vi "TC.vi"() -> ()   [LabVIEW 2013]
uses:
  lib/Lib.llb/CS.lvclass
  lib/Lib.llb/TCS.lvclass
  lib/Lib.llb/QCS.lvclass
  lib/Lib.llb/CS Emulation.lvclass
  lib/Lib.llb/PCS.lvclass
panel:
  out "TempStabilized":refnum<user-event>
  out "All I":dbl[](array[numeric])
  out "VI called?":bool=TRUE
  out "Error code":u8
  out "UpdateChannelInfo":refnum<user-event>
  out "zBridge set nr.":u8
  out "zDll":path=path "C:/Users/Sasha/Dropbox/Labview/LC Software/ImpSoft-V5.2.2-multithreaded/ImpBridgeLabview/ImpBridgeDll.dll"
  in  "String":string="^ Click the Run button to start the program "
  in  "Tab Control 6":enum32{"Page 1", "Page 2"}(tab)
  in  "Load config":bool
  in  "Start":bool
  in  "Load Data":bool
  in  "Pause":bool
  in  "Stop":bool
  in  "Minimize":bool
  in  "Copy to Clipboard":bool
  in  "Save to Cal Log":bool
  in  "Save config":bool
  in  "Save Data":bool
  in  "Clear all plots":bool
  in  "LogFileCreationTime":timestamp=timestamp(2742897600 s since 1904-01-01)
  out "UpdateLogFilePath":refnum<user-event>
  out "Calib path":path=path "C:/avs-47/aaaa"
  out "Log path":path
  out "TCS port":i32(ring)=3 items=["COM1", "COM2", "COM3", "COM4", "COM5", "COM6", "COM7", "COM8", "COM9", "PRN1", "PRN2", "PRN3", "PRN4"]
  out "UpdateCalibrations":refnum<user-event>
  out "AVS VISA session":refnum<visa-resource-name>="COM3"
  out "Current1flow":bool
  out "Current2flow":bool
  in  "Tab Control":enum32{"AVS"}(tab)
  in  "Channel Controls":T1(tab)=enum."All"
  out "T 01":dbl=nan caption="T" format="%#.3f mK"
  out "R 0":dbl caption="R" format="%.3p"
  out "R-Plot 0":cluster{dbl[], dbl[]}(graph) caption="R-Plot"
  in  "Log 0":bool caption="Log Y"
  out "T 02":dbl=nan caption="T" format="%#.3f mK"
  out "R 1":dbl caption="R" format="%.3p"
  out "R-Plot 1":cluster{dbl[], dbl[]}(graph) caption="R-Plot"
  in  "Log 1":bool caption="Log Y"
  out "T 03":dbl=nan caption="T" format="%#.3f mK"
  out "R 2":dbl caption="R" format="%.3p"
  out "R-Plot 2":cluster{dbl[], dbl[]}(graph) caption="R-Plot"
  in  "Log 2":bool caption="Log Y"
  out "T 04":dbl=nan caption="T" format="%#.3f mK"
  out "R 3":dbl caption="R" format="%.3p"
  out "R-Plot 3":cluster{dbl[], dbl[]}(graph) caption="R-Plot"
  in  "Log 3":bool caption="Log Y"
  out "T 05":dbl=nan caption="T" format="%#.3f mK"
  out "R 4":dbl caption="R" format="%.3p"
  out "R-Plot 4":cluster{dbl[], dbl[]}(graph) caption="R-Plot"
  in  "Log 4":bool caption="Log Y"
  out "T 06":dbl=nan caption="T" format="%#.3f mK"
  out "R 5":dbl caption="R" format="%.3p"
  out "R-Plot 5":cluster{dbl[], dbl[]}(graph) caption="R-Plot"
  in  "Log 5":bool caption="Log Y"
  out "T 07":dbl=nan caption="T" format="%#.3f mK"
  out "R 6":dbl caption="R" format="%.3p"
  out "R-Plot 6":cluster{dbl[], dbl[]}(graph) caption="R-Plot"
  in  "Log 6":bool caption="Log Y"
  out "T 08":dbl=nan caption="T" format="%#.3f mK"
  out "R 7":dbl caption="R" format="%.3p"
  out "R-Plot 7":cluster{dbl[], dbl[]}(graph) caption="R-Plot"
  in  "Log 7":bool caption="Log Y"
  out "T 9":dbl=nan caption="T" format="%#.3f mK"
  out "R 8":dbl caption="R" format="%.3p"
  out "R-Plot 8":cluster{dbl[], dbl[]}(graph) caption="R-Plot"
  in  "Log 8":bool caption="Log Y"
  out "T 10":dbl=nan caption="T" format="%#.3f mK"
  out "R 9":dbl caption="R" format="%.3p"
  out "R-Plot 9":cluster{dbl[], dbl[]}(graph) caption="R-Plot"
  in  "Log 9":bool caption="Log Y"
  out "T":T2 {"T0 3" format="%.2p"; "T0 2" format="%.2p"; "T0" format="%.2p"; "T0" format="%.2p"; "T0" format="%.2p"; "T0" format="%.2p"; "T0" format="%.2p"; "T0" format="%.2p"; "T0" format="%.2p"; "T0" format="%.2p"}
  in  "AVS names":T3={"AVS Name 0"="3K", "AVS Name 1"="Still", "AVS Name 2"="50 mK", "AVS Name 3"="MC", "AVS Name 4"="MC", "AVS Name 5"="", "AVS Name 6"="", "AVS Name 7"="", "AVS Name 8"="", "AVS Name 9"=""}
  in  "Edit Calibrations":T4
  in  "Thermometer":T5 {"Select sensor 10" items=["No Calibration.vi"]; "Select sensor 9" items=["No Calibration.vi"]; "Select sensor 8" items=["No Calibration.vi"]; "Select sensor 7" items=["No Calibration.vi"]; "Select sensor 6" items=["No Calibration.vi"]; "Select sensor 5" items=["No Calibration.vi"]; "Select sensor 4" items=["No Calibration.vi"]; "Select sensor 3" items=["No Calibration.vi"]; "Select sensor 2" items=["No Calibration.vi"]; "Select sensor 1" items=["No Calibration.vi"]}
  out "Units":T3
  out "R":T6={"R0"=0.0, "R1"=0.0, "R2"=-0.0, "R3"=0.0, "R4"=0.0, "R5"=0.0, "R6"=0.0, "R7"=0.0, "R6 2"=0.0, "R7 2"=0.0} {"R7 2" format="%.3p"; "R6 2" format="%.3p"; "R7" format="%.3p"; "R6" format="%.3p"; "R5" format="%.3p"; "R4" format="%.3p"; "R3" format="%.3p"; "R2" format="%.3p"; "R1" format="%.3p"; "R0" format="%.3p"}
  in  "Scan Parameters":enum32{"Page 1", "Page 2"}(tab)
  in  "Exc&Ranges":T7={"Excitationl 0"=4, "Excitationl 0"=4, "Excitationl 0"=3, "Excitationl 0"=3, "Excitationl 0"=3, "Excitationl 0"=3, "Excitationl 0"=3, "Excitationl 0"=3, "Range 0"=5, "Range 0"=5, "Range 0"=5, "Range 0"=5, "Range 0"=5, "Range 0"=5, "Range 0"=5, "Range 0"=5} {"Range 0" items=["n.a."=-1, "open"=0, "2 Ohm"=1, "20 Ohm"=2, "200 Ohm"=3, "2k Ohm"=4, "20k Ohm"=5, "200k Ohm"=6, "2M Ohm"=7]; "Range 0" items=["n.a."=-1, "open"=0, "2 Ohm"=1, "20 Ohm"=2, "200 Ohm"=3, "2k Ohm"=4, "20k Ohm"=5, "200k Ohm"=6, "2M Ohm"=7]; "Range 0" items=["n.a."=-1, "open"=0, "2 Ohm"=1, "20 Ohm"=2, "200 Ohm"=3, "2k Ohm"=4, "20k Ohm"=5, "200k Ohm"=6, "2M Ohm"=7]; "Range 0" items=["n.a."=-1, "open"=0, "2 Ohm"=1, "20 Ohm"=2, "200 Ohm"=3, "2k Ohm"=4, "20k Ohm"=5, "200k Ohm"=6, "2M Ohm"=7]; "Range 0" items=["n.a."=-1, "open"=0, "2 Ohm"=1, "20 Ohm"=2, "200 Ohm"=3, "2k Ohm"=4, "20k Ohm"=5, "200k Ohm"=6, "2M Ohm"=7]; "Range 0" items=["n.a."=-1, "open"=0, "2 Ohm"=1, "20 Ohm"=2, "200 Ohm"=3, "2k Ohm"=4, "20k Ohm"=5, "200k Ohm"=6, "2M Ohm"=7]; "Range 0" items=["n.a."=-1, "open"=0, "2 Ohm"=1, "20 Ohm"=2, "200 Ohm"=3, "2k Ohm"=4, "20k Ohm"=5, "200k Ohm"=6, "2M Ohm"=7]; "Range 0" items=["n.a."=-1, "open"=0, "2 Ohm"=1, "20 Ohm"=2, "200 Ohm"=3, "2k Ohm"=4, "20k Ohm"=5, "200k Ohm"=6, "2M Ohm"=7]; "Excitationl 0" items=["none", "3 µV", "10 µV", "30 µV", "100 µV", "300 µV", "1 mV", "3 mV"]; "Excitationl 0" items=["none", "3 µV", "10 µV", "30 µV", "100 µV", "300 µV", "1 mV", "3 mV"]; "Excitationl 0" items=["none", "3 µV", "10 µV", "30 µV", "100 µV", "300 µV", "1 mV", "3 mV"]; "Excitationl 0" items=["none", "3 µV", "10 µV", "30 µV", "100 µV", "300 µV", "1 mV", "3 mV"]; "Excitationl 0" items=["none", "3 µV", "10 µV", "30 µV", "100 µV", "300 µV", "1 mV", "3 mV"]; "Excitationl 0" items=["none", "3 µV", "10 µV", "30 µV", "100 µV", "300 µV", "1 mV", "3 mV"]; "Excitationl 0" items=["none", "3 µV", "10 µV", "30 µV", "100 µV", "300 µV", "1 mV", "3 mV"]; "Excitationl 0" items=["none", "3 µV", "10 µV", "30 µV", "100 µV", "300 µV", "1 mV", "3 mV"]}
  out "Status":T8
  out "zBridge params":T3
  out "uPlots":T9
  in  "Autorange":bool=TRUE
  out "Active":T10={"active Channel 0"=TRUE, "active Channel 1"=TRUE, "active Channel 2"=TRUE, "active Channel 3"=FALSE, "active Channel 4"=FALSE, "active Channel 5"=FALSE, "active Channel 6"=FALSE, "active Channel 7"=FALSE, "active Channel 8"=FALSE, "active Channel 9"=FALSE}
  out "SP":cluster{"Numeric":dbl, "R/T":dbl}(graph) caption="R-Plot 10"
  in  "HW Address":u32
  in  "Edit calibration":bool
  in  "Convert":bool
  out "T7":dbl caption="T=" format="%#.2p"
  in  "R7":dbl caption="R=" format="%_6g"
  in  "Select sensor 1":u16(ring) items=["No Calibration.vi"]
  out "I_list[i]":dbl[](array[numeric]) min=-1.0
  out "I 2":dbl[](array[numeric]) min=-1.0
  out "Revision":string="TC" caption="V"
  in  "Tab Control 5":enum32{"Page 1", "Page 2"}(tab)
  in  "Data History":enum32{"History", "Settings"}(tab)=enum."Settings"
  in  "Mode Buttons":T11(radio)
  in  "Clear plot":bool
  out "AVS names small":T3={"AVS Name 0"="3K", "AVS Name 1"="Still", "AVS Name 2"="50 mK", "AVS Name 3"="MC", "AVS Name 4"="MC", "AVS Name 5"="", "AVS Name 6"="", "AVS Name 7"="", "AVS Name 8"="", "AVS Name 9"=""}
  out "Time":dbl format="%<%X\n%x>T"
  out "Small T":dbl[](array[numeric]) caption="T" format="%.2p"
  out "Small R":dbl[](array[numeric]) caption="R" format="%.3p"
  in  "AVS Runtime Settings":T12={"Read AVS channels from"=0, "Last Channel"=4, "Delay Between Scans"=0, "Stabilisation Delay"=0.5, "Averages"=2, "Data Memory"=5000, "Filter graphs:"=FALSE, "Y_min"=0.0, "Y_max"=2000000.0, "Plot type"=enum."T vs Time", "Boolean"=FALSE, "Data Memory 2"=30.0} {"Data Memory 2" min=0.0; "Delay Between Scans" format="%.0f s"; "Averages" min=1 max=1000; "Stabilisation Delay" min=0.5; "Last Channel" min=0 max=9 step=1; "Read AVS channels from" min=0 max=7 step=1; "Y_max" format="%#_6f"; "Y_min" min=0.0 format="%#_6f"; "Data Memory" min=3 max=20000}
  out "I":dbl[](array[numeric])
  in  "Data":cluster{"R":dbl[], "T":dbl[], "Time":dbl[]}[](array[cluster])=[{"R"=[], "T"=[], "Time"=[]}, {"R"=[0.0, 2.0], "T"=[], "Time"=[]}]
  out "Int":dbl=10.0 format="%#.2f"
  out "T_array":dbl[](array[numeric])
  in  "Data array":dbl[](array[numeric])
  out "I3_SetPnt":dbl
  out "Currents changed":bool
  in  "Excitations":T13={"Excitationl 0"=4, "Excitation 1"=4, "Excitation 2"=3, "Excitation 3"=3, "Excitation 4"=3, "Excitation 5"=3, "Excitation 6"=3, "Excitation 7"=3} {"Excitation 7" items=["none", "3 µV", "10 µV", "30 µV", "100 µV", "300 µV", "1 mV", "3 mV"]; "Excitation 6" items=["none", "3 µV", "10 µV", "30 µV", "100 µV", "300 µV", "1 mV", "3 mV"]; "Excitation 5" items=["none", "3 µV", "10 µV", "30 µV", "100 µV", "300 µV", "1 mV", "3 mV"]; "Excitation 4" items=["none", "3 µV", "10 µV", "30 µV", "100 µV", "300 µV", "1 mV", "3 mV"]; "Excitation 3" items=["none", "3 µV", "10 µV", "30 µV", "100 µV", "300 µV", "1 mV", "3 mV"]; "Excitation 2" items=["none", "3 µV", "10 µV", "30 µV", "100 µV", "300 µV", "1 mV", "3 mV"]; "Excitation 1" items=["none", "3 µV", "10 µV", "30 µV", "100 µV", "300 µV", "1 mV", "3 mV"]; "Excitationl 0" items=["none", "3 µV", "10 µV", "30 µV", "100 µV", "300 µV", "1 mV", "3 mV"]}
  in  "Ranges":T13={"Excitationl 0"=5, "Excitation 1"=5, "Excitation 2"=5, "Excitation 3"=5, "Excitation 4"=5, "Excitation 5"=5, "Excitation 6"=5, "Excitation 7"=5} {"Excitation 7" items=["n.a."=-1, "open"=0, "2 Ohm"=1, "20 Ohm"=2, "200 Ohm"=3, "2k Ohm"=4, "20k Ohm"=5, "200k Ohm"=6, "2M Ohm"=7]; "Excitation 6" items=["n.a."=-1, "open"=0, "2 Ohm"=1, "20 Ohm"=2, "200 Ohm"=3, "2k Ohm"=4, "20k Ohm"=5, "200k Ohm"=6, "2M Ohm"=7]; "Excitation 5" items=["n.a."=-1, "open"=0, "2 Ohm"=1, "20 Ohm"=2, "200 Ohm"=3, "2k Ohm"=4, "20k Ohm"=5, "200k Ohm"=6, "2M Ohm"=7]; "Excitation 4" items=["n.a."=-1, "open"=0, "2 Ohm"=1, "20 Ohm"=2, "200 Ohm"=3, "2k Ohm"=4, "20k Ohm"=5, "200k Ohm"=6, "2M Ohm"=7]; "Excitation 3" items=["n.a."=-1, "open"=0, "2 Ohm"=1, "20 Ohm"=2, "200 Ohm"=3, "2k Ohm"=4, "20k Ohm"=5, "200k Ohm"=6, "2M Ohm"=7]; "Excitation 2" items=["n.a."=-1, "open"=0, "2 Ohm"=1, "20 Ohm"=2, "200 Ohm"=3, "2k Ohm"=4, "20k Ohm"=5, "200k Ohm"=6, "2M Ohm"=7]; "Excitation 1" items=["n.a."=-1, "open"=0, "2 Ohm"=1, "20 Ohm"=2, "200 Ohm"=3, "2k Ohm"=4, "20k Ohm"=5, "200k Ohm"=6, "2M Ohm"=7]; "Excitationl 0" items=["n.a."=-1, "open"=0, "2 Ohm"=1, "20 Ohm"=2, "200 Ohm"=3, "2k Ohm"=4, "20k Ohm"=5, "200k Ohm"=6, "2M Ohm"=7]}
  out "CS ref":refnum<class "CS.lvclass">
  out "start 2":bool
  in  "Tab Control 3":enum32{"Page 1", "Page 2"}(tab)
  out "Automatic mode 0":bool
  out "Automatic mode 1":bool
  out "Map Channel 0 to 2":T14(ring) caption="Output to"
  in  "uA 0":u32
  in  "CS Names":T15={"CS Name 0"="N.C.", "CS Name 1"="3K", "CS Name 2"="Still", "CS Name 3"="MC"}
  out "Ch0 -":T16={"uA"="000", "ON"=FALSE, "Gated"=FALSE, "current flows"=FALSE, "Error"=FALSE}
  in  "uA 3":u32
  in  "uA 2":u32
  in  "uA 1":u32
  out "Automatic mode 3":bool
  out "Automatic mode 2":bool
  out "Chn 3":T16={"uA"="000", "ON"=FALSE, "Gated"=FALSE, "current flows"=FALSE, "Error"=FALSE}
  out "Chn 2":T16={"uA"="000", "ON"=FALSE, "Gated"=FALSE, "current flows"=FALSE, "Error"=FALSE}
  out "Chn 1":T16={"uA"="000", "ON"=FALSE, "Gated"=FALSE, "current flows"=FALSE, "Error"=FALSE}
  out "I3":dbl=10.0
  out "vi reference":refnum<vi>
  in  "CS Ch3 mode":enum32{"Page 1", "Page 2"}(tab)=enum."Page 2"
  in  "T Sweep":T17={"Start value"=200.0, "End value"=250.0, "Step"=10.0, "Current"=0.0, "I_next"=FALSE, "I_prev"=FALSE, "Interrrupt Sweep"=FALSE, "Start"=FALSE, "Boolean"=TRUE} {"Step" min=0.0; "End value" min=0.0; "Start value" min=0.0}
  in  "Show PID graph?":bool
  out "I0":dbl format="%#.1f"
  out "CallExtVI":refnum<user-event>
  out "Unit":string
  out "UpdateValuesAVS":refnum<user-event>
  out "DoPID":refnum<user-event>
  out "UpdateValuesZBridge":refnum<user-event>
  out "zBridge params/Error":string
  out "CurCalibrations":T18
  out "LMB Down":bool
  out "T controlled":dbl
  out "ResetPIDloop":refnum<user-event>
  in  "Tab Control 2":T19(tab)
  in  "Parameters":bool
  out "ID":string
  out "Bridge status":errorcluster
  out "CS status":errorcluster
  out "General":errorcluster caption="General status"
  in  "Refresh Button":bool
  in  "Bridge settings":T20={"AVS type"=enum."AVS47A (GPIB interface)", "AVS_SPort"="COM5", "Address"="GPIB0::20::INSTR", "AVS_CalFolder"=path "E:/Dropbox/Labview/LC Software/All Calibrations"}
  in  "Current source settings":T21={"TCS_Port"="COM1", "TCS_Imax"=5, "CS type"=enum."TCS", "QCS/PCS Device"=0}
  in  "Data logging":T22={"AVS_Path"=path "C:/avs-47", "AVS_FName"="LogAVS", "CAL_FName"="calibration", "Filenames suffix"="_%Y-%m-%d-%H-%M-%S", "Delimeter"="\t", "NewFevery"=7, "Time Units"=enum."Days", "Date/Time Format"="%Y-%m-%d %H:%M:%S", "External VI path"=path "C:/Users/User1/Dropbox/Labview/LC Software/TempControl/OnTempStabilized Ext VI Laurens.vi", "VI state:"=enum."Bad", "Ask on start?"=FALSE, "Run description"="\n"}
  in  "I_Clear":bool
  in  "I3 as temp":cluster{"I3 as temp 2":bool}
  in  "I3":T23={"Toggle ON/OFF"=FALSE, "Toggle Gated"=FALSE, "I"=0, "Range"=enum."x1 uA"} {"I" max=100000 step=1}
  in  "I2":T23={"Toggle ON/OFF"=FALSE, "Toggle Gated"=FALSE, "I"=0, "Range"=enum."x1 uA"} {"I" max=100000 step=1}
  in  "I1":T23={"Toggle ON/OFF"=FALSE, "Toggle Gated"=FALSE, "I"=0, "Range"=enum."x1 uA"} {"I" max=100000 step=1}
  in  "I0":T23={"Toggle ON/OFF"=FALSE, "Toggle Gated"=FALSE, "I"=0, "Range"=enum."x1 uA"} {"I" max=100000 step=1}
  in  "Set QCS Channel 0 output to":T24(ring) caption="Output to"
  in  "Mode":enum16{"Manual", "Automatic"}(ring) caption="CS control mode"
  in  "Write to log":bool
  in  "Load from file":bool
  in  "Save to file":bool
  in  "I_tofirst":bool
  in  "I_next":bool
  in  "I_prev":bool
  out "VI state:":T25(ring)
  in  "Call external VI":bool
  out "Time Old":dbl format="%#_16g"
  in  "I_list":dbl[][](array[numeric]) min=-1.0
  out "I_selection":bool[](array[boolean])=[TRUE, FALSE, FALSE, FALSE, FALSE, FALSE, FALSE, FALSE, FALSE, FALSE]
  in  "Automode Settings 2":T26={"AVS Channel"=0, "N averages"=10, "Delay Time"=10.0, "T stability"=0.3, "FB on"=enum."Temperature"} {"Delay Time" min=0.0 format="%#_g min"; "AVS Channel" min=-1 max=9 step=1}
  in  "Automode 2":bool=TRUE caption="Enable automatic sweeping/list iteration"
  in  "PID setup 2":T27={"Current limit, [uA]"=10000.0, "Proportional Gain"=3.0, "Integral Gain"=3.0, "Derivative Gain"=1.0, "SP tolerance"=0.1, "Feed Fwd Gain [uA/mK]"=0.0, "Integral Gain Bandwidth"=10.0, "Integral Gain Background"=1.0, "FB on 2"=enum."1"} {"Integral Gain Background" format="%#.6g"; "Integral Gain Bandwidth" format="%#.6g"; "Feed Fwd Gain [uA/mK]" format="%#.5g"; "SP tolerance" format="%#.5g"; "Derivative Gain" format="%#.6g"; "Integral Gain" format="%#.6g"; "Proportional Gain" format="%#.6g"; "Current limit, [uA]" format="%#.5g"}
  in  "Reset PID":bool
  in  "Next step":bool
  out "I_list_idx":i32=10 caption="Point #"
  out "I_list_idx_max":i32=10 caption="of"
  out "Timer":dbl format="%<%H:%M:%S>t"
  out "Slope":dbl format="%#_3g %"
  out "Error":dbl=10.0 format="%#_6f"
  out "SP reached?":bool
  # "Quick convert R->T:"
  # "Ohm"
  # "mK"
  # "Ch#"
  # "Miniplot"
  # "Channel parameters"
  # "Impedance"
  # "Unit"
  # "Type of sensor"
  # "T [mK]"
  # "Description"
  # "0"
  # "1"
  # "2"
  # "3"
  # "4"
  # "5"
  # "6"
  # "7"
  # "8"
  # "9"
  # "0"
  # "1"
  # "2"
  # "3"
  # "4"
  # "5"
  # "7"
  # "8"
  # "9"
  # "6"
  # "auto"
  # "auto"
  # "auto"
  # "auto"
  # "gated"
  # "gated"
  # "gated"
  # "gated"
  # "Ch3"
  # "Current source mode"
  # "Current source manual control"
  # "Automatic mode or current source"
  # "Currents List"
  # "Settings"
  # "I0"
  # "I1"
  # "I2"
  # "I3"
  # "Status"
  # "On temperature stabilized"
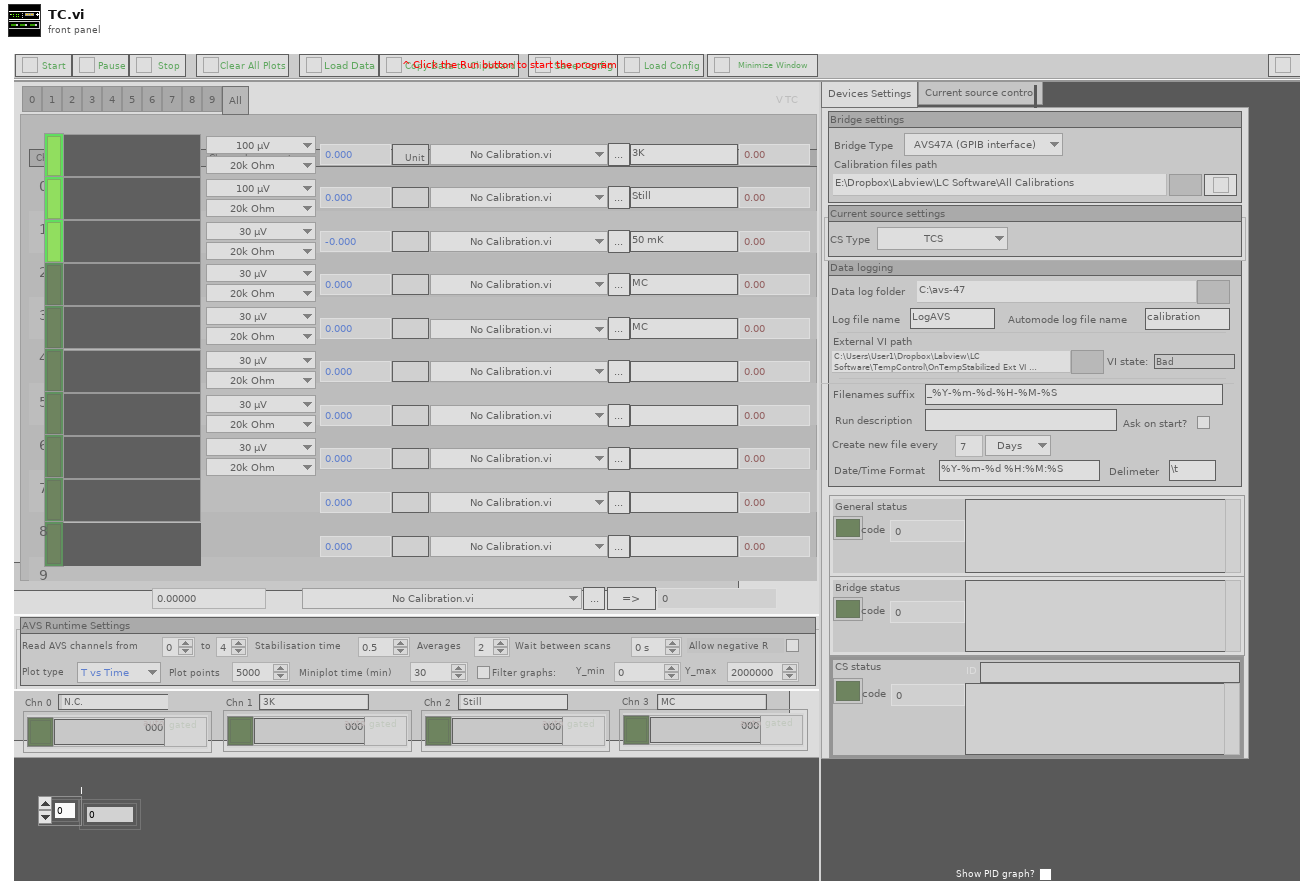
[diagram p1: front panel]
types:
  T1 = enum32{"0", "1", "2", "3", "4", "5", "6", "7", "8", "9", "All", "PID loop"}
  T2 = cluster{"T0":dbl, "T0":dbl, "T0":dbl, "T0":dbl, "T0":dbl, "T0":dbl, "T0":dbl, "T0":dbl, "T0 2":dbl, "T0 3":dbl}
  T3 = cluster{"AVS Name 0":string, "AVS Name 1":string, "AVS Name 2":string, "AVS Name 3":string, "AVS Name 4":string, "AVS Name 5":string, "AVS Name 6":string, "AVS Name 7":string, "AVS Name 8":string, "AVS Name 9":string}
  T4 = cluster{"Boolean":bool, "Boolean 2":bool, "Boolean 3":bool, "Boolean 4":bool, "Boolean 5":bool, "Boolean 6":bool, "Boolean 7":bool, "Boolean 8":bool, "Boolean 9":bool, "Boolean 10":bool}
  T5 = cluster{"Select sensor 1":u16, "Select sensor 2":u16, "Select sensor 3":u16, "Select sensor 4":u16, "Select sensor 5":u16, "Select sensor 6":u16, "Select sensor 7":u16, "Select sensor 8":u16, "Select sensor 9":u16, "Select sensor 10":u16}
  T6 = cluster{"R0":dbl, "R1":dbl, "R2":dbl, "R3":dbl, "R4":dbl, "R5":dbl, "R6":dbl, "R7":dbl, "R6 2":dbl, "R7 2":dbl}
  T7 = cluster{"Excitationl 0":i16, "Excitationl 0":i16, "Excitationl 0":i16, "Excitationl 0":i16, "Excitationl 0":i16, "Excitationl 0":i16, "Excitationl 0":i16, "Excitationl 0":i16, "Range 0":i16, "Range 0":i16, "Range 0":i16, "Range 0":i16, "Range 0":i16, "Range 0":i16, "Range 0":i16, "Range 0":i16}
  T8 = cluster{"Numeric":dbl, "Numeric":dbl, "Numeric":dbl, "Numeric":dbl, "Numeric":dbl, "Numeric":dbl, "Numeric":dbl, "Numeric":dbl, "Numeric":dbl, "Numeric":dbl}
  T9 = cluster{"uPlot 0":cluster{dbl[], dbl[]}, "uPlot 1":cluster{dbl[], dbl[]}, "uPlot 2":cluster{dbl[], dbl[]}, "uPlot 3":cluster{dbl[], dbl[]}, "uPlot 4":cluster{dbl[], dbl[]}, "uPlot 5":cluster{dbl[], dbl[]}, "uPlot 6":cluster{dbl[], dbl[]}, "uPlot 7":cluster{dbl[], dbl[]}, "uPlot 8":cluster{dbl[], dbl[]}, "uPlot 9":cluster{dbl[], dbl[]}}
  T10 = cluster{"active Channel 0":bool, "active Channel 1":bool, "active Channel 2":bool, "active Channel 3":bool, "active Channel 4":bool, "active Channel 5":bool, "active Channel 6":bool, "active Channel 7":bool, "active Channel 8":bool, "active Channel 9":bool}
  T11 = enum32{"No Selection", "Cursor Mode", "Erase point", "Erase Range"}
  T12 = cluster{"Read AVS channels from":i8, "Last Channel":i8, "Delay Between Scans":u32, "Stabilisation Delay":dbl, "Averages":u16, "Data Memory":u16, "Filter graphs:":bool, "Y_min":dbl, "Y_max":dbl, "Plot type":enum16{"R vs Time", "T vs Time"}, "Boolean":bool, "Data Memory 2":dbl}
  T13 = cluster{"Excitationl 0":i16, "Excitation 1":i16, "Excitation 2":i16, "Excitation 3":i16, "Excitation 4":i16, "Excitation 5":i16, "Excitation 6":i16, "Excitation 7":i16}
  T14 = enum16{"Chn 0", "Aux 0", "Aux 1", "Aux 2", "Aux 3"}
  T15 = cluster{"CS Name 0":string, "CS Name 1":string, "CS Name 2":string, "CS Name 3":string}
  T16 = cluster{"uA":string, "ON":bool, "Gated":bool, "current flows":bool, "Error":bool}
  T17 = cluster{"Start value":dbl, "End value":dbl, "Step":dbl, "Current":dbl, "I_next":bool, "I_prev":bool, "Interrrupt Sweep":bool, "Start":bool, "Boolean":bool}
  T18 = cluster{"[0]":string, "[1]":string, "[2]":string, "[3]":string, "[4]":string, "[5]":string, "[6]":string, "[7]":string, "[8]":string, "[9]":string}
  T19 = enum32{"Devices Settings", "Current source control"}
  T20 = cluster{"AVS type":enum16{"AVS47A (GPIB interface)", "AVS47B (RS232 interface)", "AVS Emulation", "Impedance Bridge", "Disabled"}, "AVS_SPort":refnum<visa-resource-name>, "Address":refnum<visa-resource-name>, "AVS_CalFolder":path}
  T21 = cluster{"TCS_Port":refnum<visa-resource-name>, "TCS_Imax":i32, "CS type":enum16{"TCS", "QCS v1", "PCS (n.a.)", "CS Emulation", "Disabled"}, "QCS/PCS Device":u16}
  T22 = cluster{"AVS_Path":path, "AVS_FName":string, "CAL_FName":string, "Filenames suffix":string, "Delimeter":string, "NewFevery":u32, "Time Units":enum16{"Minutes", "Hours", "Days"}, "Date/Time Format":string, "External VI path":path, "VI state:":enum32{"Bad", "Idle", "Run top level", "Running"}, "Ask on start?":bool, "Run description":string}
  T23 = cluster{"Toggle ON/OFF":bool, "Toggle Gated":bool, "I":u32, "Range":enum8{"Auto", "x1 uA", "x10 uA", "x100 uA", "x1 mA"}}
  T24 = enum16{"Channel 0", "Aux 0", "Aux 1", "Aux 2", "Aux 3"}
  T25 = enum32{"Bad", "Idle", "Run top level", "Running"}
  T26 = cluster{"AVS Channel":i32, "N averages":i32, "Delay Time":dbl, "T stability":dbl, "FB on":enum16{"Resistance", "Temperature"}}
  T27 = cluster{"Current limit, [uA]":dbl, "Proportional Gain":dbl, "Integral Gain":dbl, "Derivative Gain":dbl, "SP tolerance":dbl, "Feed Fwd Gain [uA/mK]":dbl, "Integral Gain Bandwidth":dbl, "Integral Gain Background":dbl, "FB on 2":enum16{"0", "1", "2", "3"}}
  T28 = cluster{"error":bool, "code":i32, "source":string}
  T29 = enum32{"No Selection", "Erase Data", "Erase Range", "Cursor Mode"}
  T30 = enum16{"AVS47A (GPIB interface)", "AVS47B (RS232 interface)", "AVS Emulation", "Impedance Bridge", "Disabled"}
  T31 = enum16{"TCS", "QCS v1", "PCS (n.a.)", "CS Emulation", "Disabled"}
  T32 = enum8{"Auto", "x1 uA", "x10 uA", "x100 uA", "x1 mA"}
  T33 = cluster{"Cluster":cluster{"Time":dbl[], "T":dbl[]}, "Cluster":cluster{"Time":dbl[], "T":dbl[]}, "Cluster":cluster{"Time":dbl[], "T":dbl[]}, "Cluster":cluster{"Time":dbl[], "T":dbl[]}, "Cluster":cluster{"Time":dbl[], "T":dbl[]}, "Cluster":cluster{"Time":dbl[], "T":dbl[]}, "Cluster":cluster{"Time":dbl[], "T":dbl[]}, "Cluster":cluster{"Time":dbl[], "T":dbl[]}, "Cluster":cluster{"Time":dbl[], "T":dbl[]}, "Cluster":cluster{"Time":dbl[], "T":dbl[]}}
  T34 = enum32{"HKEY_CLASSES_ROOT", "HKEY_CURRENT_USER", "HKEY_LOCAL_MACHINE", "HKEY_USERS", "HKEY_PERFORMANCE_DATA", "HKEY_CURRENT_CONFIG", "HKEY_DYN_DATA"}
  T35 = enum32{"invalid app kind", "Development System", "Run Time System", "Student Edition", "Embedded LabVIEW", "Evaluation", "Custom"}
  T36 = cluster{"[0]":dbl, "[1]":dbl, "[2]":dbl, "[3]":dbl, "[4]":dbl, "[5]":dbl, "[6]":dbl, "[7]":dbl, "[8]":dbl, "[9]":dbl}
  T37 = cluster{"Temperature[0]":dbl, "Temperature[1]":dbl, "Temperature[2]":dbl, "Temperature[3]":dbl, "Temperature[4]":dbl, "Temperature[5]":dbl, "Temperature[6]":dbl, "Temperature[7]":dbl, "Temperature[8]":dbl, "Temperature[9]":dbl}
  T38 = cluster{"type":string, "creator":string, "permissions":i32, "data size":i32, "res size":i32, "creation date":u32, "modification date":u32, "bFolder":bool, "bInvisible":bool, "location":cluster{"vertical":i16, "horizontal":i16}, "owner":string, "group":string}
  T39 = cluster{"Units[0]":string, "Units[1]":string, "Units[2]":string, "Units[3]":string, "Units[4]":string, "Units[5]":string, "Units[6]":string, "Units[7]":string, "Units[8]":string, "Units[9]":string}
  T40 = cluster{"zBridge params[0]":string, "zBridge params[1]":string, "zBridge params[2]":string, "zBridge params[3]":string, "zBridge params[4]":string, "zBridge params[5]":string, "zBridge params[6]":string, "zBridge params[7]":string, "zBridge params[8]":string, "zBridge params[9]":string}
  T41 = cluster{"date/time string":string, "Value":dbl[], "Value":dbl[], "Value":dbl[]}
  T42 = typedef "LVPoint32TypeDef.ctl" = cluster{"Horizontal":i32, "Vertical":i32}
  T43 = cluster{"Output Array":dbl[], "array w/ subset deleted":dbl[], "array w/ subset deleted":dbl[]}
  T44 = typedef "LVRectTypeDef.ctl" = cluster{"Left":i16, "Top":i16, "Right":i16, "Bottom":i16}
  T45 = cluster{"Excitationl 0":i16, "Excitation 1":i16, "Excitation 2":i16, "Excitation 3":i16, "Excitation 4":i16, "Excitation 5":i16, "Excitation 6":i16, "Excitation 7":i16, "Range 0":i16, "Range 1":i16, "Range 2":i16, "Range 3":i16, "Range 4":i16, "Range 5":i16, "Range 6":i16, "Range 7":i16}
  T46 = enum8{"Active", "Channel Type", "Channel No", "Reference No", "RLC select", "Save Data", "L Inverted", "Menu Active"}
  T47 = cluster{"Range 0":i16, "Range 1":i16, "Range 2":i16, "Range 3":i16, "Range 4":i16, "Range 7":i16, "Range 5":i16, "Range 6":i16}
  T48 = cluster{"Range 0":i16, "Range 1":i16, "Range 2":i16, "Range 3":i16, "Range 4":i16, "Range 5":i16, "Range 6":i16, "Range 7":i16}
  T49 = cluster{"RANGE 0":u16, "RANGE 1":u16, "RANGE 2":u16, "RANGE 3":u16, "RANGE 4":u16, "RANGE 5":u16, "RANGE 6":u16, "RANGE 7":u16}
  T50 = cluster{"Range":u8, "Current":dbl, "Current (string)":string, "On?":bool, "G?":bool, "I?":bool, "Err?":bool}
  T51 = cluster{"uA":string, " ON":bool, "Gated":bool, "current flows":bool, "Error":bool}
  T52 = cluster{"Toggle ON/OFF":bool, "Toggle Gated":bool}
  T53 = cluster{"Current":u32, "Range":enum16{"Auto", "x1 uA", "x10 uA", "x100 uA", "x1 mA"}}
  T54 = cluster{"Toggle ON/OFF":bool, "Toggle Gated":bool, "Current":u32, "Range":enum8{"Auto", "x1 uA", "x10 uA", "x100 uA", "x1 mA"}}
  T55 = cluster{"Status[0]":i32, "Status[1]":i32, "Status[2]":i32, "Status[3]":i32, "Status[4]":i32, "Status[5]":i32, "Status[6]":i32, "Status[7]":i32, "Status[8]":i32, "Status[9]":i32}
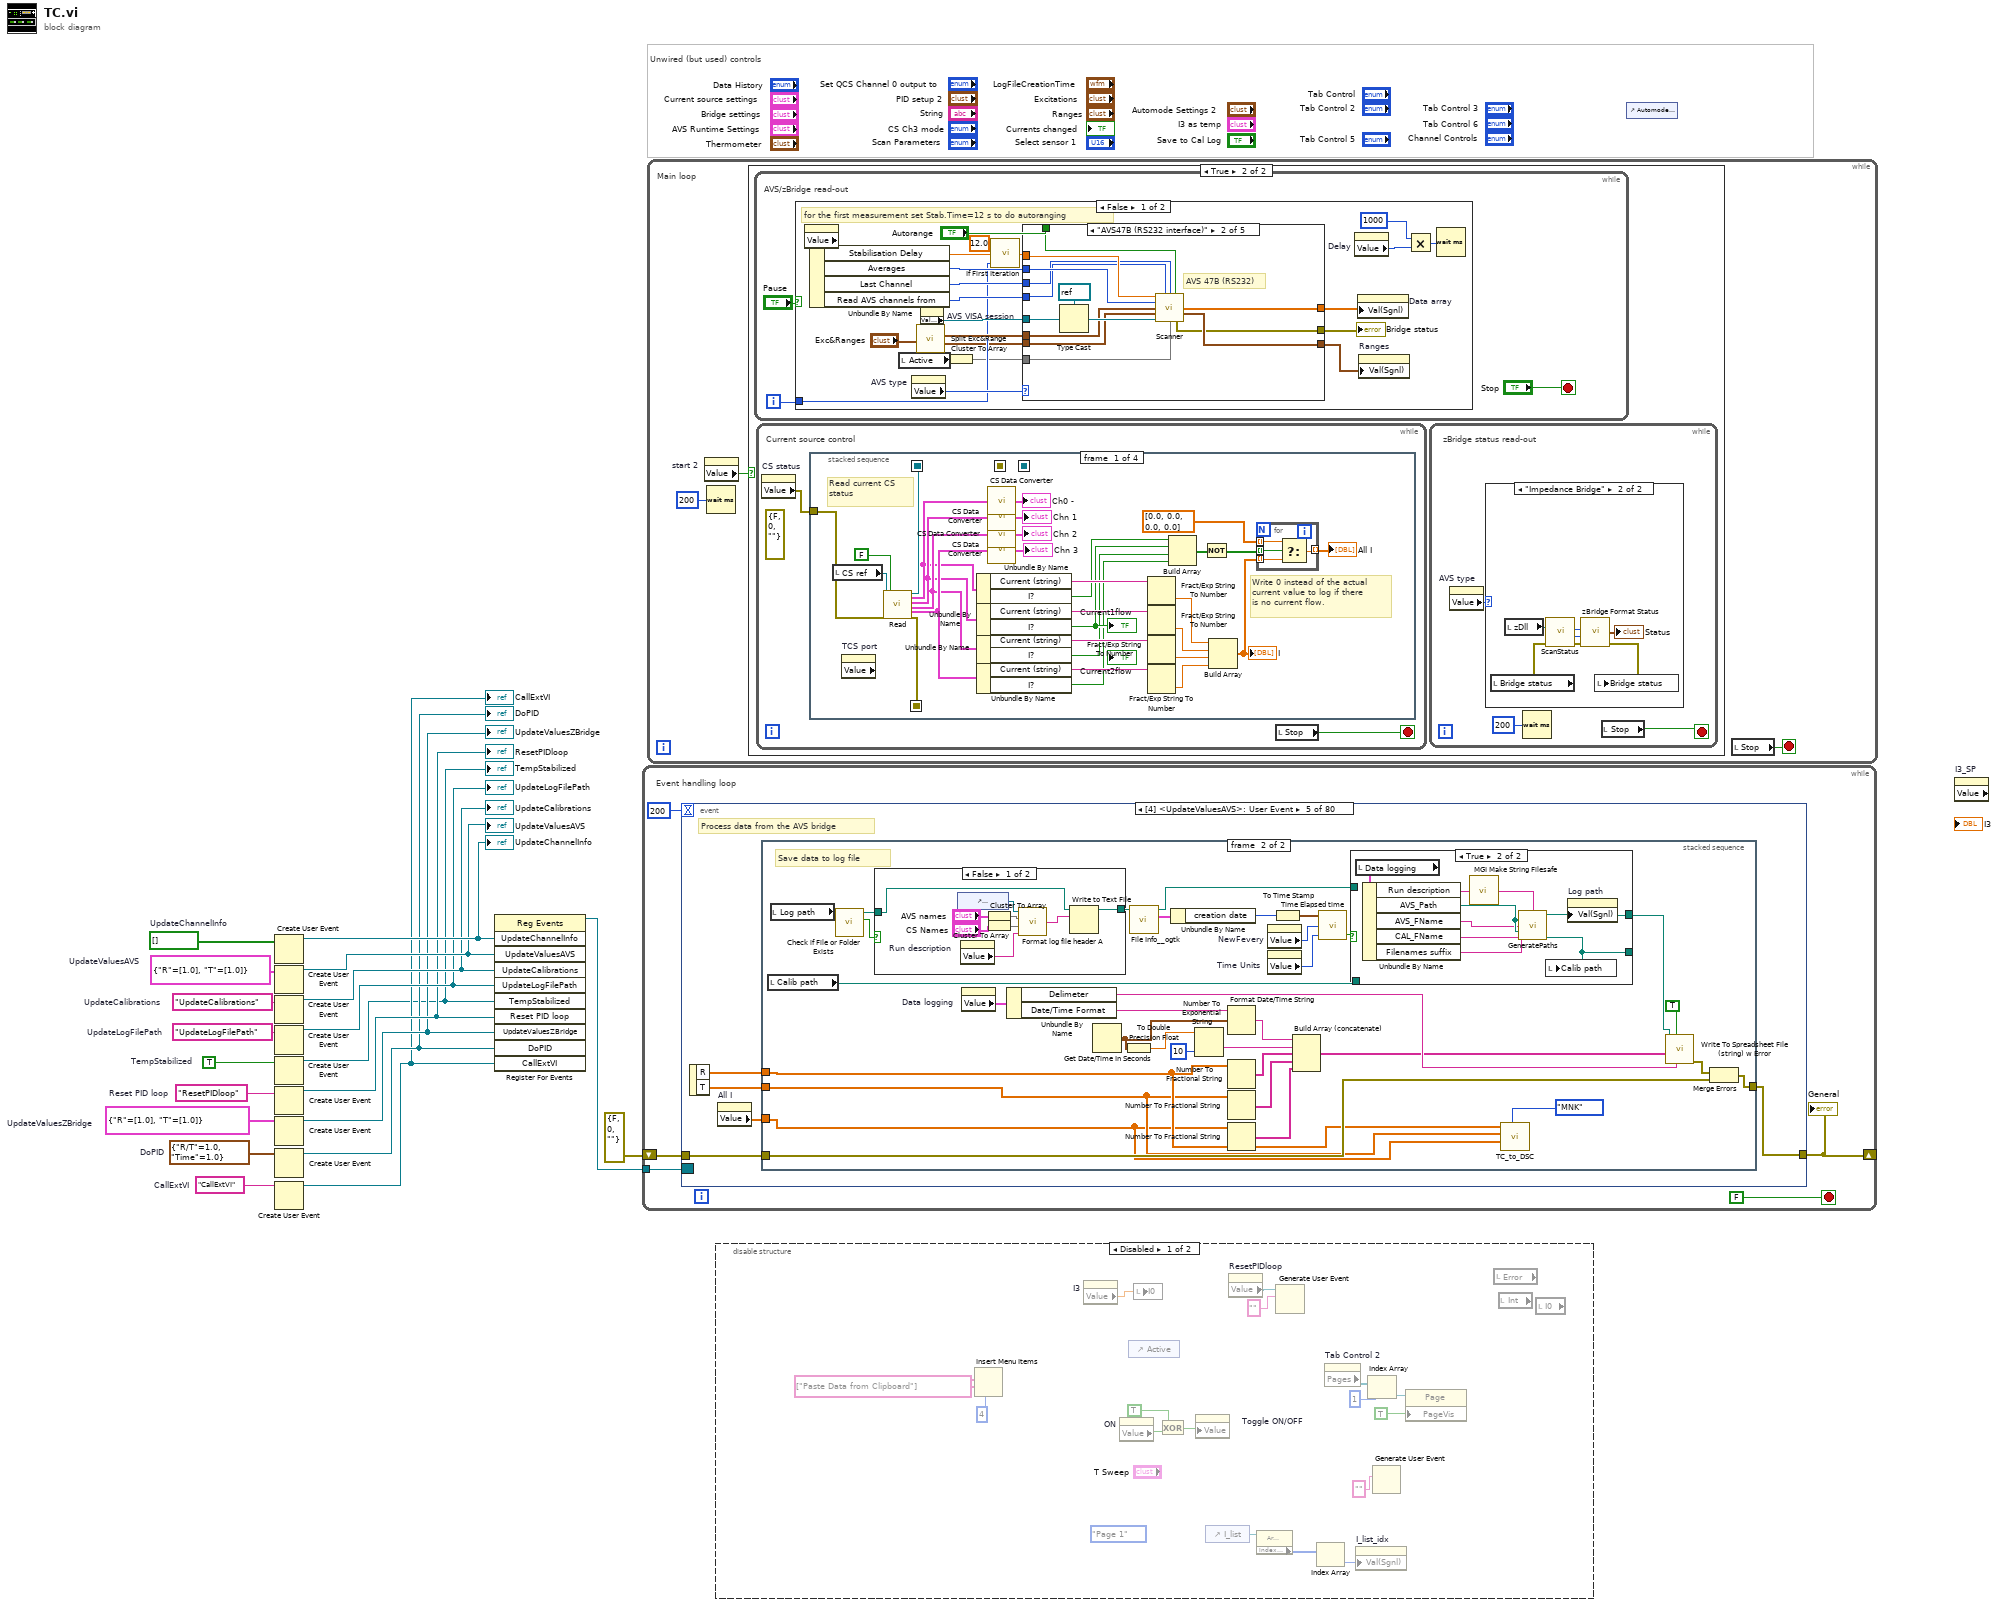
[diagram p0: block diagram]
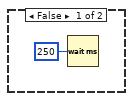
[diagram p3: hidden frame]
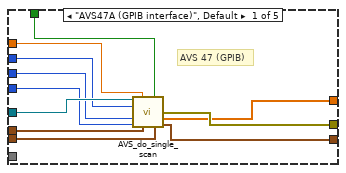
[diagram p5: hidden frame]
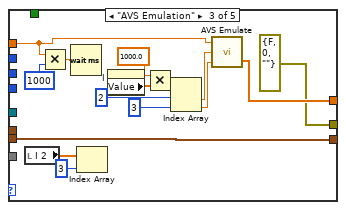
[diagram p6: hidden frame]
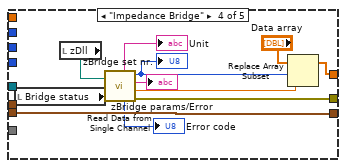
[diagram p7: hidden frame]
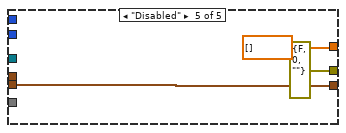
[diagram p8: hidden frame]
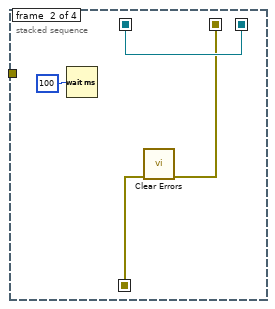
[diagram p10: hidden frame]
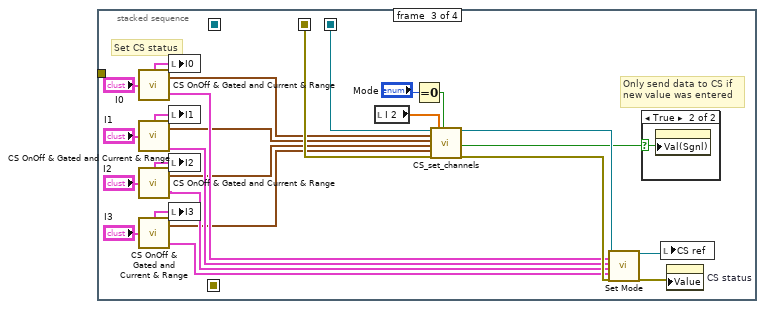
[diagram p11: hidden frame]
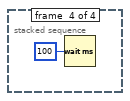
[diagram p13: hidden frame]
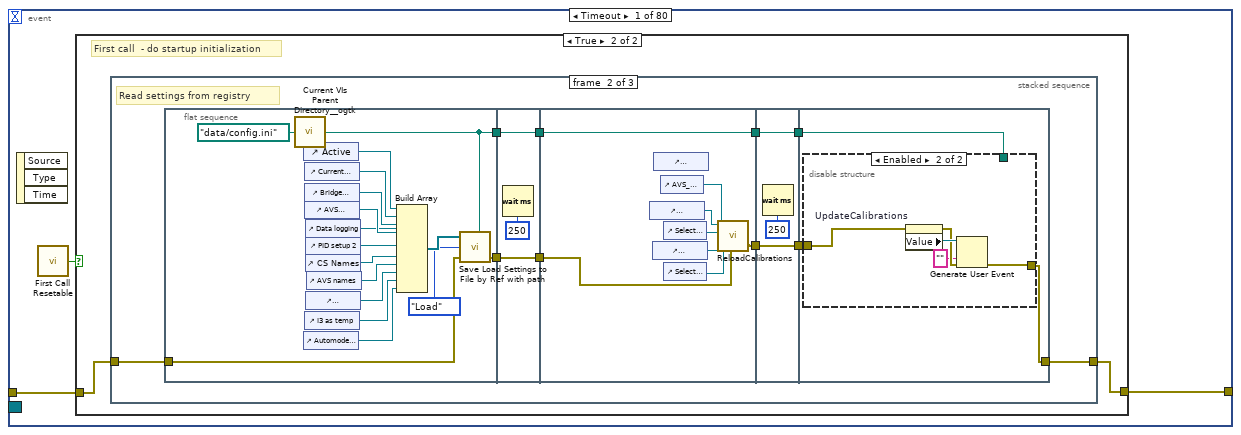
[diagram p14: hidden frame]
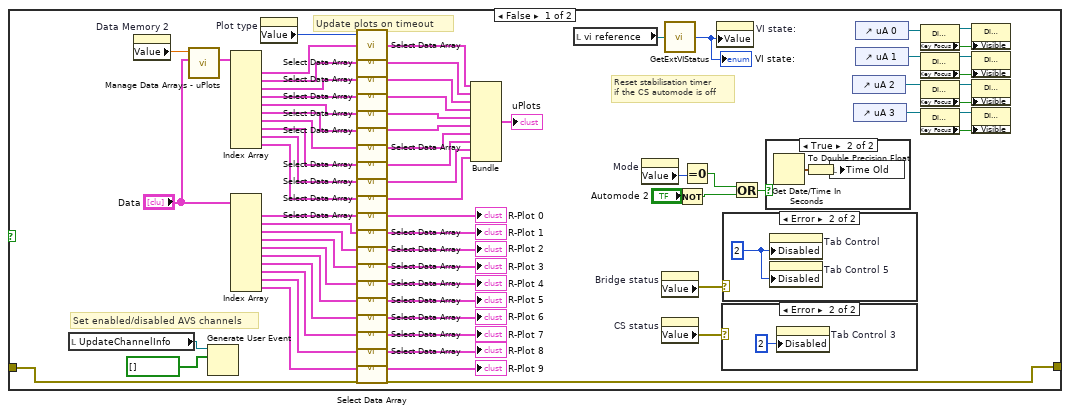
[diagram p15: hidden frame]
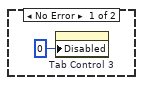
[diagram p16: hidden frame]
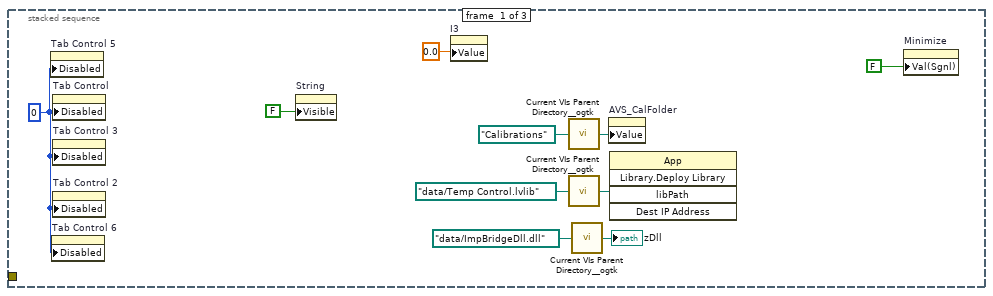
[diagram p19: hidden frame]
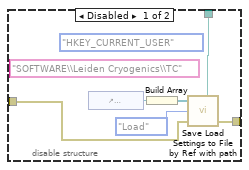
[diagram p20: hidden frame]
diagram:
  w2 = "CallExtVI"  # CallExtVI
  w4 = bool[] []  # UpdateChannelInfo
  w7 = cluster{"R/T":dbl, "Time":dbl} {"R/T"=1.0, "Time"=1.0}  # DoPID
  w8 = cluster{"R":dbl[], "T":dbl[]} {"R"=[1.0], "T"=[1.0]}  # UpdateValuesAVS
  w9 = cluster{"R":dbl[], "T":dbl[]} {"R"=[1.0], "T"=[1.0]}  # UpdateValuesZBridge
  w11 = "ResetPIDloop"  # Reset PID loop
  w13 = TRUE  # TempStabilized
  w14 = "UpdateLogFilePath"  # UpdateLogFilePath
  w17 = "UpdateCalibrations"  # UpdateCalibrations
  # "Unwired (but used) controls"
  n1 = Create User Event(user event datatype=w4) -> (user event=w20:refnum<user-event>)  [unwired: 1 in, 1 out]
  "UpdateChannelInfo" <- w20
  n2 = Create User Event(user event datatype=w8) -> (user event=w19:refnum<user-event>)  [unwired: 1 in, 1 out]
  "UpdateValuesAVS" <- w19
  n3 = Create User Event(user event datatype=w17) -> (user event=w16:refnum<user-event>)  [unwired: 1 in, 1 out]
  "UpdateCalibrations" <- w16
  n4 = Create User Event(user event datatype=w14) -> (user event=w15:refnum<user-event>)  [unwired: 1 in, 1 out]
  "UpdateLogFilePath" <- w15
  n5 = Create User Event ("TempStabilized")(user event datatype=w13) -> (user event=w1:refnum<user-event>)  [unwired: 1 in, 1 out]
  "TempStabilized" <- w1
  n6 = Create User Event(user event datatype=w11) -> (user event=w10:refnum<user-event>)  [unwired: 1 in, 1 out]
  "ResetPIDloop" <- w10
  n7 = Create User Event(user event datatype=w9) -> (user event=w6:refnum<user-event>)  [unwired: 1 in, 1 out]
  "UpdateValuesZBridge" <- w6
  n8 = Create User Event(user event datatype=w7) -> (user event=w5:refnum<user-event>)  [unwired: 1 in, 1 out]
  "DoPID" <- w5
  n9 = Create User Event(user event datatype=w2) -> (user event=w3:refnum<user-event>)  [unwired: 1 in, 1 out]
  "CallExtVI" <- w3
  n10 = register-events(w20, w19, w16, w15, w1, w10, w6, w5, w3) -> (reference out=w18:refnum<event-registration>)  [unwired: 2 in, 1 out]
  n11 = while {
    tunnel: w18 -> [w24]
    shift-right: [w21] -> _
    shift-left: errorcluster {"status"=FALSE, "code"=0, "source"=""} ("error in (no error)") -> [w22]
    stop <- FALSE stop-if-true
    # "Event handling loop"
    n12 = event shown="[4] <UpdateValuesAVS>: User Event" {
      selector: w24 -> [_ _ _ _ _ _ _ _ _ _ _ _ _ _ _ _ _ _ _ _ _ _ _ _ _ _ _ _ _ _ _ _ _ _ _ _ _ _ _ _ _ _ _ _ _ _ _ _ _ _ _ _ _ _ _ _ _ _ _ _ _ _ _ _ _ _ _ _ _ _ _ _ _ _ _ _ _ _ _ _]
      dyn-events: _ -> [_ _ _ _ _ _ _ _ _ _ _ _ _ _ _ _ _ _ _ _ _ _ _ _ _ _ _ _ _ _ _ _ _ _ _ _ _ _ _ _ _ _ _ _ _ _ _ _ _ _ _ _ _ _ _ _ _ _ _ _ _ _ _ _ _ _ _ _ _ _ _ _ _ _ _ _ _ _ _ _]
      timeout: 200 -> [_ _ _ _ _ _ _ _ _ _ _ _ _ _ _ _ _ _ _ _ _ _ _ _ _ _ _ _ _ _ _ _ _ _ _ _ _ _ _ _ _ _ _ _ _ _ _ _ _ _ _ _ _ _ _ _ _ _ _ _ _ _ _ _ _ _ _ _ _ _ _ _ _ _ _ _ _ _ _ _]
      tunnel: w22 -> [w28 _ _ w355 w404 w483 _ _ w645 _ _ w724 w732 w771 _ _ _ _ _ _ _ _ _ w964 _ w971 _ _ _ _ _ _ _ _ _ w1050 _ _ _ _ _ _ _ _ _ _ _ _ _ _ _ _ _ _ _ _ _ _ _ _ w1409 w1426 _ _ _ _ _ _ _ _ _ _ _ _ _ _ _ _ _ _]
      tunnel: [w27 _ _ w359 w403 w480 _ _ w644 _ _ w723 w732 w771 _ _ _ _ _ _ _ _ _ w964 _ w971 _ _ _ _ _ _ _ _ _ w1050 _ _ _ _ _ _ _ _ _ _ _ _ _ _ _ _ _ _ _ _ _ _ _ _ w1408 w1425 _ _ _ _ _ _ _ _ _ _ _ _ _ _ _ _ _ _] -> w21
      event Timeout {
        n13 = event-data() -> ()  [unwired: 1 in, 3 out]
        n14 = call "First Call Resetable.vi"() -> ("First Call?"=w26:bool)
        n15 = case shown="True" w26 {
          tunnel: w28 -> [w33 w104]
          tunnel: [w33 w103] -> w27
          frame False {
            # "Update plots on timeout"
            # "Set enabled/disabled AVS channels"
            # "Reset stabilisation timer\nif the CS automode is off"
            n16 = local read "UpdateChannelInfo"() -> (w34:refnum<user-event>)
            n17 = property on="Data Memory 2" class="DigNum (strict)"() -> ("Value"=w81:dbl)  [unwired: 2 in, 2 out]
            n18 = call "Manage Data Arrays - uPlots.vi"("Data In"="Data", "Data Memory"=w81) -> ("Data Out"=w36:cluster{"R":dbl[], "T":dbl[], "Time":dbl[]}[])  [unwired: 7 in]
            n19 = Generate User Event(user event=w34, event data cluster=bool[] [] ("event data")) -> ()  [unwired: 2 in, 2 out]
            n20 = Index Array(array=w36) -> (element #1=w51:cluster{"R":dbl[], "T":dbl[], "Time":dbl[]}, element #2=w52:cluster{"R":dbl[], "T":dbl[], "Time":dbl[]}, element #3=w53:cluster{"R":dbl[], "T":dbl[], "Time":dbl[]}, element #4=w54:cluster{"R":dbl[], "T":dbl[], "Time":dbl[]}, element #5=w55:cluster{"R":dbl[], "T":dbl[], "Time":dbl[]}, element #6=w56:cluster{"R":dbl[], "T":dbl[], "Time":dbl[]}, element #7=w57:cluster{"R":dbl[], "T":dbl[], "Time":dbl[]}, element #8=w58:cluster{"R":dbl[], "T":dbl[], "Time":dbl[]}, element #9=w59:cluster{"R":dbl[], "T":dbl[], "Time":dbl[]}, element #10=w60:cluster{"R":dbl[], "T":dbl[], "Time":dbl[]})  [unwired: 10 in]
            n21 = Index Array(array="Data") -> (element #1=w80:cluster{"R":dbl[], "T":dbl[], "Time":dbl[]}, element #2=w79:cluster{"R":dbl[], "T":dbl[], "Time":dbl[]}, element #3=w78:cluster{"R":dbl[], "T":dbl[], "Time":dbl[]}, element #4=w77:cluster{"R":dbl[], "T":dbl[], "Time":dbl[]}, element #5=w76:cluster{"R":dbl[], "T":dbl[], "Time":dbl[]}, element #6=w75:cluster{"R":dbl[], "T":dbl[], "Time":dbl[]}, element #7=w74:cluster{"R":dbl[], "T":dbl[], "Time":dbl[]}, element #8=w73:cluster{"R":dbl[], "T":dbl[], "Time":dbl[]}, element #9=w72:cluster{"R":dbl[], "T":dbl[], "Time":dbl[]}, element #10=w71:cluster{"R":dbl[], "T":dbl[], "Time":dbl[]})  [unwired: 10 in]
            n22 = property on="Plot type" class="Enum (strict)"() -> ("Value"=w39:enum16{"R vs Time", "T vs Time"})  [unwired: 2 in, 2 out]
            n23 = call "Select Data Array.vi"("Cluster 2"=w51, "Value"=w39) -> ("Cluster"=w61:cluster{"Time":dbl[], "T":dbl[]})
            n24 = call "Select Data Array.vi"("Cluster 2"=w52, "Value"=w39) -> ("Cluster"=w62:cluster{"Time":dbl[], "T":dbl[]})
            n25 = call "Select Data Array.vi"("Cluster 2"=w53, "Value"=w39) -> ("Cluster"=w63:cluster{"Time":dbl[], "T":dbl[]})
            n26 = call "Select Data Array.vi"("Cluster 2"=w54, "Value"=w39) -> ("Cluster"=w64:cluster{"Time":dbl[], "T":dbl[]})
            n27 = call "Select Data Array.vi"("Cluster 2"=w55, "Value"=w39) -> ("Cluster"=w70:cluster{"Time":dbl[], "T":dbl[]})
            n28 = call "Select Data Array.vi"("Cluster 2"=w56, "Value"=w39) -> ("Cluster"=w65:cluster{"Time":dbl[], "T":dbl[]})
            n29 = call "Select Data Array.vi"("Cluster 2"=w57, "Value"=w39) -> ("Cluster"=w66:cluster{"Time":dbl[], "T":dbl[]})
            n30 = call "Select Data Array.vi"("Cluster 2"=w58, "Value"=w39) -> ("Cluster"=w67:cluster{"Time":dbl[], "T":dbl[]})
            n31 = call "Select Data Array.vi"("Cluster 2"=w59, "Value"=w39) -> ("Cluster"=w68:cluster{"Time":dbl[], "T":dbl[]})
            n32 = call "Select Data Array.vi"("Cluster 2"=w60, "Value"=w39) -> ("Cluster"=w69:cluster{"Time":dbl[], "T":dbl[]})
            n33 = call "Select Data Array.vi"("Cluster 2"=w80, "Value"=w39) -> ("Cluster"=→"R-Plot 0":cluster{"Time":dbl[], "T":dbl[]})
            n34 = call "Select Data Array.vi"("Cluster 2"=w79, "Value"=w39) -> ("Cluster"=→"R-Plot 1":cluster{"Time":dbl[], "T":dbl[]})
            n35 = call "Select Data Array.vi"("Cluster 2"=w78, "Value"=w39) -> ("Cluster"=→"R-Plot 2":cluster{"Time":dbl[], "T":dbl[]})
            n36 = call "Select Data Array.vi"("Cluster 2"=w77, "Value"=w39) -> ("Cluster"=→"R-Plot 3":cluster{"Time":dbl[], "T":dbl[]})
            n37 = call "Select Data Array.vi"("Cluster 2"=w76, "Value"=w39) -> ("Cluster"=→"R-Plot 4":cluster{"Time":dbl[], "T":dbl[]})
            n38 = call "Select Data Array.vi"("Cluster 2"=w75, "Value"=w39) -> ("Cluster"=→"R-Plot 5":cluster{"Time":dbl[], "T":dbl[]})
            n39 = call "Select Data Array.vi"("Cluster 2"=w74, "Value"=w39) -> ("Cluster"=→"R-Plot 6":cluster{"Time":dbl[], "T":dbl[]})
            n40 = call "Select Data Array.vi"("Cluster 2"=w73, "Value"=w39) -> ("Cluster"=→"R-Plot 7":cluster{"Time":dbl[], "T":dbl[]})
            n41 = call "Select Data Array.vi"("Cluster 2"=w72, "Value"=w39) -> ("Cluster"=→"R-Plot 8":cluster{"Time":dbl[], "T":dbl[]})
            n42 = call "Select Data Array.vi"("Cluster 2"=w71, "Value"=w39) -> ("Cluster"=→"R-Plot 9":cluster{"Time":dbl[], "T":dbl[]})
            n43 = Bundle("Cluster"=w61, "Cluster"=w62, "Cluster"=w63, "Cluster"=w64, "Cluster"=w70, "Cluster"=w65, "Cluster"=w66, "Cluster"=w67, "Cluster"=w68, "Cluster"=w69) -> (→"uPlots":T33)  [unwired: 1 in]
            n44 = local read "vi reference"() -> (w35:refnum<vi>)
            n45 = property on="Mode" class="Enum (strict)"() -> ("Value"=w96:enum16{"Manual", "Automatic"})  [unwired: 2 in, 2 out]
            n46 = property on="Bridge status" class="Clust (strict)"() -> ("Value"=w31:errorcluster)  [unwired: 2 in, 2 out]
            n47 = property on="CS status" class="Clust (strict)"() -> ("Value"=w30:errorcluster)  [unwired: 2 in, 2 out]
            n48 = call "GetExtVIStatus.vi"("vi reference in"=w35) -> ("Exec.State"=w32:T25)  [unwired: 2 out]
            "VI state:" <- w32
            n49 = Not(x="Automode 2") -> (.not. x?=w95:bool)
            n50 = Equal To 0?(x=w96) -> (x = 0?=w29:bool)
            n51 = property on="VI state:" class="Enum (strict)"("Value"=w32) -> ()  [unwired: 2 in, 2 out]
            n52 = case shown="Error" w30 {
              frame No Error {
                n53 = property on="Tab Control 3" class="TabCtl (strict)"("Disabled"=u8 0) -> ()  [unwired: 2 in, 2 out]
              }
              frame Error {
                n54 = property on="Tab Control 3" class="TabCtl (strict)"("Disabled"=u8 2) -> ()  [unwired: 2 in, 2 out]
              }
            }
            n55 = case shown="Error" w31 {
              frame No Error {
              }
              frame Error {
                w100 = u8 2 ("Disabled")
                n56 = property on="Tab Control" class="TabCtl (strict)"("Disabled"=w100) -> ()  [unwired: 2 in, 2 out]
                n57 = property on="Tab Control 5" class="TabCtl (strict)"("Disabled"=w100) -> ()  [unwired: 2 in, 2 out]
              }
            }
            n58 = Or(x=w29, y=w95) -> (x .or. y?=w94:bool)
            n59 = case shown="True" w94 {
              frame False {
              }
              frame True {
                n60 = Get Date/Time In Seconds() -> (seconds since 1Jan1904=w101:timestamp)
                n61 = To Double Precision Float(number=w101) -> (double precision float=w102:dbl)
                n62 = local write "Time Old"(w102) -> ()
              }
            }
            n63 = control-ref of="uA 2"() -> (w82:refnum<vi>)
            n64 = control-ref of="uA 3"() -> (w83:refnum<vi>)
            n65 = control-ref of="uA 0"() -> (w93:refnum<vi>)
            n66 = control-ref of="uA 1"() -> (w89:refnum<vi>)
            n67 = property class="DigNum (strict)"(reference=w93) -> (reference out=w92:refnum<vi>, "Key Focus"=w91:bool)  [unwired: 1 in, 1 out]
            n68 = property class="DigNum (strict)"(reference=w89) -> (reference out=w90:refnum<vi>, "Key Focus"=w88:bool)  [unwired: 1 in, 1 out]
            n69 = property class="DigNum (strict)"(reference=w82) -> (reference out=w84:refnum<vi>, "Key Focus"=w85:bool)  [unwired: 1 in, 1 out]
            n70 = property class="DigNum (strict)"(reference=w83) -> (reference out=w86:refnum<vi>, "Key Focus"=w87:bool)  [unwired: 1 in, 1 out]
            n71 = property class="DigNum (strict)"(reference=w92, "Visible"=w91) -> ()  [unwired: 1 in, 2 out]
            n72 = property class="DigNum (strict)"(reference=w90, "Visible"=w88) -> ()  [unwired: 1 in, 2 out]
            n73 = property class="DigNum (strict)"(reference=w84, "Visible"=w85) -> ()  [unwired: 1 in, 2 out]
            n74 = property class="DigNum (strict)"(reference=w86, "Visible"=w87) -> ()  [unwired: 1 in, 2 out]
          }
          frame True {
            # "First call  - do startup initialization"
            n75 = stacked-sequence {
              tunnel: w104 -> [_ w124 _]
              tunnel: [_ w115 _] -> w103
              frame #0 {
                w112 = u8 0 ("Disabled")
                n76 = property on="Tab Control 5" class="TabCtl (strict)"("Disabled"=w112) -> ()  [unwired: 2 in, 2 out]
                n77 = property on="Tab Control 6" class="TabCtl (strict)"("Disabled"=w112) -> ()  [unwired: 2 in, 2 out]
                n78 = property on="Tab Control" class="TabCtl (strict)"("Disabled"=w112) -> ()  [unwired: 2 in, 2 out]
                n79 = property on="Tab Control 3" class="TabCtl (strict)"("Disabled"=w112) -> ()  [unwired: 2 in, 2 out]
                n80 = property on="Tab Control 2" class="TabCtl (strict)"("Disabled"=w112) -> ()  [unwired: 2 in, 2 out]
                n81 = property on="String" class="Str"("Visible"=FALSE) -> ()  [unwired: 2 in, 2 out]
                n82 = property on="I3" class="DigNum (strict)"("Value"=0.0 ("I3")) -> ()  [unwired: 2 in, 2 out]
                n83 = call "Current VIs Parent Directory__ogtk.vi"("Relative path (.)"=path "Calibrations" ("Library Path")) -> ("Parent Directory (+ Relative)"=w108:path)  [unwired: 4 in]
                n84 = call "Current VIs Parent Directory__ogtk.vi"("Relative path (.)"=path "data/Temp Control.lvlib" ("Library Path")) -> ("Parent Directory (+ Relative)"=w110:path)  [unwired: 4 in]
                n85 = call "Current VIs Parent Directory__ogtk.vi"("Relative path (.)"=path "data/ImpBridgeDll.dll" ("Library Path")) -> ("Parent Directory (+ Relative)"=→"zDll":path)  [unwired: 4 in]
                n86 = property on="AVS_CalFolder" class="Path"("Value"=w108) -> ()  [unwired: 2 in, 2 out]
                n87 = invoke class="App" method="Library.Deploy Library"("libPath"=w110) -> ()  [unwired: 4 in, 5 out]
                n88 = property on="Minimize" class="Bool (strict)"("Val(Sgnl)"=FALSE ("Value (Signaling)")) -> ()  [unwired: 2 in, 2 out]
              }
              frame #1 {
                # "Read settings from registry"
                n89 = flat-sequence {
                  tunnel: [w138] -> w123
                  tunnel: w124 -> [w137]
                  tunnel: [w135] -> w122
                  tunnel: w123 -> [w144]
                  tunnel: [w144] -> w121
                  tunnel: [w142] -> w120
                  tunnel: w122 -> [w142]
                  tunnel: [w149] -> w119
                  tunnel: w121 -> [w148]
                  tunnel: [w146] -> w118
                  tunnel: w120 -> [w146]
                  tunnel: w119 -> [w155]
                  tunnel: [w155] -> w117
                  tunnel: [w153] -> w116
                  tunnel: w118 -> [w153]
                  tunnel: w117 -> [w158]
                  tunnel: [w157] -> w115
                  tunnel: w116 -> [w156]
                  frame #0 {
                    n90 = call "Current VIs Parent Directory__ogtk.vi"("Relative path (.)"=path "data/config.ini") -> ("Parent Directory (+ Relative)"=w135:path)  [unwired: 4 in]
                    n91 = control-ref of="Active"() -> (w127:refnum<vi>)
                    n92 = control-ref of="Automode Settings 2"() -> (w125:refnum<vi>)
                    n93 = control-ref of="Current source settings"() -> (w128:refnum<vi>)
                    n94 = control-ref of="Bridge settings"() -> (w139:refnum<vi>)
                    n95 = control-ref of="AVS Runtime Settings"() -> (w134:refnum<vi>)
                    n96 = control-ref of="I3 as temp"() -> (w126:refnum<vi>)
                    n97 = control-ref of="Data logging"() -> (w133:refnum<vi>)
                    n98 = control-ref of="PID setup 2"() -> (w132:refnum<vi>)
                    n99 = control-ref of="CS Names"() -> (w131:refnum<vi>)
                    n100 = control-ref of="CurCalibrations"() -> (w129:refnum<vi>)
                    n101 = control-ref of="AVS names"() -> (w130:refnum<vi>)
                    n102 = Build Array(w127, w128, w139, w134, w133, w132, w131, w130, w129, w126, w125) -> (w141:refnum<vi>[])
                    n103 = call "Save Load Settings to File by Ref with path.vi"("Array of Cluster References"=w141, "Action"=enum8{"Load", "Save"}."Load", "error in (no error)"=w137, "configuration file path"=w135) -> ("error out"=w138:errorcluster)  [unwired: 5 in]
                  }
                  frame #1 {
                    n104 = Wait (ms)(milliseconds to wait=250) -> ()  [unwired: 1 out]
                  }
                  frame #2 {
                    n105 = control-ref of="Thermometer"() -> (w147:refnum<vi>)
                    n106 = control-ref of="CurCalibrations"() -> (w145:refnum<vi>)
                    n107 = control-ref of="CurCalibrations"() -> ()  [unwired: 1 out]
                    n108 = control-ref of="AVS_CalFolder"() -> (w151:refnum<vi>)
                    n109 = control-ref of="Select sensor 1"() -> (w152:refnum<vi>)
                    n110 = control-ref of="Select sensor 1"() -> (w150:refnum<vi>)
                    n111 = call "ReloadCalibrations.vi"("error in (no error)"=w148, "Quick convert sensors"=w150, "CurCalibrations"=w145, "Calibration files path"=w151, "Channel1 sensors"=w152, "Channels list"=w147) -> ("error out"=w149:errorcluster)  [unwired: 1 in]
                  }
                  frame #3 {
                    n112 = Wait (ms)(milliseconds to wait=250) -> ()  [unwired: 1 out]
                  }
                  frame #4 {
                    n113 = disable-structure shown="Enabled" {
                      disable-tunnel: w158 -> [w161 w168]
                      disable-tunnel: [w160 w166] -> w157
                      disable-tunnel: w156 -> [w159 _]
                      frame Disabled {
                        (unwired) "SOFTWARE\\Leiden Cryogenics\\TC" ("subkey 2")
                        (unwired) T34."HKEY_CURRENT_USER" ("root key (HKEY_LOCAL_MACHINE) 2")
                        n114 = control-ref of="Thermometer"() -> (w163:refnum<vi>)
                        n115 = Build Array(w163) -> (w162:refnum<vi>[])
                        n116 = call "Save Load Settings to File by Ref with path.vi"("Array of Cluster References"=w162, "Action"=enum8{"Load", "Save"}."Load", "error in (no error)"=w161, "configuration file path"=w159) -> ("error out"=w160:errorcluster)  [unwired: 5 in]
                      }
                      frame Enabled {
                        n117 = property on="UpdateCalibrations" class="TypRef (strict)"(error in=w168) -> (error out=w167:errorcluster, "Value"=w169:refnum<user-event>)  [unwired: 1 in, 1 out]
                        n118 = Generate User Event(user event=w169, event data cluster="" ("event data"), error in=w167) -> (error out=w166:errorcluster)  [unwired: 1 in, 1 out]
                      }
                    }
                  }
                }
              }
              frame #2 {
                w179 = 0.0 ("T_error")
                w180 = u8 0 ("Disabled")
                # "Set enabled/disabled AVS channels"
                # "Print VI version on low left corner"
                # "Reset Current lists\nto first element"
                # "Reset pid parameters"
                # "Hardware settings"
                # "Reset currents lists"
                # "Set initial controls state"
                n119 = property on="Start" class="Bool"("Visible"=TRUE, "Disabled"=u8 0, "Value"=FALSE ("start")) -> ()  [unwired: 2 in, 2 out]
                n120 = property on="I_list_idx" class="DigNum (strict)"("Val(Sgnl)"=1 ("Value (Signaling)")) -> ()  [unwired: 2 in, 2 out]
                n121 = property on="Mode" class="Enum (strict)"("Val(Sgnl)"=enum16{"Manual", "Automatic"}."Manual" ("Value (Signaling)")) -> ()  [unwired: 2 in, 2 out]
                n122 = property on="I_tofirst" class="Bool (strict)"("Val(Sgnl)"=TRUE ("Value (Signaling)")) -> ()  [unwired: 2 in, 2 out]
                n123 = property on="AVS type" class="Enum (strict)"("Disabled"=w180) -> ()  [unwired: 2 in, 2 out]
                n124 = property on="Address" class="VISAName"("Disabled"=w180) -> ()  [unwired: 2 in, 2 out]
                n125 = property on="TCS_Port" class="VISAName"("Disabled"=w180) -> ()  [unwired: 2 in, 2 out]
                n126 = property on="CS type" class="Enum (strict)"("Disabled"=w180) -> ()  [unwired: 2 in, 2 out]
                n127 = property on="QCS/PCS Device" class="DigNum (strict)"("Disabled"=w180) -> ()  [unwired: 2 in, 2 out]
                n128 = property on="Set QCS Channel 0 output to" class="Enum (strict)"("Disabled"=u8 2, "Value"=T24."Channel 0" ("Map Channel 0 to")) -> ()  [unwired: 2 in, 2 out]
                n129 = property class="App"() -> ("App.Kind"=w175:T35)  [unwired: 2 in, 2 out]
                n130 = case shown="\"Run Time System\"" w175 {
                  tunnel: [w185 w196] -> w176
                  frame "invalid app kind", Default {
                    n131 = control-ref of="This VI"() -> (w192:refnum<vi>)
                    n132 = property class="VI"(reference=w192) -> ("Hist.Revision"=w191:u32)  [unwired: 1 in, 2 out]
                    n133 = Divide(x=w191, y=1000.0 ("x")) -> (x/y=w187:dbl)
                    n134 = Number To Fractional String(use system decimal point (T)=FALSE, number=w187, precision (6)=i16 2) -> (F-format string=w186:string)  [unwired: 1 in]
                    n135 = Concatenate Strings("" ("string"), w186) -> (w185:string)
                  }
                  frame "Run Time System" {
                    n136 = Current VI's Path() -> (path=w198:path)
                    n137 = Strip Path(path=w198) -> (stripped path=w197:path)  [unwired: 1 out]
                    n138 = Path To String(path=w197) -> (string=w195:string)
                    n139 = invoke class="FileVersionInfo" method="GetVersionInfo"(reference=refnum<k24> refnum (".NET object"), "fileName"=w195) -> ("GetVersionInfo"=w194:refnum<k24>)  [unwired: 2 in, 3 out]
                    n140 = property class="FileVersionInfo"(reference=w194) -> ("FileVersion"=w196:string)  [unwired: 1 in, 2 out]
                  }
                }
                "Revision" <- w176
                n141 = local write "Error"(w179) -> ()
                n142 = local write "Int"(w179) -> ()
                n143 = local read "UpdateChannelInfo"() -> (w174:refnum<user-event>)
                n144 = Generate User Event(user event=w174, event data cluster=bool[] [] ("event data")) -> ()  [unwired: 2 in, 2 out]
              }
            }
          }
        }
      }
      event "Start": Value Change {
        # "\"Start\" button clicked -> start measuring"
        n145 = event-data() -> ()  [unwired: 1 in, 6 out]
        n146 = stacked-sequence {
          frame #0 {
            n147 = property on="Run description" class="Str"() -> ("Value"=w201:string)  [unwired: 2 in, 2 out]
            n148 = property on="Ask on start?" class="Bool (strict)"() -> ("Value"=w200:bool)  [unwired: 2 in, 2 out]
            n149 = Not(x=w200) -> (.not. x?=w199:bool)
            n150 = call "Run Reference DLG.vi"("Enable"=w200, "Run Reference"=w201, "Dont' ask again"=w199) -> ("Dont' ask again"=w203:bool, "Run Reference"=w204:string, "OK"=w205:bool)  [unwired: 13 in, 1 out]
            n151 = Not(x=w203) -> (.not. x?=w202:bool)
            n152 = case shown="True" w205 {
              tunnel: w204 -> [_ w207]
              tunnel: w202 -> [_ w206]
              frame False {
              }
              frame True {
                n153 = property on="Run description" class="Str"("Val(Sgnl)"=w207) -> ()  [unwired: 2 in, 2 out]
                n154 = property on="Ask on start?" class="Bool (strict)"("Val(Sgnl)"=w206) -> ()  [unwired: 2 in, 2 out]
              }
            }
          }
          frame #1 {
            (unwired) T34."HKEY_CURRENT_USER" ("root key (HKEY_LOCAL_MACHINE) 2")
            # "Save new settings to config file"
            n155 = control-ref of="Active"() -> (w211:refnum<vi>)
            n156 = control-ref of="I3 as temp"() -> (w210:refnum<vi>)
            n157 = control-ref of="Automode Settings 2"() -> (w209:refnum<vi>)
            n158 = control-ref of="Automode Settings 2"() -> (w208:refnum<vi>)
            n159 = control-ref of="CS Names"() -> (w216:refnum<vi>)
            n160 = control-ref of="AVS names"() -> (w215:refnum<vi>)
            n161 = control-ref of="CurCalibrations"() -> (w212:refnum<vi>)
            n162 = control-ref of="Bridge settings"() -> (w222:refnum<vi>)
            n163 = control-ref of="AVS Runtime Settings"() -> (w223:refnum<vi>)
            n164 = control-ref of="Current source settings"() -> (w221:refnum<vi>)
            n165 = control-ref of="Thermometer"() -> (w224:refnum<vi>)
            n166 = control-ref of="PID setup 2"() -> (w225:refnum<vi>)
            n167 = control-ref of="Data logging"() -> (w220:refnum<vi>)
            n168 = Build Array(w211, w222, w223, w221, w220, w224, w225, w216, w215, w212, w210, w209, w208) -> (w218:refnum<vi>[])
            n169 = call "Current VIs Parent Directory__ogtk.vi"("Relative path (.)"=path "data/config.ini") -> ("Parent Directory (+ Relative)"=w213:path)  [unwired: 4 in]
            n170 = call "Save Load Settings to File by Ref with path.vi"("Array of Cluster References"=w218, "subkey"="SOFTWARE\\Leiden Cryogenics\\TC" ("subkey 2"), "Action"=enum8{"Load", "Save"}."Save", "configuration file path"=w213) -> ()  [unwired: 5 in, 1 out]
          }
          frame #2 {
            w238 = u8 2 ("Disabled")
            # "Reset stop button"
            # "Hide Start button"
            # "Load external calibration VI"
            # "Set controls\nInitialize data for run"
            # "Lock hardware settings"
            n171 = property on="AVS type" class="Enum (strict)"("Disabled"=w238) -> ()  [unwired: 2 in, 2 out]
            n172 = property on="Address" class="VISAName"("Disabled"=w238) -> ()  [unwired: 2 in, 2 out]
            n173 = property on="AVS_SPort" class="VISAName"("Disabled"=w238) -> ()  [unwired: 2 in, 2 out]
            n174 = property on="TCS_Port" class="VISAName"("Disabled"=w238) -> ()  [unwired: 2 in, 2 out]
            n175 = property on="CS type" class="Enum (strict)"("Disabled"=w238) -> ()  [unwired: 2 in, 2 out]
            n176 = property on="QCS/PCS Device" class="DigNum (strict)"("Disabled"=w238) -> ()  [unwired: 2 in, 2 out]
            n177 = property on="Set QCS Channel 0 output to" class="Enum (strict)"("Disabled"=u8 0) -> ()  [unwired: 2 in, 2 out]
            n178 = Get Date/Time In Seconds() -> (seconds since 1Jan1904=w237:timestamp)
            n179 = To Double Precision Float(number=w237) -> (double precision float=w236:dbl)
            n180 = local write "Time Old"(w236) -> ()
            n181 = property on="External VI path" class="Path"() -> ("Value"=w235:path)  [unwired: 2 in, 2 out]
            n182 = vi-ref "OnTempStabilizedRef.vi"() -> (w234:refnum<vi>)
            n183 = Open VI Reference(type specifier VI Refnum (for type only)=w234, vi path=w235) -> (vi reference=→"vi reference":refnum<vi>)  [unwired: 4 in, 1 out]
            n184 = local write "VI called?"(FALSE ("VI called?")) -> ()
            n185 = disable-structure shown="Disabled" {
              frame Disabled {
                (unwired) 0.0 ("Value")
              }
              frame Enabled {
              }
            }
            n186 = property on="Start" class="Bool"("Visible"=FALSE, "Disabled"=u8 2) -> ()  [unwired: 2 in, 2 out]
            n187 = Initialize Array(cluster{"R":dbl[], "T":dbl[], "Time":dbl[]} {"R"=[], "T"=[], "Time"=[]}, 10 ("dimension size")) -> (w229:cluster{"R":dbl[], "T":dbl[], "Time":dbl[]}[])
            n188 = disable-structure shown="Enabled" {
              frame Enabled {
                n189 = property on="Stop" class="Bool (strict)"("Value"=FALSE ("MainStopButton")) -> ()  [unwired: 2 in, 2 out]
              }
              frame Disabled {
              }
            }
            n190 = local write "Data"(w229) -> ()
          }
          frame #3 {
            # "Initialize CS"
            n191 = local read "CS ref"() -> (w250:refnum<class "CS.lvclass">)
            n192 = call-dynamic "Initialize.vi"("CS in"=w250, "HW Address"="HW Address", "error in (no error)"=T28 {"error"=FALSE, "code"=0, "source"=""} ("error in")) -> ("CS out"=w243:refnum<class "CS.lvclass">, "Instrument ID"=→"ID":string, "error out"=w242:errorcluster)  [unwired: 10 in]
            n193 = call-dynamic "Get Currents & Ranges.vi"("CS.lvclass in"=w243, "error in (no error)"=w242) -> ("CS.lvclass out"=w251:refnum<class "CS.lvclass">, "I0"=w252:cluster{"Value":dbl, "Range":dbl}, "I1"=w244:cluster{"Value":dbl, "Range":dbl}, "I2"=w245:cluster{"Value":dbl, "Range":dbl}, "I3"=w246:cluster{"Value":dbl, "Range":dbl}, "error out"=w248:errorcluster)  [unwired: 12 in]
            "CS status" <- w248
            n194 = local write "CS ref"(w251) -> ()
            n195 = Unbundle By Name(w248) -> ("status"=w240:bool)
            n196 = case shown="False" w240 {
              tunnel: w244 -> [w264 _]
              tunnel: w245 -> [w263 _]
              tunnel: w246 -> [w262 _]
              tunnel: w252 -> [w256 _]
              frame False {
                n197 = Unbundle By Name(w256) -> ("Value"=w255:dbl, "Range"=w254:dbl)
                n198 = Unbundle By Name(w264) -> ("Value"=w261:dbl, "Range"=w260:dbl)
                n199 = Unbundle By Name(w263) -> ("Value"=w259:dbl, "Range"=w258:dbl)
                n200 = Unbundle By Name(w262) -> ("Value"=w253:dbl, "Range"=w257:dbl)
                n201 = property on="I" class="DigNum (strict)"("Value"=w255) -> ()  [unwired: 2 in, 2 out]
                n202 = property on="I" class="DigNum (strict)"("Value"=w261) -> ()  [unwired: 2 in, 2 out]
                n203 = property on="I" class="DigNum (strict)"("Value"=w259) -> ()  [unwired: 2 in, 2 out]
                n204 = property on="I" class="DigNum (strict)"("Value"=w253) -> ()  [unwired: 2 in, 2 out]
                n205 = property on="Range" class="Enum (strict)"("Value"=w254) -> ()  [unwired: 2 in, 2 out]
                n206 = property on="Range" class="Enum (strict)"("Value"=w260) -> ()  [unwired: 2 in, 2 out]
                n207 = property on="Range" class="Enum (strict)"("Value"=w258) -> ()  [unwired: 2 in, 2 out]
                n208 = property on="Range" class="Enum (strict)"("Value"=w257) -> ()  [unwired: 2 in, 2 out]
                n209 = local write "I0"(w253) -> ()
                n210 = property on="I3" class="DigNum (strict)"("Value"=w253) -> ()  [unwired: 2 in, 2 out]
              }
              frame True {
              }
            }
          }
          frame #4 {
            # "Initialize AVS/zBridge"
            n211 = property on="AVS type" class="Enum (strict)"() -> ("Value"=w268:T30)  [unwired: 2 in, 2 out]
            n212 = case shown="\"AVS47B (RS232 interface)\"" w268 {
              tunnel: [w276 w285 refnum<visa-resource-name> refnum ("dup VISA session") refnum<visa-resource-name> refnum ("dup VISA session")] -> w267
              tunnel: [w275 w288 w301 errorcluster {"status"=FALSE, "code"=0, "source"=""} ("error out")] -> w266
              tunnel: [TRUE ("start 2") TRUE ("start 2") TRUE ("start 2") TRUE ("start 2")] -> w269
              frame "AVS47A (GPIB interface)" {
                # "Set default Parameters,\n enable Autoranging"
                n213 = property on="Address" class="VISAName"() -> ("Value"=w270:refnum<visa-resource-name>)  [unwired: 2 in, 2 out]
                n214 = call "AVS47IB Initialize.vi"("Instr. Descriptor (GPIB::)"=w270) -> ("VISA session"=w284:refnum<visa-resource-name>, "error out"=w271:errorcluster)  [unwired: 13 in]
                n215 = call "AVS47IB Stop.vi"("VISA session"=w284, "error in (no error)"=w271) -> ("dup VISA session"=w282:refnum<visa-resource-name>, "error out"=w274:errorcluster)  [unwired: 12 in]
                n216 = call "AVS47IB Go Remote.vi"("VISA session"=w282, "error in (no error)"=w274) -> ("dup VISA session"=w283:refnum<visa-resource-name>, "error out"=w273:errorcluster)  [unwired: 12 in]
                n217 = call "AVS47IB Configure 47IB.vi"("VISA session"=w283, "Printer Enabled (-1:no change)"=i8 0, "Buffer Enabled (-1:no change)"=i8 0, "Message Headers Included  (-1:no change)"=i8 0, "Autoranging Enabled (-1:no change)"=i8 1, "Stabilisation Delay (-1:no change)"=i8 15, "error in (no error)"=w273) -> ("dup VISA session"=w276:refnum<visa-resource-name>, "error out"=w275:errorcluster)  [unwired: 7 in]
              }
              frame "AVS47B (RS232 interface)" {
                n218 = property on="Bridge settings" class="Clust (strict)"() -> ("Value"=w293:T20)  [unwired: 2 in, 2 out]
                n219 = Unbundle By Name(w293) -> ("AVS_SPort"=w292:refnum<visa-resource-name>)
                n220 = call "InitPort_b.vi"("VISA resource"=w292) -> ("error out"=w287:errorcluster, "dup VISA resource"=w291:refnum<visa-resource-name>)  [unwired: 5 in]
                n221 = Type Cast(type=refnum<visa-resource-name> refnum ("dup VISA session"), x=w291) -> (*(type *) &x=w286:refnum<visa-resource-name>)
                n222 = case shown="No Error" w287 {
                  selector: w287 -> [w294 w297]
                  tunnel: w286 -> [w295 w299]
                  tunnel: [w294 w298] -> w288
                  tunnel: [w295 refnum<visa-resource-name> refnum ("dup VISA session")] -> w285
                  frame No Error {
                  }
                  frame Error {
                    n223 = VISA Close(VISA resource name=w299, error in (no error)=w297) -> (error out=w298:errorcluster)
                  }
                }
              }
              frame "Impedance Bridge" {
                n224 = local read "zDll"() -> (w300:path)
                n225 = call "StartScan.vi"("path in"=w300) -> ("error out"=w301:errorcluster)  [unwired: 9 in, 1 out]
              }
              frame "Disabled", Default {
              }
            }
            "AVS VISA session" <- w267
            "start 2" <- w269
            n226 = property on="Data array" class="Arr (strict)"("Value"=dbl[] [0.0, 0.0, 0.0, 0.0, 0.0, 0.0, 0.0, 0.0, 0.0, 0.0] ("R_array")) -> ()  [unwired: 2 in, 2 out]
            n227 = property on="Bridge status" class="Clust (strict)"("Value"=w266) -> ()  [unwired: 2 in, 2 out]
          }
          frame #5 {
            # "Generate paths for log files"
            n228 = Unbundle By Name("Data logging") -> ("Run description"=w308:string, "Filenames suffix"=w309:string, "AVS_Path"=w311:path, "AVS_FName"=w313:string, "CAL_FName"=w312:string)
            n229 = call "MGI Make String Filesafe.vi"("String In"=w308) -> ("Filesafe String Out"=w307:string)
            n230 = call "GeneratePaths.vi"("Filename Suffix"=w309, "Run description"=w307, "AVS_Path"=w311, "AVS_FName"=w313, "CAL_Path"=w311, "CAL_FName"=w312) -> ("Generated Log path"=w310:path, "Generated Calib path"=→"Calib path":path)  [unwired: 8 in]
            n231 = property on="Log path" class="Path"("Val(Sgnl)"=w310) -> ()  [unwired: 2 in, 2 out]
          }
        }
      }
      event "Stop": Value Change; Application Instance Close {
        # "\"Stop\" button pressed -> Stop measuring."
        n232 = event-data() -> ()  [unwired: 1 in, 3 out]
        n233 = flat-sequence {
          frame #0 {
            (unwired) T34."HKEY_CURRENT_USER" ("root key (HKEY_LOCAL_MACHINE) 2")
            # "Save settings to config file"
            n234 = control-ref of="Active"() -> (w318:refnum<vi>)
            n235 = control-ref of="Bridge settings"() -> (w327:refnum<vi>)
            n236 = control-ref of="AVS Runtime Settings"() -> (w326:refnum<vi>)
            n237 = control-ref of="Current source settings"() -> (w328:refnum<vi>)
            n238 = control-ref of="Data logging"() -> (w329:refnum<vi>)
            n239 = control-ref of="Thermometer"() -> (w325:refnum<vi>)
            n240 = control-ref of="PID setup 2"() -> (w324:refnum<vi>)
            n241 = control-ref of="CS Names"() -> (w323:refnum<vi>)
            n242 = control-ref of="AVS names"() -> (w322:refnum<vi>)
            n243 = control-ref of="CurCalibrations"() -> (w319:refnum<vi>)
            n244 = control-ref of="I3 as temp"() -> (w317:refnum<vi>)
            n245 = control-ref of="Automode Settings 2"() -> (w316:refnum<vi>)
            n246 = call "Current VIs Parent Directory__ogtk.vi"("Relative path (.)"=path "data/config.ini") -> ("Parent Directory (+ Relative)"=w320:path)  [unwired: 4 in]
            n247 = Build Array(w318, w327, w326, w328, w329, w325, w324, w323, w322, w319, w317, w316) -> (w331:refnum<vi>[])
            n248 = call "Save Load Settings to File by Ref with path.vi"("Array of Cluster References"=w331, "subkey"="SOFTWARE\\Leiden Cryogenics\\TC" ("subkey 2"), "Action"=enum8{"Load", "Save"}."Save", "configuration file path"=w320) -> ()  [unwired: 5 in, 1 out]
          }
          frame #1 {
            # "Free serial ports"
            n249 = control-ref of="AVS VISA session"() -> (w334:refnum<vi>)
            n250 = control-ref of="TCS_Port"() -> (w339:refnum<vi>)
            n251 = local read "zDll"() -> (w333:path)
            n252 = call "StopScan.vi"("path in"=w333) -> ()  [unwired: 9 in, 2 out]
            n253 = property class="VISAName"(reference=w334) -> (error out=w336:errorcluster, "Value"=w335:refnum<visa-resource-name>)  [unwired: 1 in, 1 out]
            n254 = property class="VISAName"(reference=w339) -> (error out=w337:errorcluster, "Value"=w338:refnum<visa-resource-name>)  [unwired: 1 in, 1 out]
            n255 = VISA Close(VISA resource name=w335, error in (no error)=w336) -> ()  [unwired: 1 out]
            n256 = VISA Close(VISA resource name=w338, error in (no error)=w337) -> ()  [unwired: 1 out]
          }
          frame #2 {
            w342 = u8 0 ("Disabled")
            # "Reset controls state"
            n257 = property on="Start" class="Bool"("Visible"=TRUE, "Disabled"=u8 0, "Value"=FALSE ("start")) -> ()  [unwired: 2 in, 2 out]
            n258 = property on="Stop" class="Bool (strict)"("Value"=FALSE ("MainStopButton")) -> ()  [unwired: 2 in, 2 out]
            n259 = property on="start 2" class="Bool (strict)"("Value"=FALSE ("start 2")) -> ()  [unwired: 2 in, 2 out]
            n260 = property on="AVS type" class="Enum (strict)"("Disabled"=w342) -> ()  [unwired: 2 in, 2 out]
            n261 = property on="Address" class="VISAName"("Disabled"=w342) -> ()  [unwired: 2 in, 2 out]
            n262 = property on="AVS_SPort" class="VISAName"("Disabled"=w342) -> ()  [unwired: 2 in, 2 out]
            n263 = property on="TCS_Port" class="VISAName"("Disabled"=w342) -> ()  [unwired: 2 in, 2 out]
            n264 = property on="CS type" class="Enum (strict)"("Disabled"=w342) -> ()  [unwired: 2 in, 2 out]
            n265 = property on="QCS/PCS Device" class="DigNum (strict)"("Disabled"=w342) -> ()  [unwired: 2 in, 2 out]
          }
          frame #3 {
            w346 = u8 2 ("Disabled")
            # "Disable UI"
            n266 = property on="Tab Control 6" class="TabCtl (strict)"("Disabled"=w346) -> ()  [unwired: 2 in, 2 out]
            n267 = property on="Tab Control" class="TabCtl (strict)"("Disabled"=w346) -> ()  [unwired: 2 in, 2 out]
            n268 = property on="Tab Control 3" class="TabCtl (strict)"("Disabled"=w346) -> ()  [unwired: 2 in, 2 out]
            n269 = property on="Tab Control 2" class="TabCtl (strict)"("Disabled"=w346) -> ()  [unwired: 2 in, 2 out]
            n270 = property on="Tab Control 5" class="TabCtl (strict)"("Disabled"=w346) -> ()  [unwired: 2 in, 2 out]
            n271 = property on="String" class="Str"("Visible"=TRUE) -> ()  [unwired: 2 in, 2 out]
          }
          frame #4 {
            # "Stop execution"
            n272 = Stop(stop? (T)=TRUE) -> ()
          }
        }
      }
      event "Data array": Value Change {
        # "Received new data from AVS/zBridge. Do general tasks - update indicators, calculate temperature and pass the data further to \nAVS/zBridge specific processing"
        n273 = event-data() -> ("NewVal"=w352:dbl[])  [unwired: 1 in, 4 out]
        n274 = for {
          tunnel: w352 -> [w384] mode=indexing
          tunnel: [w382] -> w351 mode=indexing
          n275 = Less?(x=w384, y=1e+25) -> (x < y?=w385:bool)
          n276 = Select(t=w384, s=w385, f=inf) -> (s? t:f=w382:dbl)
        }
        n277 = Index Array(array=w351) -> (element #1=→"R 0":dbl, element #2=→"R 1":dbl, element #3=→"R 2":dbl, element #4=→"R 3":dbl, element #5=→"R 4":dbl, element #6=→"R 5":dbl, element #7=→"R 6":dbl, element #8=→"R 7":dbl, element #9=→"R 8":dbl, element #10=→"R 9":dbl)  [unwired: 10 in]
        n278 = Array To Cluster(array=w351) -> (cluster=→"R":T36)
        n279 = local read "CurCalibrations"() -> (w354:T18)
        n280 = property on="AVS_CalFolder" class="Path"() -> ("Value"=w363:path)  [unwired: 2 in, 2 out]
        n281 = Cluster To Array(cluster=w354) -> (array=w353:string[])
        n282 = call "Resistance to Temp no Ext.vi"("error in"=w355, "Path"=w363, "CurCalibrations"=w353, "Resistance"=w351) -> ("Temperature"=w358:dbl[])  [unwired: 1 in, 3 out]
        "T_array" <- w358
        n283 = Array To Cluster(array=w358) -> (cluster=w361:T37)
        "T" <- w361
        n284 = Unbundle(w361) -> ("Temperature[0]"=→"T 01":dbl, "Temperature[1]"=→"T 02":dbl, "Temperature[2]"=→"T 03":dbl, "Temperature[3]"=→"T 04":dbl, "Temperature[4]"=→"T 05":dbl, "Temperature[5]"=→"T 06":dbl, "Temperature[6]"=→"T 07":dbl, "Temperature[7]"=→"T 08":dbl, "Temperature[8]"=→"T 9":dbl, "Temperature[9]"=→"T 10":dbl)
        n285 = property on="Mode Buttons" class="RadioBtnsControl (strict)"() -> ("Value"=w360:T11)  [unwired: 2 in, 2 out]
        n286 = case shown="\"No Selection\", Default" w360 {
          tunnel: w358 -> [w399 _]
          tunnel: w351 -> [w398 _]
          frame "No Selection", Default {
            n287 = Get Date/Time In Seconds() -> (seconds since 1Jan1904=w397:timestamp)
            n288 = To Double Precision Float(number=w397) -> (double precision float=→"Time":dbl)
            "Small T" <- w399
            "Small R" <- w398
          }
          frame "Cursor Mode" {
          }
        }
        n289 = Bundle(w351, "Temperature"=w358) -> (w357:cluster{dbl[], "Temperature":dbl[]})  [unwired: 1 in]
        n290 = property on="AVS type" class="Enum (strict)"() -> ("Value"=w356:T30)  [unwired: 2 in, 2 out]
        n291 = case shown="\"Impedance Bridge\"" w356 {
          tunnel: [w390 w391 w394] -> w359
          tunnel: w355 -> [w389 w391 w395]
          tunnel: w357 -> [w387 _ w393]
          frame Default {
            n292 = local read "UpdateValuesAVS"() -> (w388:refnum<user-event>)
            n293 = Generate User Event(user event=w388, event data cluster=w387, error in=w389) -> (error out=w390:errorcluster)  [unwired: 1 in, 1 out]
          }
          frame "Disabled" {
          }
          frame "Impedance Bridge" {
            n294 = local read "UpdateValuesZBridge"() -> (w392:refnum<user-event>)
            n295 = Generate User Event(user event=w392, event data cluster=w393, error in=w395) -> (error out=w394:errorcluster)  [unwired: 1 in, 1 out]
          }
        }
      }
      event User Event {
        # "Process data from the AVS bridge"
        n296 = event-data() -> ("R"=w401:dbl[], "T"=w400:dbl[])  [unwired: 1 in]
        n297 = property on="All I" class="Arr (strict)"() -> ("Value"=w402:dbl[])  [unwired: 2 in, 2 out]
        n298 = stacked-sequence {
          tunnel: w404 -> [_ w431]
          tunnel: [_ w445] -> w403
          tunnel: w402 -> [_ w427]
          tunnel: w401 -> [w423 w429]
          tunnel: w400 -> [w424 w428]
          frame #0 {
            # "Filter data and add it to the data array. \nDo PID"
            n299 = property on="AVS Runtime Settings" class="Clust (strict)"() -> ("Value"=w412:T12)  [unwired: 2 in, 2 out]
            n300 = Unbundle By Name(w412) -> ("Y_max"=w415:dbl, "Y_min"=w414:dbl, "Filter graphs:"=w413:bool)
            n301 = local read "Data"() -> (w409:cluster{"R":dbl[], "T":dbl[], "Time":dbl[]}[])
            n302 = property on="Data Memory" class="DigNum (strict)"() -> ("Value"=w417:u16)  [unwired: 2 in, 2 out]
            n303 = Get Date/Time In Seconds() -> (seconds since 1Jan1904=w411:timestamp)
            n304 = To Double Precision Float(number=w411) -> (double precision float=w408:dbl)
            n305 = call "Manage Data Arrays - AVS.vi"("Y_max"=w415, "Y_min"=w414, "Filter Graph Results"=w413, "Append New Data"=TRUE, "Data In"=w409, "Curr R"=w423, "Curr T"=w424, "Curr Time"=w408, "Data Memory"=w417) -> ("Data Out"=w410:cluster{"R":dbl[], "T":dbl[], "Time":dbl[]}[])  [unwired: 10 in]
            n306 = property on="FB on" class="Enum (strict)"() -> ("Value"=w405:enum16{"Resistance", "Temperature"})  [unwired: 2 in, 2 out]
            n307 = local write "Data"(w410) -> ()
            n308 = property on="AVS Channel" class="DigNum (strict)"() -> ("Value"=w406:i32)  [unwired: 2 in, 2 out]
            n309 = Index Array(array=w423, index=w406) -> (element=w422:dbl)
            n310 = Index Array(array=w424, index=w406) -> (element=w421:dbl)
            n311 = case shown="\"Temperature\"" w405 {
              tunnel: w422 -> [w425 _]
              tunnel: [w425 w426] -> w419
              tunnel: w421 -> [_ w426]
              frame "Resistance", Default {
              }
              frame "Temperature" {
              }
            }
            "T controlled" <- w419
            n312 = local read "DoPID"() -> (w420:refnum<user-event>)
            n313 = Bundle(w419, w408) -> (w418:cluster{dbl, dbl})  [unwired: 1 in]
            n314 = Generate User Event(user event=w420, event data cluster=w418) -> ()  [unwired: 2 in, 2 out]
            n315 = local write "Units"(T3 {"AVS Name 0"="O\u0000h\u0000m\u0000\u0000\u0000\u0000\u0000\u0000\u0000\u0000\u0000\u0000\u0000\u0000\u0000\u0000\u0000", "AVS Name 1"="O\u0000h\u0000m\u0000\u0000\u0000\u0000\u0000\u0000\u0000\u0000\u0000\u0000\u0000\u0000\u0000\u0000\u0000", "AVS Name 2"="O\u0000h\u0000m\u0000\u0000\u0000\u0000\u0000\u0000\u0000\u0000\u0000\u0000\u0000\u0000\u0000\u0000\u0000", "AVS Name 3"="O\u0000h\u0000m\u0000\u0000\u0000\u0000\u0000\u0000\u0000\u0000\u0000\u0000\u0000\u0000\u0000\u0000\u0000", "AVS Name 4"="O\u0000h\u0000m\u0000\u0000\u0000\u0000\u0000\u0000\u0000\u0000\u0000\u0000\u0000\u0000\u0000\u0000\u0000", "AVS Name 5"="O\u0000h\u0000m\u0000\u0000\u0000\u0000\u0000\u0000\u0000\u0000\u0000\u0000\u0000\u0000\u0000\u0000\u0000", "AVS Name 6"="O\u0000h\u0000m\u0000\u0000\u0000\u0000\u0000\u0000\u0000\u0000\u0000\u0000\u0000\u0000\u0000\u0000\u0000", "AVS Name 7"="O\u0000h\u0000m\u0000\u0000\u0000\u0000\u0000\u0000\u0000\u0000\u0000\u0000\u0000\u0000\u0000\u0000\u0000", "AVS Name 8"="O\u0000h\u0000m\u0000\u0000\u0000\u0000\u0000\u0000\u0000\u0000\u0000\u0000\u0000\u0000\u0000\u0000\u0000", "AVS Name 9"="O\u0000h\u0000m\u0000\u0000\u0000\u0000\u0000\u0000\u0000\u0000\u0000\u0000\u0000\u0000\u0000\u0000\u0000"} ("Units")) -> ()
          }
          frame #1 {
            # "Save data to log file"
            n316 = local read "Calib path"() -> (w444:path)
            n317 = local read "Log path"() -> (w443:path)
            n318 = call <vilib>:"Check if File or Folder Exists.vi"("path"=w443) -> ("file or folder exists?"=w435:bool, "dup path"=w436:path)  [unwired: 8 in, 1 out]
            n319 = case shown="False" w435 {
              tunnel: w436 -> [w472 w479]
              tunnel: [w472 w479] -> w437
              frame False {
                n320 = control-ref of="Thermometer"() -> (w475:refnum<vi>)
                n321 = property on="Run description" class="Str"() -> ("Value"=w471:string)  [unwired: 2 in, 2 out]
                n322 = Cluster To Array(cluster="AVS names") -> (array=w477:string[])
                n323 = Cluster To Array(cluster="CS Names") -> (array=w478:string[])
                n324 = call "Format log file header A.vi"("Run description"=w471, "CS Names"=w478, "AVS names"=w477, "Thermometer"=w475) -> ("String"=w473:string)
                n325 = Write to Text File(file (use dialog)=w472, text=w473) -> ()  [unwired: 2 in, 3 out]
              }
              frame True {
              }
            }
            n326 = property on="Data logging" class="Clust (strict)"() -> ("Value"=w458:T22)  [unwired: 2 in, 2 out]
            n327 = Unbundle By Name(w458) -> ("Delimeter"=w459:string, "Date/Time Format"=w457:string)
            n328 = Get Date/Time In Seconds() -> (seconds since 1Jan1904=w450:timestamp)
            n329 = To Double Precision Float(number=w450) -> (double precision float=w448:dbl)
            n330 = call "File Info__ogtk.vi"("file"=w437) -> ("file info"=w433:T38, "file out"=w442:path)  [unwired: 5 in, 1 out]
            n331 = Unbundle By Name(w433) -> ("creation date"=w434:u32)
            n332 = Number To Exponential String(number=w448, precision (6)=i16 10) -> (E-format string=w449:string)  [unwired: 2 in]
            n333 = Format Date/Time String(time format string (%c)=w457, seconds (now)=w450) -> (date/time string=w454:string)  [unwired: 1 in]
            n334 = Number To Fractional String(number=w429) -> (F-format string=w456:string[])  [unwired: 3 in]
            n335 = Number To Fractional String(number=w428) -> (F-format string=w455:string[])  [unwired: 3 in]
            n336 = Number To Fractional String(number=w427) -> (F-format string=w453:string[])  [unwired: 3 in]
            n337 = property on="NewFevery" class="DigNum (strict)"() -> ("Value"=w438:u32)  [unwired: 2 in, 2 out]
            n338 = property on="Time Units" class="Enum (strict)"() -> ("Value"=w439:enum16{"Minutes", "Hours", "Days"})  [unwired: 2 in, 2 out]
            n339 = To Time Stamp(1:w434) -> (0:w440:timestamp)
            n340 = Build Array (concatenate)(w454, w449, w456, w455, w453) -> (w452:string[])
            n341 = call "Time Elapsed time.vi"("Time Units"=w439, "Delay Time"=w438, "Time Old In"=w440) -> ("T>dT?"=w441:bool)  [unwired: 2 out]
            n342 = case shown="True" w441 {
              tunnel: [w461 w464] -> w432
              tunnel: [w460 w465] -> _
              tunnel: w442 -> [w461 _]
              tunnel: w444 -> [w460 _]
              frame False {
              }
              frame True {
                n343 = local read "Data logging"() -> (w466:T22)
                n344 = Unbundle By Name(w466) -> ("Run description"=w462:string, "AVS_Path"=w470:path, "AVS_FName"=w468:string, "CAL_FName"=w469:string, "Filenames suffix"=w467:string)
                n345 = call "MGI Make String Filesafe.vi"("String In"=w462) -> ("Filesafe String Out"=w463:string)
                n346 = call "GeneratePaths.vi"("Filename Suffix"=w467, "Run description"=w463, "AVS_Path"=w470, "AVS_FName"=w468, "CAL_Path"=w470, "CAL_FName"=w469) -> ("Generated Log path"=w464:path, "Generated Calib path"=w465:path)  [unwired: 8 in]
                n347 = local write "Calib path"(w465) -> ()
                n348 = property on="Log path" class="Path"("Val(Sgnl)"=w464) -> ()  [unwired: 2 in, 2 out]
              }
            }
            n349 = call "TC_to_DSC.vi"("Enum"=enum16{"CF", "MNK"}."MNK", "I"=w427, "T"=w428, "R"=w429) -> ()  [unwired: 8 in]
            n350 = call "Write To Spreadsheet File (string) w Error.vi"("delimiter (\\t)"=w459, "append to file? (new file:F)"=TRUE, "1D data"=w452, "file path (dialog if empty)"=w432) -> ("error out"=w446:errorcluster)  [unwired: 6 in, 1 out]
            n351 = Merge Errors(w446, w431) -> (w445:errorcluster)
          }
        }
      }
      event User Event {
        # "Process data from the zBridge bridge"
        n352 = event-data() -> ("R"=w486:dbl[], "T"=w485:dbl[])  [unwired: 1 in, 4 out]
        n353 = local read "zBridge params/Error"() -> (w481:string)
        n354 = local read "zBridge set nr."() -> (w487:u8)
        n355 = property on="All I" class="Arr (strict)"() -> ("Value"=w484:dbl[])  [unwired: 2 in, 2 out]
        n356 = local read "Unit"() -> (w482:string)
        n357 = stacked-sequence {
          tunnel: w481 -> [w513 _]
          tunnel: w487 -> [w496 w523]
          tunnel: w486 -> [w495 w549]
          tunnel: w485 -> [w494 w548]
          tunnel: w484 -> [_ w547]
          tunnel: w483 -> [_ w546]
          tunnel: [_ w545] -> w480
          tunnel: w482 -> [w499 _]
          frame #0 {
            # "Only do PID after measuring\non selected channel"
            n358 = local read "zBridge params"() -> (w498:T3)
            n359 = local read "Units"() -> (w500:T3)
            n360 = Cluster To Array(cluster=w500) -> (array=w503:string[])
            n361 = Cluster To Array(cluster=w498) -> (array=w514:string[])
            n362 = Replace Array Subset(array=w503, new element=w499, index=w496) -> (w502:string[])
            n363 = Replace Array Subset(array=w514, new element=w513, index=w496) -> (w515:string[])
            n364 = Array To Cluster(array=w502) -> (cluster=→"Units":T39)
            n365 = Array To Cluster(array=w515) -> (cluster=→"zBridge params":T40)
            n366 = property on="AVS Runtime Settings" class="Clust (strict)"() -> ("Value"=w507:T12)  [unwired: 2 in, 2 out]
            n367 = Unbundle By Name(w507) -> ("Y_max"=w510:dbl, "Y_min"=w509:dbl, "Filter graphs:"=w508:bool)
            n368 = local read "Data"() -> (w504:cluster{"R":dbl[], "T":dbl[], "Time":dbl[]}[])
            n369 = property on="FB on" class="Enum (strict)"() -> ("Value"=w488:enum16{"Resistance", "Temperature"})  [unwired: 2 in, 2 out]
            n370 = property on="AVS Channel" class="DigNum (strict)"() -> ("Value"=w489:i32)  [unwired: 2 in, 2 out]
            n371 = property on="Data Memory" class="DigNum (strict)"() -> ("Value"=w512:u16)  [unwired: 2 in, 2 out]
            n372 = Get Date/Time In Seconds() -> (seconds since 1Jan1904=w506:timestamp)
            n373 = To Double Precision Float(number=w506) -> (double precision float=w491:dbl)
            n374 = Index Array(array=w495, index=w489) -> (element=w492:dbl)
            n375 = Index Array(array=w494, index=w489) -> (element=w493:dbl)
            n376 = call "Manage Data Arrays - zBridge.vi"("Y_max"=w510, "Y_min"=w509, "Filter Graph Results"=w508, "Append New Data"=TRUE, "Data In"=w504, "Curr R"=w495, "Curr T"=w494, "Curr Time"=w491, "Channel"=w496, "Data Memory"=w512) -> ("Data Out"=w505:cluster{"R":dbl[], "T":dbl[], "Time":dbl[]}[])  [unwired: 9 in]
            n377 = case shown="\"Resistance\", Default" w488 {
              tunnel: w493 -> [_ w518]
              tunnel: w492 -> [w517 _]
              tunnel: [w517 w518] -> w490
              frame "Resistance", Default {
              }
              frame "Temperature" {
              }
            }
            n378 = local write "Data"(w505) -> ()
            n379 = Equal?(x=w496, y=w489) -> (x = y?=w497:bool)
            n380 = case shown="True" w497 {
              tunnel: w490 -> [_ w520]
              tunnel: w491 -> [_ w519]
              frame False {
              }
              frame True {
                n381 = local read "DoPID"() -> (w522:refnum<user-event>)
                n382 = Bundle(w520, w519) -> (w521:cluster{dbl, dbl})  [unwired: 1 in]
                n383 = Generate User Event(user event=w522, event data cluster=w521) -> ()  [unwired: 2 in, 2 out]
              }
            }
            n384 = property on="T controlled" class="DigNum (strict)"("Value"=w490) -> ()  [unwired: 2 in, 2 out]
          }
          frame #1 {
            n385 = local read "Log path"() -> (w526:path)
            n386 = local read "Calib path"() -> (w543:path)
            n387 = call "Strip Path Extension - Path__ogtk.vi"("path"=w526) -> ("root"=w527:string, "extension"=w530:string)
            n388 = Format Into String(format string="_%d", initial string=w527, w523) -> (resulting string=w528:string)  [unwired: 1 in, 1 out]
            n389 = local read "Data logging"() -> (w544:T22)
            n390 = Concatenate Strings(w528, "." ("string"), w530) -> (w525:string)
            n391 = String To Path(string=w525) -> (path=w524:path)
            n392 = call <vilib>:"Check if File or Folder Exists.vi"("path"=w524) -> ("file or folder exists?"=w535:bool, "dup path"=w536:path)  [unwired: 8 in, 1 out]
            n393 = Unbundle By Name(w544) -> ("Delimeter"=w562:string, "Date/Time Format"=w561:string)
            n394 = case shown="False" w535 {
              tunnel: w536 -> [w579 w582]
              tunnel: [w579 w582] -> w537
              frame False {
                n395 = local read "AVS names"() -> (w578:T3)
                n396 = local read "CS Names"() -> (w577:T15)
                n397 = control-ref of="Thermometer"() -> (w581:refnum<vi>)
                n398 = property on="Run description" class="Str"() -> ("Value"=w574:string)  [unwired: 2 in, 2 out]
                n399 = Cluster To Array(cluster=w578) -> (array=w575:string[])
                n400 = Cluster To Array(cluster=w577) -> (array=w576:string[])
                n401 = call "Format log file header Z.vi"("Run description"=w574, "CS Names"=w576, "AVS names"=w575, "Thermometer"=w581) -> ("String"=w580:string)
                n402 = Write to Text File(file (use dialog)=w579, text=w580) -> ()  [unwired: 2 in, 3 out]
              }
              frame True {
              }
            }
            n403 = Get Date/Time In Seconds() -> (seconds since 1Jan1904=w554:timestamp)
            n404 = To Double Precision Float(number=w554) -> (double precision float=w552:dbl)
            n405 = Number To Exponential String(number=w552, precision (6)=i16 10) -> (E-format string=w553:string)  [unwired: 2 in]
            n406 = Format Date/Time String(time format string (%c)=w561, seconds (now)=w554) -> (date/time string=w558:string)  [unwired: 1 in]
            n407 = Number To Exponential String(number=w549) -> (E-format string=w560:string[])  [unwired: 3 in]
            n408 = Number To Engineering String(4:w548) -> (0:w559:string[])  [unwired: 3 in]
            n409 = Number To Fractional String(number=w547) -> (F-format string=w557:string[])  [unwired: 3 in]
            n410 = call "File Info__ogtk.vi"("file"=w537) -> ("file info"=w533:T38, "file out"=w542:path)  [unwired: 5 in, 1 out]
            n411 = Unbundle By Name(w533) -> ("creation date"=w534:u32)
            n412 = Build Array (concatenate)(w558, w553, w560, w559, w557) -> (w556:string[])
            n413 = property on="NewFevery" class="DigNum (strict)"() -> ("Value"=w538:u32)  [unwired: 2 in, 2 out]
            n414 = property on="Time Units" class="Enum (strict)"() -> ("Value"=w539:enum16{"Minutes", "Hours", "Days"})  [unwired: 2 in, 2 out]
            n415 = To Time Stamp(1:w534) -> (0:w540:timestamp)
            n416 = call "Time Elapsed time.vi"("Time Units"=w539, "Delay Time"=w538, "Time Old In"=w540) -> ("T>dT?"=w541:bool)  [unwired: 2 out]
            n417 = case shown="True" w541 {
              tunnel: [w564 w567] -> w532
              tunnel: [w563 w569] -> _
              tunnel: w542 -> [w564 _]
              tunnel: w543 -> [w563 _]
              frame False {
              }
              frame True {
                n418 = local read "Data logging"() -> (w570:T22)
                n419 = Unbundle By Name(w570) -> ("Run description"=w566:string, "Filenames suffix"=w568:string, "AVS_Path"=w573:path, "AVS_FName"=w571:string, "CAL_FName"=w572:string)
                n420 = call "MGI Make String Filesafe.vi"("String In"=w566) -> ("Filesafe String Out"=w565:string)
                n421 = call "GeneratePaths.vi"("Filename Suffix"=w568, "Run description"=w565, "AVS_Path"=w573, "AVS_FName"=w571, "CAL_Path"=w573, "CAL_FName"=w572) -> ("Generated Log path"=w567:path, "Generated Calib path"=w569:path)  [unwired: 8 in]
                n422 = local write "Calib path"(w569) -> ()
                n423 = property on="Log path" class="Path"("Val(Sgnl)"=w567) -> ()  [unwired: 2 in, 2 out]
              }
            }
            n424 = call "Write To Spreadsheet File (string) w Error.vi"("delimiter (\\t)"=w562, "append to file? (new file:F)"=TRUE, "1D data"=w556, "file path (dialog if empty)"=w532) -> ("error out"=w550:errorcluster)  [unwired: 6 in, 1 out]
            n425 = Merge Errors(w550, w546) -> (w545:errorcluster)
          }
        }
      }
      event User Event {
        # "Current source automatic mode"
        # "Check if PID error (SP-PV)==0"
        # "Check if temperature\nis stabilized"
        # "Check if any channel\nis in automatic mode"
        # "Check if stabilization delay time \nis elapsed"
        # "T sabilized?"
        # "If TCS auto mode enabled and temperature is not changing => fire TempStabilized event to save log and set new CS point. Otherwise do PID (if enabled)."
        n426 = event-data() -> ("R/T"=w592:dbl, "Time"=w593:dbl)  [unwired: 1 in, 4 out]
        n427 = local read "I_list[i]"() -> (w586:dbl[])
        n428 = local read "Error"() -> (w596:dbl)
        n429 = property on="N averages" class="DigNum (strict)"() -> ("Value"=w589:i32)  [unwired: 2 in, 2 out]
        n430 = property on="FB to" class="Enum (strict)"() -> ("Value"=w585:enum16{"0", "1", "2", "3"})  [unwired: 2 in, 2 out]
        n431 = local read "Time Old"() -> (w602:dbl)
        n432 = local read "Mode"() -> (w584:enum16{"Manual", "Automatic"})
        n433 = property on="T stability" class="DigNum (strict)"() -> ("Value"=w587:dbl)  [unwired: 2 in, 2 out]
        n434 = Equal To 0?(x=w596) -> (x = 0?=w594:bool)
        n435 = property on="Delay Time" class="DigNum (strict)"() -> ("Value"=w588:dbl)  [unwired: 2 in, 2 out]
        n436 = Index Array(array=w586, index=w585) -> (element=w603:dbl)
        n437 = Not Equal To 0?(x=w584) -> (x != 0?=w583:bool)
        n438 = call "Derivatives Pt by Pt.vi"("Points to avg"=w589, "accuracy (%)"=w587, "Time"=w593, "Data"=w592) -> ("Stable?"=w595:bool, "Stability (%)"=→"Slope":dbl, "dt (s)"=w599:dbl)  [unwired: 3 in]
        n439 = call "Time Elapsed dbl.vi"("Delay Time"=w588, "Time Old In"=w602) -> ("T>dT?"=w591:bool, "Delta T"=→"Timer":dbl, "Time New Out"=w601:dbl)  [unwired: 1 in]
        n440 = Compound Arithmetic op=AND(w591, w583, w594, w595) -> (w597:bool)
        "SP reached?" <- w597
        n441 = property on="I3 as temp 2" class="Bool (strict)"() -> ("Value"=w590:bool)  [unwired: 2 in, 2 out]
        n442 = case shown="True" w597 {
          tunnel: w601 -> [_ w620]
          tunnel: w599 -> [w618 _]
          tunnel: w592 -> [w612 _]
          tunnel: w590 -> [w610 _]
          tunnel: w603 -> [w611 _]
          tunnel: w586 -> [w607 _]
          tunnel: w585 -> [w606 _]
          tunnel: w583 -> [w604 _]
          frame False {
            # "Temperature is not stable. If enabled, do PID regulation"
            n443 = And(x=w610, y=w604) -> (x .and. y?=w605:bool)
            n444 = local read "PID setup 2"() -> (w615:T27)
            n445 = property on="I3" class="DigNum (strict)"() -> ("Value"=w616:dbl)  [unwired: 2 in, 2 out]
            n446 = call "PID control incremental.vi"("Process Variable"=w612, "dt"=w618, "Setpoint"=w611, "PID Settings"=w615, "I in"=w616, "PID Enabled"=w605) -> ("err out"=→"Error":dbl, "int out"=→"Int":dbl, "I out"=w609:dbl)  [unwired: 10 in, 1 out]
            n447 = Bundle("Numeric"=w611, "R/T"=w612) -> (→"SP":cluster{"Numeric":dbl, "R/T":dbl})  [unwired: 1 in]
            n448 = Replace Array Subset(array=w607, new element=w609, index=w606) -> (→"I 2":dbl[])
          }
          frame True {
            # "Temperature is stable & automode is on"
            n449 = case shown="False" "Call external VI" {
              tunnel: w620 -> [w623 _]
              frame False {
                # "External VI call disabled -> proceed\nwith automode"
                n450 = local write "Time Old"(w623) -> ()
                n451 = property on="TempStabilized" class="TypRef (strict)"() -> ("Value"=w622:refnum<user-event>)  [unwired: 2 in, 2 out]
                n452 = Generate User Event(user event=w622, event data cluster=TRUE ("event data")) -> ()  [unwired: 2 in, 2 out]
              }
              frame True {
                # "Call external VI"
                n453 = property on="CallExtVI" class="TypRef (strict)"() -> ("Value"=w624:refnum<user-event>)  [unwired: 2 in, 2 out]
                n454 = Generate User Event(user event=w624, event data cluster="" ("event data")) -> ()  [unwired: 2 in, 2 out]
              }
            }
          }
        }
      }
      event User Event {
        n455 = event-data() -> ()  [unwired: 1 in, 5 out]
        n456 = local read "vi reference"() -> (w629:refnum<vi>)
        n457 = call "GetExtVIStatus.vi"("vi reference in"=w629) -> ("vi reference out"=w626:refnum<vi>, "Exec.State"=w628:T25, "Finished?"=w627:bool)
        n458 = case shown="\"Idle\"" w628 {
          tunnel: w627 -> [_ _]
          tunnel: w626 -> [_ w630]
          frame "Bad", Default {
          }
          frame "Idle" {
            n459 = local read "VI called?"() -> (w631:bool)
            n460 = case shown="True" w631 {
              tunnel: w630 -> [w633 _]
              frame False {
                n461 = property on="Data array" class="Arr (strict)"() -> ("Value"=w636:dbl[])  [unwired: 2 in, 2 out]
                n462 = property on="T_array" class="Arr (strict)"() -> ("Value"=w637:dbl[])  [unwired: 2 in, 2 out]
                n463 = property on="I" class="Arr (strict)"() -> ("Value"=w638:dbl[])  [unwired: 2 in, 2 out]
                n464 = Format Date/Time String() -> (date/time string=w635:string)  [unwired: 3 in]
                n465 = Bundle("date/time string"=w635, "Value"=w636, "Value"=w637, "Value"=w638) -> (w634:T41)  [unwired: 1 in]
                n466 = call "CallExtVI.vi"("vi reference in"=w633, "Cluster"=w634) -> ()  [unwired: 1 out]
                "VI called?" <- TRUE ("VI called?")
              }
              frame True {
                n467 = property on="TempStabilized" class="TypRef (strict)"() -> ("Value"=w640:refnum<user-event>)  [unwired: 2 in, 2 out]
                n468 = Get Date/Time In Seconds() -> (seconds since 1Jan1904=w641:timestamp)
                n469 = To Double Precision Float(number=w641) -> (double precision float=w642:dbl)
                n470 = Generate User Event(user event=w640, event data cluster=TRUE ("event data")) -> ()  [unwired: 2 in, 2 out]
                n471 = local write "Time Old"(w642) -> ()
              }
            }
          }
        }
      }
      event User Event {
        # "CS automode\nT is stabilized"
        n472 = event-data() -> ("TempStabilized"=w643:bool)  [unwired: 1 in, 4 out]
        n473 = stacked-sequence {
          tunnel: w645 -> [w648 _]
          tunnel: [w649 _] -> w644
          tunnel: w643 -> [_ w657]
          frame #0 {
            # "Step1: Save R,T,I values to calibration file"
            n474 = property on="Data logging" class="Clust (strict)"() -> ("Value"=w652:T22)  [unwired: 2 in, 2 out]
            n475 = Unbundle By Name(w652) -> ("Date/Time Format"=w653:string, "Delimeter"=w650:string)
            n476 = local write "VI called?"(FALSE ("VI called?")) -> ()
            n477 = property on="R" class="Clust (strict)"() -> ("Value"=w651:T6)  [unwired: 2 in, 2 out]
            n478 = property on="T" class="Clust (strict)"() -> ("Value"=w655:T2)  [unwired: 2 in, 2 out]
            n479 = property on="I" class="Arr (strict)"() -> ("Value"=w654:dbl[])  [unwired: 2 in, 2 out]
            n480 = property on="Calib path" class="Path"() -> ("Value"=w656:path)  [unwired: 2 in, 2 out]
            n481 = call "Write to cal log file.vi"("Value 2"=w654, "Date/Time Format"=w653, "Value 3"=w655, "Value"=w651, "Delimeter"=w650, "Value 4"=w656) -> ("error out"=w647:errorcluster)  [unwired: 1 out]
            n482 = Merge Errors(w647, w648) -> (w649:errorcluster)
          }
          frame #1 {
            # "Step 2: Sweep through the currents list"
            n483 = case shown="True" w657 {
              frame False {
              }
              frame True {
                n484 = local read "I_list_idx_max"() -> (w659:i32)
                n485 = local read "I_list_idx"() -> (w660:i32)
                n486 = Less?(x=w660, y=w659) -> (x < y?=w658:bool)
                n487 = case shown="False" w658 {
                  frame False {
                    n488 = property on="Mode" class="Enum (strict)"("Val(Sgnl)"=enum16{"Manual", "Automatic"}."Manual" ("Value (Signaling)")) -> ()  [unwired: 2 in, 2 out]
                  }
                  frame True {
                    n489 = property on="I_next" class="Bool (strict)"("Val(Sgnl)"=TRUE) -> ()  [unwired: 2 in, 2 out]
                  }
                }
              }
            }
          }
        }
      }
      event User Event {
        # "Disable controls for disabled channels"
        n490 = event-data() -> ()  [unwired: 1 in, 5 out]
        n491 = property on="AVS type" class="Enum (strict)"() -> ("Value"=w667:T30)  [unwired: 2 in, 2 out]
        n492 = case shown="\"AVS47B (RS232 interface)\"" w667 {
          tunnel: [w677 w688 w697] -> w666
          frame Default {
            n493 = property on="AVS Runtime Settings" class="Clust (strict)"() -> ("Value"=w681:T12)  [unwired: 2 in, 2 out]
            n494 = Unbundle By Name(w681) -> ("Read AVS channels from"=w679:i8, "Last Channel"=w680:i8)
            n495 = for {
              N: 10 -> [_]
              tunnel: w680 -> [w683]
              tunnel: w679 -> [w684]
              tunnel: [w682] -> w677 mode=indexing
              i -> [w685]
              n496 = Less Or Equal?(x=w684, y=w685) -> (x <= y?=w687:bool)
              n497 = Less Or Equal?(x=w685, y=w683) -> (x <= y?=w686:bool)
              n498 = And(x=w687, y=w686) -> (x .and. y?=w682:bool)
            }
          }
          frame "Impedance Bridge" {
            n499 = local read "zDll"() -> (w689:path)
            n500 = for {
              N: 10 -> [_]
              tunnel: [w692] -> w690 mode=indexing
              tunnel: w689 -> [w693]
              i -> [w695]
              n501 = call "GetByteParam.vi"("ParNo"=u8 0, "SetNo"=w695, "zDll"=w693) -> ("return type"=w692:u8)  [unwired: 6 in, 2 out]
            }
            n502 = Greater Than 0?(x=w690) -> (x > 0?=w688:bool[])
          }
          frame "AVS47B (RS232 interface)" {
            n503 = local read "Active"() -> (w696:T10)
            n504 = Cluster To Array(cluster=w696) -> (array=w697:bool[])
          }
        }
        n505 = control-ref of="Active"() -> (w673:refnum<vi>)
        n506 = control-ref of="Exc&Ranges"() -> (w669:refnum<vi>)
        n507 = control-ref of="R"() -> (w674:refnum<vi>)
        n508 = control-ref of="Thermometer"() -> (w675:refnum<vi>)
        n509 = control-ref of="T"() -> (w676:refnum<vi>)
        n510 = control-ref of="uPlots"() -> (w670:refnum<vi>)
        n511 = control-ref of="AVS names"() -> (w668:refnum<vi>)
        n512 = control-ref of="zBridge params"() -> (w665:refnum<vi>)
        n513 = control-ref of="Status"() -> (w664:refnum<vi>)
        n514 = control-ref of="Units"() -> (w663:refnum<vi>)
        n515 = Build Array(w673, w669, w674, w675, w676, w670, w668, w665, w664, w663) -> (w671:refnum<vi>[])
        n516 = Array Size(array=w671) -> (size(s)=w672:i32)
        n517 = for {
          N: w672 -> [_]
          tunnel: w671 -> [w701] mode=indexing
          tunnel: w666 -> [w698]
          n518 = property class="Clust"(reference=w701) -> ("Controls[]"=w699:refnum<vi>[])  [unwired: 1 in, 2 out]
          n519 = Array Size(array=w699) -> (size(s)=w700:i32)
          n520 = for {
            N: w700 -> [_]
            tunnel: w699 -> [w703] mode=indexing
            tunnel: w698 -> [w702] mode=indexing
            n521 = case shown="True" w702 {
              tunnel: w703 -> [w704 w709]
              frame False {
                n522 = property class="Ctl"(reference=w704, "Disabled"=u8 2) -> ("ClassName"=w705:string)  [unwired: 1 in, 2 out]
                n523 = case shown="\"Boolean\"" w705 {
                  tunnel: w704 -> [_ w708 _]
                  frame "False", Default {
                  }
                  frame "Boolean" {
                    n524 = property class="Ctl"(reference=w708, "Value"=FALSE) -> ()  [unwired: 1 in, 2 out]
                  }
                  frame "Ring" {
                  }
                }
              }
              frame True {
                n525 = property class="Ctl"(reference=w709, "Disabled"=u8 0) -> ("ClassName"=w710:string)  [unwired: 1 in, 2 out]
                n526 = case shown="\"Boolean\"" w710 {
                  tunnel: w709 -> [_ w713]
                  frame "False", Default {
                  }
                  frame "Boolean" {
                    n527 = property class="Ctl"(reference=w713, "Value"=TRUE) -> ()  [unwired: 1 in, 2 out]
                  }
                }
              }
            }
          }
        }
      }
      event "Log path": Value Change {
        # "Modify window title to show measurement information"
        n528 = event-data() -> ("NewVal"=w720:path)  [unwired: 1 in, 5 out]
        n529 = property on="Run description" class="Str"() -> ("Value"=w714:string)  [unwired: 2 in, 2 out]
        n530 = property on="AVS type" class="Enum (strict)"() -> ("RingText.Text"=w715:string)  [unwired: 2 in, 2 out]
        n531 = property on="CS type" class="Enum (strict)"() -> ("RingText.Text"=w718:string)  [unwired: 2 in, 2 out]
        n532 = Path To String(path=w720) -> (string=w717:string)
        n533 = Format Into String(format string="%s - %s - %s   (%s)", w714, w715, w718, w717) -> (resulting string=w716:string)  [unwired: 2 in, 1 out]
        n534 = control-ref of="This VI"() -> (w721:refnum<vi>)
        n535 = property class="VI"(reference=w721, "Front Panel.Title"=w716) -> ()  [unwired: 1 in, 2 out]
      }
      event "Refresh Button", "Bridge settings.AVS_CalFolder": Value Change; User Event {
        # "Refresh the list of calibration files"
        n536 = event-data() -> ()  [unwired: 1 in, 3 out]
        n537 = control-ref of="Thermometer"() -> (w728:refnum<vi>)
        n538 = control-ref of="CurCalibrations"() -> (w722:refnum<vi>)
        n539 = control-ref of="AVS_CalFolder"() -> (w726:refnum<vi>)
        n540 = control-ref of="Select sensor 1"() -> (w727:refnum<vi>)
        n541 = control-ref of="Select sensor 1"() -> (w725:refnum<vi>)
        n542 = call "ReloadCalibrations.vi"("error in (no error)"=w724, "Quick convert sensors"=w725, "CurCalibrations"=w722, "Calibration files path"=w726, "Channel1 sensors"=w727, "Channels list"=w728) -> ("error out"=w723:errorcluster)  [unwired: 1 in]
      }
      event "Mode Buttons": Value Change {
        w734 = refnum<vi> refnum  # XYGraph
        # "Show cursor on plot is \"Cursor\" or \"Delete points\" mode is enabled"
        # "!!NOTE:This routine assumes that XY graph is control #1 on tab page!!"
        n543 = event-data() -> ("NewVal"=w730:T11)  [unwired: 1 in, 5 out]
        n544 = property on="Channel Controls" class="TabCtl (strict)"() -> ("Pages"=w738:refnum<vi>[], "Value"=w737:T1)  [unwired: 2 in, 2 out]
        n545 = Index Array(array=w738, index=w737) -> (element=w736:refnum<vi>)
        n546 = property class="Page"(reference=w736) -> ("ControlsOnPage"=w731:refnum<vi>[])  [unwired: 1 in, 2 out]
        n547 = Index Array(array=w731, index=1) -> (element=w735:refnum<vi>)
        n548 = Type Cast(type=w734, x=w735) -> (*(type *) &x=w729:refnum<vi>)
        n549 = case shown="\"Erase Range\"" w730 {
          tunnel: w729 -> [w739 w748 w756 w764]
          frame "No Selection", Default {
            n550 = property class="XYGraph"(reference=w739, "Active Cursor"=u32 0, "Cursor.Visible"=FALSE) -> (reference out=w742:refnum<vi>)  [unwired: 1 in, 1 out]
            n551 = property class="XYGraph"(reference=w742, "Active Cursor"=u32 1, "Cursor.Visible"=FALSE) -> ()  [unwired: 1 in, 2 out]
          }
          frame "Erase Range" {
            n552 = property class="XYGraph"(reference=w748, "Active Cursor"=u32 0, "Cursor.Visible"=TRUE, "Cursor.Cursor Color"=u32 16777062, "Cursor.Cursor Index"=0, "ActPaletteTool"=0 ("Palette:Active Tool")) -> (reference out=w751:refnum<vi>)  [unwired: 1 in, 1 out]
            n553 = property class="XYGraph"(reference=w751, "Active Cursor"=u32 1, "Cursor.Visible"=TRUE, "Cursor.Cursor Color"=u32 6618880) -> ()  [unwired: 1 in, 2 out]
          }
          frame "Cursor Mode" {
            n554 = property class="XYGraph"(reference=w756, "Active Cursor"=u32 0, "Cursor.Visible"=TRUE, "Cursor.Cursor Color"=u32 6618880, "ActPaletteTool"=0 ("Palette:Active Tool")) -> (reference out=w759:refnum<vi>)  [unwired: 1 in, 1 out]
            n555 = property class="XYGraph"(reference=w759, "Active Cursor"=u32 1, "Cursor.Visible"=FALSE) -> ()  [unwired: 1 in, 2 out]
          }
          frame "Erase point" {
            n556 = property class="XYGraph"(reference=w764, "Active Cursor"=u32 0, "Cursor.Visible"=TRUE, "Cursor.Cursor Color"=u32 16777062, "ActPaletteTool"=0 ("Palette:Active Tool")) -> (reference out=w767:refnum<vi>)  [unwired: 1 in, 1 out]
            n557 = property class="XYGraph"(reference=w767, "Active Cursor"=u32 1, "Cursor.Visible"=FALSE) -> ()  [unwired: 1 in, 2 out]
          }
        }
      }
      event "Log 0", "Log 1", "Log 2", "Log 3", "Log 4", "Log 5", "Log 6", "Log 7", "Log 8", "Log 9": Value Change {
        w776 = refnum<vi> refnum  # XYGraph
        # "!!NOTE:This routine assumes that XY graph is control #1 on tab page!!"
        # "Toggle logarithmic scale for Y-axis on plot"
        n558 = event-data() -> ("NewVal"=w774:bool)  [unwired: 1 in, 5 out]
        n559 = property on="Channel Controls" class="TabCtl (strict)"() -> ("Pages"=w781:refnum<vi>[], "Value"=w780:T1)  [unwired: 2 in, 2 out]
        n560 = Index Array(array=w781, index=w780) -> (element=w779:refnum<vi>)
        n561 = property class="Page"(reference=w779) -> ("ControlsOnPage"=w778:refnum<vi>[])  [unwired: 1 in, 2 out]
        n562 = Index Array(array=w778, index=1) -> (element=w777:refnum<vi>)
        n563 = Type Cast(type=w776, x=w777) -> (*(type *) &x=w775:refnum<vi>)
        n564 = Boolean To (0,1)(Boolean=w774) -> (0, 1=w773:i16)
        n565 = property class="XYGraph"(reference=w775, "YScale.Mapping Mode"=w773) -> ()  [unwired: 1 in, 2 out]
      }
      event "R-Plot 0", "R-Plot 1", "R-Plot 2", "R-Plot 3", "R-Plot 4", "R-Plot 5", "R-Plot 6", "R-Plot 7", "R-Plot 8", "R-Plot 9": Mouse Down? {
        # "Disabled"
        n566 = event-data() -> ("CtlRef"=w783:refnum<vi>, "Button"=w788:u16, "Mods.Double Click"=w785:bool)  [unwired: 1 in, 5 out]
        n567 = Equal?(x=u16 1, y=w788) -> (x = y?=w786:bool)
        n568 = And(x=w786, y=w785) -> (x .and. y?=w784:bool)
        n569 = disable-structure shown="Disabled" {
          disable-tunnel: w784 -> [w791 _]
          disable-tunnel: w783 -> [w790 _]
          disable-tunnel: "Mode Buttons" -> [w789 _]
          frame Disabled {
            n570 = case shown="True" w791 {
              tunnel: w789 -> [_ w793]
              tunnel: w790 -> [_ w792]
              frame False {
              }
              frame True {
                n571 = case shown="\"Erase Range\"" w793 {
                  tunnel: w792 -> [_ w794]
                  frame "No Selection", Default {
                  }
                  frame "Erase Range" {
                    n572 = property class="XYGraph (strict)"(reference=w794, "ActPaletteTool"=0 ("Palette:Active Tool"), "Active Cursor"=u32 0, "Cursor.Visible"=TRUE) -> ()  [unwired: 1 in, 2 out]
                  }
                }
              }
            }
          }
          frame Enabled {
          }
        }
        n573 = event-data() -> ()  [unwired: 5 in, 1 out]
      }
      event "R-Plot 0", "R-Plot 1", "R-Plot 2", "R-Plot 3", "R-Plot 4", "R-Plot 5", "R-Plot 6", "R-Plot 7", "R-Plot 8", "R-Plot 9": Mouse Down {
        # "Process (double) click on plots in special modes (\"Cursor\", \"Erase\")"
        n574 = event-data() -> ("CtlRef"=w799:refnum<vi>, "Coords"=w802:T42, "Button"=w798:u16, "Mods.Double Click"=w801:bool)  [unwired: 1 in, 4 out]
        n575 = property on="Mode Buttons" class="RadioBtnsControl (strict)"() -> ("Value"=w800:T11)  [unwired: 2 in, 2 out]
        n576 = case shown="0, Default" w798 {
          tunnel: w802 -> [_ w836]
          tunnel: w801 -> [_ w835]
          tunnel: w800 -> [w807 w834]
          tunnel: w799 -> [w808 w833]
          frame 0, Default {
            n577 = local read "LMB Down"() -> (w805:bool)
            n578 = Equal?(x=w807, y=T11."Erase Range" ("Mode Buttons")) -> (x = y?=w806:bool)
            n579 = And(x=w805, y=w806) -> (x .and. y?=w804:bool)
            n580 = case shown="True" w804 {
              tunnel: w808 -> [_ w831]
              frame False {
              }
              frame True {
                n581 = property class="XYGraph (strict)"(reference=w831, "Active Cursor"=u32 0, "Active Cursor"=u32 1) -> ("Cursor.Cursor X"=w828:dbl, "Cursor.Cursor X"=w809:dbl)  [unwired: 1 in, 2 out]
                n582 = local read "Channel Controls"() -> (w830:T1)
                n583 = local read "Data"() -> (w825:cluster{"R":dbl[], "T":dbl[], "Time":dbl[]}[])
                n584 = Max & Min(x=w828, y=w809) -> (max(x,y)=w818:dbl, min(x,y)=w811:dbl)
                n585 = Index Array(array=w825, index=w830) -> (element=w821:cluster{"R":dbl[], "T":dbl[], "Time":dbl[]})
                n586 = Unbundle By Name(w821) -> ("R"=w819:dbl[], "T"=w820:dbl[], "Time"=w817:dbl[])
                n587 = Threshold 1D Array(2:w818, 3:w817) -> (0:w815:dbl)  [unwired: 1 in]
                n588 = Threshold 1D Array(2:w811, 3:w817) -> (0:w816:dbl)  [unwired: 1 in]
                n589 = Subtract(x=w815, y=w816) -> (x-y=w814:dbl)
                n590 = Delete From Array(array=w819, length=w814, index=w816) -> (array with subset deleted=w824:dbl[])  [unwired: 1 out]
                n591 = Delete From Array(array=w820, length=w814, index=w816) -> (array with subset deleted=w823:dbl[])  [unwired: 1 out]
                n592 = Delete From Array(array=w817, length=w814, index=w816) -> (array with subset deleted=w822:dbl[])  [unwired: 1 out]
                n593 = Bundle By Name(cluster=w821, "R"=w824, "T"=w823, "Time"=w822) -> (w826:cluster{"R":dbl[], "T":dbl[], "Time":dbl[]})
                n594 = Replace Array Subset(array=w825, new element=w826, index=w830) -> (w827:cluster{"R":dbl[], "T":dbl[], "Time":dbl[]}[])
                n595 = local write "Data"(w827) -> ()
                n596 = property class="XYGraph (strict)"(reference=w831, "Active Cursor"=u32 0, "Cursor.Cursor X"=w811, "Active Cursor"=u32 1, "Cursor.Cursor X"=w811) -> ()  [unwired: 1 in, 2 out]
              }
            }
          }
          frame 1 {
            n597 = case shown="\"Erase point\"" w834 {
              tunnel: w833 -> [_ w839 w858 w866]
              tunnel: w836 -> [_ w838 w857 w868]
              tunnel: w835 -> [_ w837 w859 w867]
              frame "No Selection", Default {
              }
              frame "Cursor Mode" {
                n598 = case shown="True" w837 {
                  tunnel: w839 -> [_ w847]
                  tunnel: w838 -> [_ w845]
                  frame False {
                  }
                  frame True {
                    n599 = invoke class="XYGraph (strict)" method="Map Coords To XY"(reference=w847, "Coords"=w845) -> (reference out=w846:refnum<vi>, "XY"=w844:cluster{"X":dbl, "Y":dbl})  [unwired: 5 in, 5 out]
                    n600 = Unbundle By Name(w844) -> ("X"=w840:dbl)
                    n601 = local read "Data"() -> (w841:cluster{"R":dbl[], "T":dbl[], "Time":dbl[]}[])
                    n602 = property class="XYGraph (strict)"(reference=w846, "Active Cursor"=u32 0, "Cursor.Cursor Position"=w844) -> ()  [unwired: 1 in, 2 out]
                    n603 = for {
                      tunnel: w841 -> [w856] mode=indexing
                      tunnel: w840 -> [w854]
                      tunnel: [w850] -> w842 mode=indexing
                      tunnel: [w849] -> w843 mode=indexing
                      n604 = Unbundle By Name(w856) -> ("R"=w853:dbl[], "T"=w852:dbl[], "Time"=w855:dbl[])
                      n605 = Threshold 1D Array(2:w854, 3:w855) -> (0:w851:dbl)  [unwired: 1 in]
                      n606 = Index Array(array=w853, index=w851) -> (element=w850:dbl)
                      n607 = Index Array(array=w852, index=w851) -> (element=w849:dbl)
                    }
                    n608 = property on="Small R" class="Arr (strict)"("Value"=w842) -> ()  [unwired: 2 in, 2 out]
                    n609 = property on="Small T" class="Arr (strict)"("Value"=w843) -> ()  [unwired: 2 in, 2 out]
                    n610 = property on="Time" class="DigNum (strict)"("Value"=w840) -> ()  [unwired: 2 in, 2 out]
                  }
                }
              }
              frame "Erase Range" {
                n611 = case shown="False" w859 {
                  tunnel: w858 -> [w863 _]
                  tunnel: w857 -> [w862 _]
                  frame False {
                    n612 = invoke class="XYGraph (strict)" method="Map Coords To XY"(reference=w863, "Coords"=w862) -> (reference out=w865:refnum<vi>, "XY"=w860:cluster{"X":dbl, "Y":dbl})  [unwired: 5 in, 5 out]
                    n613 = property class="XYGraph (strict)"(reference=w865, "Active Cursor"=u32 0, "Cursor.Cursor Position"=w860, "Active Cursor"=u32 1, "Cursor.Cursor Position"=w860) -> ()  [unwired: 1 in, 2 out]
                  }
                  frame True {
                  }
                }
              }
              frame "Erase point" {
                n614 = case shown="False" w867 {
                  tunnel: w866 -> [w873 w888]
                  tunnel: w868 -> [w872 _]
                  frame False {
                    n615 = invoke class="XYGraph (strict)" method="Map Coords To XY"(reference=w873, "Coords"=w872) -> (reference out=w871:refnum<vi>, "XY"=w870:cluster{"X":dbl, "Y":dbl})  [unwired: 5 in, 5 out]
                    n616 = property class="XYGraph (strict)"(reference=w871, "Active Cursor"=u32 0, "Cursor.Cursor Position"=w870) -> ()  [unwired: 1 in, 2 out]
                  }
                  frame True {
                    n617 = property class="XYGraph (strict)"(reference=w888, "Active Cursor"=u32 0) -> ("Cursor.Cursor X"=w875:dbl)  [unwired: 1 in, 2 out]
                    n618 = local read "Channel Controls"() -> (w874:T1)
                    n619 = local read "Data"() -> (w884:cluster{"R":dbl[], "T":dbl[], "Time":dbl[]}[])
                    n620 = Index Array(array=w884, index=w874) -> (element=w880:cluster{"R":dbl[], "T":dbl[], "Time":dbl[]})
                    n621 = Unbundle By Name(w880) -> ("R"=w876:dbl[], "T"=w877:dbl[], "Time"=w878:dbl[])
                    n622 = Threshold 1D Array(2:w875, 3:w878) -> (0:w879:dbl)  [unwired: 1 in]
                    n623 = Delete From Array(array=w876, index=w879) -> (array with subset deleted=w883:dbl[])  [unwired: 1 in, 1 out]
                    n624 = Delete From Array(array=w877, index=w879) -> (array with subset deleted=w882:dbl[])  [unwired: 1 in, 1 out]
                    n625 = Delete From Array(array=w878, index=w879) -> (array with subset deleted=w881:dbl[])  [unwired: 1 in, 1 out]
                    n626 = Bundle By Name(cluster=w880, "R"=w883, "T"=w882, "Time"=w881) -> (w885:cluster{"R":dbl[], "T":dbl[], "Time":dbl[]})
                    n627 = Replace Array Subset(array=w884, new element=w885, index=w874) -> (w886:cluster{"R":dbl[], "T":dbl[], "Time":dbl[]}[])
                    n628 = local write "Data"(w886) -> ()
                  }
                }
              }
            }
            "LMB Down" <- TRUE ("Mouse down")
          }
        }
      }
      event "R-Plot 0", "R-Plot 1", "R-Plot 2", "R-Plot 3", "R-Plot 4", "R-Plot 5", "R-Plot 6", "R-Plot 7", "R-Plot 8", "R-Plot 9": Mouse Move {
        # "Process mouse movement over plots in special modes (\"Cursor\", \"Erase\")"
        n629 = event-data() -> ("CtlRef"=w889:refnum<vi>, "Coords"=w890:T42)  [unwired: 1 in, 3 out]
        n630 = property on="Mode Buttons" class="RadioBtnsControl (strict)"() -> ("Value"=w894:T11)  [unwired: 2 in, 2 out]
        n631 = local read "LMB Down"() -> (w895:bool)
        n632 = Equal?(x=w894, y=T29."Erase Range") -> (x = y?=w891:bool)
        n633 = And(x=w895, y=w891) -> (x .and. y?=w892:bool)
        n634 = case shown="True" w892 {
          tunnel: w890 -> [_ w897]
          tunnel: w889 -> [_ w896]
          frame False {
          }
          frame True {
            n635 = invoke class="XYGraph (strict)" method="Map Coords To XY"(reference=w896, "Coords"=w897) -> (reference out=w900:refnum<vi>, "XY"=w899:cluster{"X":dbl, "Y":dbl})  [unwired: 5 in, 5 out]
            n636 = property class="XYGraph (strict)"(reference=w900, "Active Cursor"=u32 1, "Cursor.Cursor Position"=w899) -> ()  [unwired: 1 in, 2 out]
          }
        }
      }
      event "R-Plot 0", "R-Plot 1", "R-Plot 2", "R-Plot 3", "R-Plot 4", "R-Plot 5", "R-Plot 6", "R-Plot 7", "R-Plot 8", "R-Plot 9": Mouse Up {
        n637 = event-data() -> ("CtlRef"=w903:refnum<vi>, "Button"=w901:u16)  [unwired: 1 in, 6 out]
        n638 = property on="Mode Buttons" class="RadioBtnsControl (strict)"() -> ("Value"=w904:T11)  [unwired: 2 in, 2 out]
        n639 = property class="XYGraph (strict)"(reference=w903) -> ("ActPaletteTool"=w902:i32)  [unwired: 1 in, 2 out]
        n640 = case shown="1" w901 {
          tunnel: w904 -> [_ w908]
          tunnel: w903 -> [_ w907]
          tunnel: w902 -> [_ w906]
          frame 0, Default {
          }
          frame 1 {
            n641 = case shown="Default" w906 {
              tunnel: w908 -> [_ _]
              tunnel: w907 -> [_ _]
              frame Default {
                n642 = property on="Mode Buttons" class="RadioBtnsControl (strict)"("Val(Sgnl)"=T11."No Selection" ("Value (Signaling)")) -> ()  [unwired: 2 in, 2 out]
              }
              frame 0 {
              }
            }
            n643 = local write "LMB Down"(FALSE ("Mouse down")) -> ()
          }
        }
      }
      event "R-Plot 0", "R-Plot 1", "R-Plot 2", "R-Plot 3", "R-Plot 4", "R-Plot 5", "R-Plot 6", "R-Plot 7", "R-Plot 8", "R-Plot 9": Mouse Leave {
        n644 = event-data() -> ()  [unwired: 1 in, 4 out]
        n645 = local write "LMB Down"(FALSE ("Mouse down")) -> ()
      }
      event "R-Plot 0", "R-Plot 1", "R-Plot 2", "R-Plot 3", "R-Plot 4", "R-Plot 5", "R-Plot 6", "R-Plot 7", "R-Plot 8", "R-Plot 9": Scale Range Change {
        w912 = u8 0 ("X Scale.Scale Fit")
        # "Disable plot autoscaling if the user has changed the scale of the plot manualy"
        n646 = event-data() -> ("CtlRef"=w911:refnum<vi>)  [unwired: 1 in, 7 out]
        n647 = property class="XYGraph (strict)"(reference=w911, "XScale.ScaleFit"=w912, "YScale.ScaleFit"=w912) -> ()  [unwired: 1 in, 2 out]
      }
      event "R-Plot 0", "R-Plot 1", "R-Plot 2", "R-Plot 3", "R-Plot 4", "R-Plot 5", "R-Plot 6", "R-Plot 7", "R-Plot 8", "R-Plot 9": Shortcut Menu Activation? {
        w914 = string[] ["Zoom In to Last Data", "Autoscale XY"] ("item names")
        # "Add extra options to the plots context menu"
        n648 = event-data() -> ("MenuRef"=w916:refnum<k9>)  [unwired: 1 in, 6 out]
        n649 = Insert Menu Items(4:10, 7:w914, 8:w914, 9:w916) -> ()  [unwired: 2 in, 3 out]
        n650 = local read "LMB Down"() -> (w913:bool)
        n651 = event-data("Discard?"=w913) -> ()  [unwired: 1 in, 1 out]
      }
      event "R-Plot 0", "R-Plot 1", "R-Plot 2", "R-Plot 3", "R-Plot 4", "R-Plot 5", "R-Plot 6", "R-Plot 7", "R-Plot 8", "R-Plot 9": Shortcut Menu Selection (User) {
        # "Zoom in to last \"Miniplot points\". Zoom out a bit to have some space around the points"
        n652 = event-data() -> ("CtlRef"=w919:refnum<vi>, "ItemTag"=w917:string)  [unwired: 1 in, 6 out]
        n653 = Type Cast(type=refnum<vi> refnum ("R-Plot 0"), x=w919) -> (*(type *) &x=w918:refnum<vi>)
        n654 = case shown="\"Zoom In to Last Data\"" w917 {
          tunnel: w918 -> [_ w922 w951]
          frame Default {
          }
          frame "Autoscale XY" {
            w921 = u8 2 ("X Scale.Scale Fit")
            n655 = property class="XYGraph (strict)"(reference=w922, "XScale.ScaleFit"=w921, "YScale.ScaleFit"=w921) -> ()  [unwired: 1 in, 2 out]
          }
          frame "Zoom In to Last Data" {
            w947 = u8 0 ("Y Scale.Scale Fit")
            n656 = property on="AVS Runtime Settings" class="Clust (strict)"() -> ("Value"=w946:T12)  [unwired: 2 in, 2 out]
            n657 = property class="XYGraph (strict)"(reference=w951) -> (reference out=w948:refnum<vi>, "Value"=w950:cluster{dbl[], dbl[]})  [unwired: 1 in, 1 out]
            n658 = Unbundle By Name(w946) -> ("Data Memory 2"=w945:dbl)
            n659 = Unbundle(w950) -> (w924:dbl[], w949:dbl[])
            n660 = Multiply(x=w945, y=60.0) -> (x*y=w941:dbl)
            n661 = Reverse 1D Array(array=w924) -> (reversed array=w929:dbl[])
            n662 = Reverse 1D Array(array=w949) -> (reversed array=w937:dbl[])
            n663 = Index Array(array=w929) -> (element=w943:dbl)  [unwired: 1 in]
            n664 = Multiply(x=0.5, y=w941) -> (x*y=w942:dbl)
            n665 = Add(x=w942, y=w943) -> (x+y=w940:dbl)
            n666 = Subtract(x=w943, y=w941) -> (x-y=w938:dbl)
            n667 = call "Improved Threshold Detector.71.vi"("Threshold"=w938, "Array"=w924) -> ("Positive transition indices"=w925:i32[])  [unwired: 8 in, 1 out]
            n668 = Index Array(array=w925) -> (element=w952:i32)  [unwired: 1 in]
            n669 = Array Size(array=w924) -> (size(s)=w927:i32)
            n670 = Index Array(array=w924, index=w952) -> (element=w923:dbl)
            n671 = Subtract(x=w927, y=w952) -> (x-y=w926:i32)
            n672 = Array Subset(array=w937, length=w926) -> (w936:dbl[])  [unwired: 1 in]
            n673 = Array Max & Min(array=w936) -> (max value=w933:dbl, min value=w932:dbl)  [unwired: 2 out]
            n674 = Subtract(x=w933, y=w932) -> (x-y=w935:dbl)
            n675 = Divide(x=w935, y=2.0) -> (x/y=w931:dbl)
            n676 = Add(x=w933, y=w931) -> (x+y=w928:dbl)
            n677 = Subtract(x=w932, y=w931) -> (x-y=w930:dbl)
            n678 = property class="XYGraph (strict)"(reference=w948, "XScale.ScaleFit"=w947, "YScale.ScaleFit"=w947, "XScale.Maximum"=w940, "XScale.Minimum"=w923, "YScale.Maximum"=w928, "YScale.Minimum"=w930) -> ()  [unwired: 1 in, 2 out]
          }
        }
      }
      event "uPlots.uPlot 0", "uPlots.uPlot 1", "uPlots.uPlot 2", "uPlots.uPlot 3", "uPlots.uPlot 4", "uPlots.uPlot 5", "uPlots.uPlot 6", "uPlots.uPlot 7", "uPlots.uPlot 8", "uPlots.uPlot 9": Mouse Down {
        # "Switch to big plot on double click on small plot"
        n679 = event-data() -> ("Mods.Double Click"=w954:bool, "CtlRef"=w953:refnum<vi>)  [unwired: 1 in]
        n680 = case shown="True" w954 {
          tunnel: w953 -> [_ w957]
          frame False {
          }
          frame True {
            n681 = property class="XYGraph (strict)"(reference=w957) -> ("Label.Text"=w958:string)  [unwired: 1 in, 2 out]
            n682 = Reverse String(1:w958) -> (0:w959:string)
            n683 = Decimal String To Number(string=w959, default (0L)=8 ("default (0 I32)")) -> (number=w956:i32)  [unwired: 1 in, 1 out]
            n684 = property on="Channel Controls" class="TabCtl (strict)"("Val(Sgnl)"=w956) -> ()  [unwired: 2 in, 2 out]
          }
        }
      }
      event "Clear plot": Value Change {
        # "Clear data array.\nReset PID."
        n685 = event-data() -> ()  [unwired: 1 in, 6 out]
        n686 = local read "Channel Controls"() -> (w962:T1)
        n687 = local read "Data"() -> (w963:cluster{"R":dbl[], "T":dbl[], "Time":dbl[]}[])
        n688 = Replace Array Subset(array=w963, new element=cluster{"R":dbl[], "T":dbl[], "Time":dbl[]} {"R"=[], "T"=[], "Time"=[]} ("new element/subarray"), index=w962) -> (w961:cluster{"R":dbl[], "T":dbl[], "Time":dbl[]}[])
        n689 = local write "Data"(w961) -> ()
        n690 = disable-structure shown="Disabled" {
          frame Disabled {
            n691 = Initialize Array(cluster{"R":dbl[], "T":dbl[], "Time":dbl[]} {"R"=[], "T"=[], "Time"=[]}, 10 ("dimension size")) -> ()  [unwired: 1 out]
          }
          frame Enabled {
          }
        }
      }
      event "Clear all plots": Value Change {
        n692 = event-data() -> ()  [unwired: 1 in, 6 out]
        n693 = Initialize Array(cluster{"R":dbl[], "T":dbl[], "Time":dbl[]} {"R"=[], "T"=[], "Time"=[]}, 10 ("dimension size")) -> (w967:cluster{"R":dbl[], "T":dbl[], "Time":dbl[]}[])
        n694 = local write "Data"(w967) -> ()
      }
      event "Bridge settings.AVS type": Value Change {
        # "Select bridge type (AVS/zBridge). Show/hide corresponding controls."
        n695 = event-data() -> ("NewVal"=w970:T30)  [unwired: 1 in, 5 out]
        n696 = flat-sequence {
          tunnel: w970 -> [w976]
          frame #0 {
            w972 = u8 0 ("Disabled")
            w975 = u8 0 ("Disabled")
            w974 = FALSE ("Visible")
            w973 = u8 2 ("Disabled")
            n697 = property on="AVS_SPort" class="VISAName"("Visible"=w974, "Disabled"=w973) -> ()  [unwired: 2 in, 2 out]
            n698 = property on="Parameters" class="Bool"("Visible"=w974, "Disabled"=w973) -> ()  [unwired: 2 in, 2 out]
            n699 = property on="Tab Control 5" class="TabCtl (strict)"("Disabled"=w972) -> ()  [unwired: 2 in, 2 out]
            n700 = property on="Address" class="VISAName"("Visible"=w974, "Disabled"=w973) -> ()  [unwired: 2 in, 2 out]
            n701 = property on="Tab Control" class="TabCtl (strict)"("Disabled"=w972) -> ()  [unwired: 2 in, 2 out]
            n702 = property on="Read AVS channels from" class="DigNum (strict)"("Disabled"=w975) -> ()  [unwired: 2 in, 2 out]
            n703 = property on="Last Channel" class="DigNum (strict)"("Disabled"=w975) -> ()  [unwired: 2 in, 2 out]
            n704 = property on="Stabilisation Delay" class="DigNum (strict)"("Disabled"=w975) -> ()  [unwired: 2 in, 2 out]
            n705 = property on="Averages" class="DigNum (strict)"("Disabled"=w975) -> ()  [unwired: 2 in, 2 out]
            n706 = property on="Delay Between Scans" class="DigNum (strict)"("Disabled"=w975) -> ()  [unwired: 2 in, 2 out]
          }
          frame #1 {
            n707 = case shown="\"AVS47B (RS232 interface)\"" w976 {
              frame "AVS47A (GPIB interface)", Default {
                n708 = local write "Scan Parameters"(enum32{"Page 1", "Page 2"}."Page 1" ("Scan Parameters")) -> ()
                n709 = property on="Address" class="VISAName"("Visible"=TRUE, "Disabled"=u8 0) -> ()  [unwired: 2 in, 2 out]
              }
              frame "AVS47B (RS232 interface)" {
                w980 = u8 2 ("Disabled")
                n710 = local write "Scan Parameters"(enum32{"Page 1", "Page 2"}."Page 1" ("Scan Parameters")) -> ()
                n711 = property on="AVS_SPort" class="VISAName"("Visible"=TRUE, "Disabled"=u8 0) -> ()  [unwired: 2 in, 2 out]
                n712 = property on="Read AVS channels from" class="DigNum (strict)"("Disabled"=w980) -> ()  [unwired: 2 in, 2 out]
                n713 = property on="Last Channel" class="DigNum (strict)"("Disabled"=w980) -> ()  [unwired: 2 in, 2 out]
              }
              frame "AVS Emulation" {
                n714 = local write "Scan Parameters"(enum32{"Page 1", "Page 2"}."Page 1" ("Scan Parameters")) -> ()
              }
              frame "Impedance Bridge" {
                w987 = u8 2 ("Disabled")
                n715 = local write "Scan Parameters"(enum32{"Page 1", "Page 2"}."Page 2" ("Scan Parameters")) -> ()
                n716 = property on="Parameters" class="Bool"("Visible"=TRUE, "Disabled"=u8 0) -> ()  [unwired: 2 in, 2 out]
                n717 = property on="Read AVS channels from" class="DigNum (strict)"("Disabled"=w987) -> ()  [unwired: 2 in, 2 out]
                n718 = property on="Last Channel" class="DigNum (strict)"("Disabled"=w987) -> ()  [unwired: 2 in, 2 out]
                n719 = property on="Stabilisation Delay" class="DigNum (strict)"("Disabled"=w987) -> ()  [unwired: 2 in, 2 out]
                n720 = property on="Averages" class="DigNum (strict)"("Disabled"=w987) -> ()  [unwired: 2 in, 2 out]
                n721 = property on="Delay Between Scans" class="DigNum (strict)"("Disabled"=w987) -> ()  [unwired: 2 in, 2 out]
              }
              frame "Disabled" {
                w989 = u8 2 ("Disabled")
                n722 = property on="Tab Control 5" class="TabCtl (strict)"("Disabled"=w989) -> ()  [unwired: 2 in, 2 out]
                n723 = property on="Tab Control" class="TabCtl (strict)"("Disabled"=w989) -> ()  [unwired: 2 in, 2 out]
              }
            }
          }
        }
      }
      event "AVS Runtime Settings.Plot type": Value Change {
        # "Iterate through first 10 pages (plots only)"
        # "Switch between RxTime and TxTime plots"
        n724 = event-data() -> ("NewVal"=w998:enum16{"R vs Time", "T vs Time"})  [unwired: 1 in, 5 out]
        n725 = Equal To 0?(x=w998) -> (x = 0?=w997:bool)
        n726 = Select(t=u32 10532351, s=w997, f=u32 16711680) -> (s? t:f=w994:u32)
        n727 = property on="uPlots" class="Clust (strict)"() -> ("Controls[]"=w992:refnum<vi>[])  [unwired: 2 in, 2 out]
        n728 = property on="Channel Controls" class="TabCtl (strict)"() -> ("Pages"=w999:refnum<vi>[])  [unwired: 2 in, 2 out]
        n729 = for {
          N: 10 -> [_]
          tunnel: w999 -> [w1009] mode=indexing
          tunnel: w994 -> [w1001]
          tunnel: w992 -> [w1002] mode=indexing
          # "!!NOTE:This routine assumes that graph is control #1 on page!!"
          n730 = property class="Page"(reference=w1009) -> ("ControlsOnPage"=w1007:refnum<vi>[])  [unwired: 1 in, 2 out]
          n731 = Type Cast(type=refnum<vi> refnum ("R-Plot 0"), x=w1002) -> (*(type *) &x=w1000:refnum<vi>)
          n732 = Index Array(array=w1007, index=1) -> (element=w1005:refnum<vi>)
          n733 = Type Cast(type=refnum<vi> refnum ("R-Plot 0"), x=w1005) -> (*(type *) &x=w1004:refnum<vi>)
          n734 = property class="XYGraph (strict)"(reference=w1000, "Plot.Plot Color"=w1001, "Plot.Fill/Pt. Color"=w1001) -> ()  [unwired: 1 in, 2 out]
          n735 = property class="XYGraph (strict)"(reference=w1004, "Plot.Plot Color"=w1001, "Plot.Fill/Pt. Color"=w1001) -> ()  [unwired: 1 in, 2 out]
        }
        n736 = property on="ResetPIDloop" class="TypRef (strict)"() -> ("Value"=w991:refnum<user-event>)  [unwired: 2 in, 2 out]
        n737 = Generate User Event(user event=w991, event data cluster="" ("event data")) -> ()  [unwired: 2 in, 2 out]
      }
      event "AVS Runtime Settings.Read AVS channels from", "AVS Runtime Settings.Last Channel": Value Change {
        # "Change enabled channels for the AVS bridge"
        n738 = event-data() -> ()  [unwired: 1 in, 6 out]
        n739 = local read "UpdateChannelInfo"() -> (w1011:refnum<user-event>)
        n740 = Generate User Event(user event=w1011, event data cluster=bool[] [] ("event data")) -> ()  [unwired: 2 in, 2 out]
      }
      event "AVS Runtime Settings.Filter graphs:": Value Change {
        # "Graph filtering controls"
        n741 = event-data() -> ("NewVal"=w1012:bool)  [unwired: 1 in, 5 out]
        n742 = call "IsDisabled.vi"("Enabled?"=w1012) -> ("Numeric"=w1013:i16)
        n743 = property on="Y_min" class="DigNum (strict)"("Disabled"=w1013) -> ()  [unwired: 2 in, 2 out]
        n744 = property on="Y_max" class="DigNum (strict)"("Disabled"=w1013) -> ()  [unwired: 2 in, 2 out]
      }
      event "Channel Controls": Value Change {
        # "Show hide bottom Tesistance/Temperature panel depending on the current tab page"
        n745 = event-data() -> ("NewVal"=w1014:T1)  [unwired: 1 in, 5 out]
        n746 = case shown="Default" w1014 {
          frame Default {
            n747 = property on="Mode Buttons" class="RadioBtnsControl (strict)"() -> ("Value"=w1015:T11)  [unwired: 2 in, 2 out]
            n748 = property on="Data History" class="TabCtl (strict)"("Value"=enum32{"History", "Settings"}."History" ("Data History")) -> ()  [unwired: 2 in, 2 out]
            n749 = property on="Mode Buttons" class="RadioBtnsControl (strict)"("Val(Sgnl)"=w1015) -> ()  [unwired: 2 in, 2 out]
          }
          frame "All" {
            n750 = property on="Data History" class="TabCtl (strict)"("Value"=enum32{"History", "Settings"}."Settings" ("Data History")) -> ()  [unwired: 2 in, 2 out]
          }
        }
      }
      event "Thermometer": Value Change {
        # "Calibration changed - update calibrations list"
        n751 = event-data() -> ()  [unwired: 1 in, 6 out]
        n752 = property on="Thermometer" class="Clust (strict)"() -> ("Controls[]"=w1020:refnum<vi>[])  [unwired: 2 in, 2 out]
        n753 = Array Size(array=w1020) -> (size(s)=w1021:i32)
        n754 = for {
          N: w1021 -> [_]
          tunnel: w1020 -> [w1025] mode=indexing
          tunnel: [w1022] -> w1019 mode=indexing
          w1024 = refnum<vi> refnum  # Ring
          n755 = Type Cast(type=w1024, x=w1025) -> (*(type *) &x=w1023:refnum<vi>)
          n756 = property class="Ring"(reference=w1023) -> ("RingText.Text"=w1022:string)  [unwired: 1 in, 2 out]
        }
        n757 = Array To Cluster(array=w1019) -> (cluster=→"CurCalibrations":T18)
      }
      event User Event; "Data logging": Value Change {
        # "Log file settings changed. Generate new log file name"
        n758 = event-data() -> ()  [unwired: 1 in, 3 out]
        n759 = local read "Data logging"() -> (w1033:T22)
        n760 = Unbundle By Name(w1033) -> ("Run description"=w1027:string, "Filenames suffix"=w1028:string, "AVS_Path"=w1034:path, "AVS_FName"=w1032:string, "CAL_FName"=w1031:string)
        n761 = local write "LogFileCreationTime"(timestamp(2742897600 s since 1904-01-01)) -> ()
        n762 = call "MGI Make String Filesafe.vi"("String In"=w1027) -> ("Filesafe String Out"=w1026:string)
        n763 = call "GeneratePaths.vi"("Filename Suffix"=w1028, "Run description"=w1026, "AVS_Path"=w1034, "AVS_FName"=w1032, "CAL_Path"=w1034, "CAL_FName"=w1031) -> ("Generated Log path"=w1030:path, "Generated Calib path"=w1029:path)  [unwired: 8 in]
        n764 = local write "Log path"(w1030) -> ()
        n765 = local write "Calib path"(w1029) -> ()
      }
      event "Convert": Mouse Down {
        # "Quick convert R->T"
        n766 = event-data() -> ()  [unwired: 1 in, 8 out]
        n767 = property on="Select sensor 1" class="Ring (strict)"() -> ("Strings []"=w1038:string[], "Value"=w1039:u16)  [unwired: 2 in, 2 out]
        n768 = property on="AVS_CalFolder" class="Path"() -> ("Value"=w1036:path)  [unwired: 2 in, 2 out]
        n769 = Index Array(array=w1038, index=w1039) -> (element=w1037:string)
        n770 = call "SelectSensor-txt no ext.vi"("Path"=w1036, "Resistance"="R7", "Select sensor"=w1037) -> ("Temperature"=→"T7":dbl)  [unwired: 1 out]
      }
      event "T Sweep.Current": Value Change {
        # "Current/ Setpoint value is changed"
        n771 = event-data() -> ("NewVal"=→"I3_SetPnt":dbl)  [unwired: 1 in, 5 out]
        n772 = property on="ResetPIDloop" class="TypRef (strict)"() -> ("Value"=w1043:refnum<user-event>)  [unwired: 2 in, 2 out]
        n773 = Generate User Event(user event=w1043, event data cluster="" ("event data")) -> ()  [unwired: 2 in, 2 out]
      }
      event "Automode 2": Value Change {
        n774 = event-data() -> ("NewVal"=w1045:bool)  [unwired: 1 in, 5 out]
        n775 = case shown="True" w1045 {
          frame False {
          }
          frame True {
            # "Set timer to zero (01-01-1904) so the first point is set immediately, w/o wainting for time delay."
            # "If automatic mode is enabled- fire TempStabilized event to record current R,T,I values and start sweeping through TCS channels arrays"
            n776 = disable-structure shown="Disabled" {
              frame Disabled {
                n777 = Generate User Event(event data cluster="" ("event data")) -> ()  [unwired: 3 in, 2 out]
                "Time Old" <- 0.0 ("Timer")
              }
              frame Enabled {
              }
            }
          }
        }
      }
      event "Mode": Value Change {
        # "Changed Channel1 automatic mode"
        n778 = event-data() -> ()  [unwired: 1 in, 6 out]
        n779 = property on="Mode" class="Enum (strict)"() -> ("Value"=w1049:enum16{"Manual", "Automatic"})  [unwired: 2 in, 2 out]
        n780 = case shown="\"Automatic\"" w1049 {
          tunnel: [TRUE ("Automatic mode ON") FALSE ("Automatic mode ON")] -> w1048
          frame "Automatic" {
            w1051 = TRUE
            # "Set automatic mode currents equal to last manual values. Switch on the current sources."
            n781 = property on="ON" class="Bool (strict)"() -> ("Value"=w1055:bool)  [unwired: 2 in, 2 out]
            n782 = property on="ON" class="Bool (strict)"() -> ("Value"=w1054:bool)  [unwired: 2 in, 2 out]
            n783 = property on="ON" class="Bool (strict)"() -> ("Value"=w1053:bool)  [unwired: 2 in, 2 out]
            n784 = property on="ON" class="Bool (strict)"() -> ("Value"=w1052:bool)  [unwired: 2 in, 2 out]
            n785 = local read "I"() -> (w1060:dbl[])
            n786 = Exclusive Or(1:w1055, 2:w1051) -> (0:w1059:bool)
            n787 = Exclusive Or(1:w1054, 2:w1051) -> (0:w1057:bool)
            n788 = Exclusive Or(1:w1053, 2:w1051) -> (0:w1056:bool)
            n789 = Exclusive Or(1:w1052, 2:w1051) -> (0:w1058:bool)
            n790 = local write "I 2"(w1060) -> ()
            n791 = property on="Toggle ON/OFF" class="Bool (strict)"("Value"=w1059) -> ()  [unwired: 2 in, 2 out]
            n792 = property on="Toggle ON/OFF" class="Bool (strict)"("Value"=w1057) -> ()  [unwired: 2 in, 2 out]
            n793 = property on="Toggle ON/OFF" class="Bool (strict)"("Value"=w1056) -> ()  [unwired: 2 in, 2 out]
            n794 = property on="Toggle ON/OFF" class="Bool (strict)"("Value"=w1058) -> ()  [unwired: 2 in, 2 out]
          }
          frame "Manual" {
            # "Set manual mode currents \nequal to last automode \nvalues."
            n795 = local read "I 2"() -> (w1062:dbl[])
            n796 = Index Array(array=w1062) -> (element #1=w1066:dbl, element #2=w1065:dbl, element #3=w1064:dbl, element #4=w1063:dbl)  [unwired: 4 in]
            n797 = property on="I0" class="DigNum (strict)"("Val(Sgnl)"=w1066) -> ()  [unwired: 2 in, 2 out]
            n798 = property on="I1" class="DigNum (strict)"("Val(Sgnl)"=w1065) -> ()  [unwired: 2 in, 2 out]
            n799 = property on="I2" class="DigNum (strict)"("Val(Sgnl)"=w1064) -> ()  [unwired: 2 in, 2 out]
            n800 = property on="I3" class="DigNum (strict)"("Val(Sgnl)"=w1063) -> ()  [unwired: 2 in, 2 out]
          }
        }
        "Automatic mode 1" <- w1048
        "Automatic mode 2" <- w1048
        "Automatic mode 3" <- w1048
        "Automatic mode 0" <- w1048
      }
      event "Next step": Value Change {
        # "Go to next step in CS auto mode."
        n801 = event-data() -> ()  [unwired: 1 in, 6 out]
        n802 = flat-sequence {
          frame #0 {
            n803 = Get Date/Time In Seconds() -> (seconds since 1Jan1904=w1068:timestamp)
            n804 = To Double Precision Float(number=w1068) -> (double precision float=w1069:dbl)
            n805 = local write "Time Old"(w1069) -> ()
          }
          frame #1 {
            n806 = property on="TempStabilized" class="TypRef (strict)"() -> ("Value"=w1071:refnum<user-event>)  [unwired: 2 in, 2 out]
            n807 = Generate User Event(user event=w1071, event data cluster=TRUE ("event data")) -> ()  [unwired: 2 in, 2 out]
          }
        }
      }
      event "Data logging.External VI path": Value Change {
        # "Set path for the external VI to call on TempStabilised event"
        n808 = event-data() -> ("NewVal"=w1073:path)  [unwired: 1 in, 5 out]
        n809 = vi-ref "OnTempStabilizedRef.vi"() -> (w1074:refnum<vi>)
        n810 = Open VI Reference(type specifier VI Refnum (for type only)=w1074, vi path=w1073) -> (vi reference=w1072:refnum<vi>)  [unwired: 4 in, 1 out]
        n811 = local write "vi reference"(w1072) -> ()
      }
      event "Autorange": Value Change {
        # "Disabled"
        n812 = event-data() -> ("NewVal"=w1075:bool)  [unwired: 1 in, 5 out]
        n813 = Boolean To (0,1)(Boolean=w1075) -> (0, 1=w1078:i16)
        n814 = Multiply(x=i16 2, y=w1078) -> (x*y=w1076:i16)
        n815 = property on="Ranges" class="Clust (strict)"("Disabled"=w1076) -> ()  [unwired: 2 in, 2 out]
      }
      event "Current source settings.CS type": Value Change {
        # "Set CS type"
        n816 = event-data() -> ("NewVal"=w1079:T31)  [unwired: 1 in, 5 out]
        n817 = flat-sequence {
          tunnel: w1079 -> [w1106]
          frame #0 {
            w1091 = u8 2 ("Disabled")
            w1086 = u8 0 ("Disabled")
            w1101 = TRUE ("Visible")
            n818 = control-ref of="Tab Control 3"() -> (w1087:refnum<vi>)
            n819 = control-ref of="Ch0 -"() -> (w1098:refnum<vi>)
            n820 = control-ref of="Chn 1"() -> (w1090:refnum<vi>)
            n821 = control-ref of="I0"() -> (w1097:refnum<vi>)
            n822 = control-ref of="I1"() -> (w1089:refnum<vi>)
            n823 = control-ref of="Chn 2"() -> (w1085:refnum<vi>)
            n824 = control-ref of="Chn 3"() -> (w1084:refnum<vi>)
            n825 = control-ref of="Mode"() -> (w1088:refnum<vi>)
            n826 = control-ref of="Map Channel 0 to 2"() -> (w1096:refnum<vi>)
            n827 = property class="TabCtl (strict)"(reference=w1087, "Disabled"=w1086) -> ()  [unwired: 1 in, 2 out]
            n828 = property class="Clust (strict)"(reference=w1098, "Disabled"=w1086) -> ()  [unwired: 1 in, 2 out]
            n829 = property class="Clust (strict)"(reference=w1090, "Disabled"=w1086) -> ()  [unwired: 1 in, 2 out]
            n830 = property class="Clust (strict)"(reference=w1085, "Disabled"=w1086) -> ()  [unwired: 1 in, 2 out]
            n831 = property class="Clust (strict)"(reference=w1084, "Disabled"=w1086) -> ()  [unwired: 1 in, 2 out]
            n832 = property class="Clust (strict)"(reference=w1097, "Disabled"=w1086) -> ()  [unwired: 1 in, 2 out]
            n833 = property class="Clust (strict)"(reference=w1089, "Disabled"=w1086) -> ()  [unwired: 1 in, 2 out]
            n834 = property class="Enum (strict)"(reference=w1096, "Disabled"=w1086) -> ()  [unwired: 1 in, 2 out]
            n835 = property class="Enum (strict)"(reference=w1088, "Disabled"=w1086) -> ()  [unwired: 1 in, 2 out]
            n836 = control-ref of="TCS_Port"() -> (w1100:refnum<vi>)
            n837 = property on="Tab Control 2" class="TabCtl (strict)"() -> ("Pages"=w1080:refnum<vi>[])  [unwired: 2 in, 2 out]
            n838 = Index Array(array=w1080, index=1) -> (element=w1081:refnum<vi>)
            n839 = control-ref of="Toggle Gated"() -> (w1092:refnum<vi>)
            n840 = control-ref of="Toggle Gated"() -> (w1093:refnum<vi>)
            n841 = control-ref of="Toggle Gated"() -> (w1094:refnum<vi>)
            n842 = control-ref of="Toggle Gated"() -> (w1095:refnum<vi>)
            n843 = control-ref of="QCS/PCS Device"() -> (w1103:refnum<vi>)
            n844 = control-ref of="Set QCS Channel 0 output to"() -> (w1102:refnum<vi>)
            n845 = property class="Page"(reference=w1081, "PageVis"=TRUE ("Page Visible")) -> ()  [unwired: 1 in, 2 out]
            n846 = property class="Bool (strict)"(reference=w1092, "Disabled"=w1091) -> ()  [unwired: 1 in, 2 out]
            n847 = property class="Bool (strict)"(reference=w1093, "Disabled"=w1091) -> ()  [unwired: 1 in, 2 out]
            n848 = property class="Bool (strict)"(reference=w1094, "Disabled"=w1091) -> ()  [unwired: 1 in, 2 out]
            n849 = property class="Bool (strict)"(reference=w1095, "Disabled"=w1091) -> ()  [unwired: 1 in, 2 out]
            n850 = property class="DigNum (strict)"(reference=w1103, "Visible"=w1101) -> ()  [unwired: 1 in, 2 out]
            n851 = property class="Enum (strict)"(reference=w1102, "Visible"=w1101) -> ()  [unwired: 1 in, 2 out]
            n852 = property class="VISAName"(reference=w1100, "Visible"=FALSE) -> ()  [unwired: 1 in, 2 out]
          }
          frame #1 {
            n853 = case shown="\"Disabled\", Default" w1106 {
              tunnel: [refnum<class "TCS.lvclass"> refnum ("TCS.lvclass") refnum<class "QCS.lvclass"> refnum ("QCS.lvclass") w1126 w1140 refnum<class "PCS.lvclass"> refnum ("PCS.lvclass")] -> w1105
              tunnel: [w1107 w1125 u16 255 ("Value") u16 255 ("Value") w1145] -> w1104
              frame "TCS" {
                w1110 = u8 2 ("Disabled")
                w1123 = u8 0 ("Disabled")
                n854 = control-ref of="TCS_Port"() -> (w1113:refnum<vi>)
                n855 = control-ref of="Toggle Gated"() -> (w1122:refnum<vi>)
                n856 = control-ref of="Toggle Gated"() -> (w1121:refnum<vi>)
                n857 = control-ref of="Toggle Gated"() -> (w1120:refnum<vi>)
                n858 = control-ref of="Toggle Gated"() -> (w1119:refnum<vi>)
                n859 = control-ref of="QCS/PCS Device"() -> (w1115:refnum<vi>)
                n860 = control-ref of="Ch0 -"() -> (w1118:refnum<vi>)
                n861 = control-ref of="I0"() -> (w1111:refnum<vi>)
                n862 = control-ref of="Map Channel 0 to 2"() -> (w1112:refnum<vi>)
                n863 = property class="Bool (strict)"(reference=w1122, "Disabled"=w1123) -> ()  [unwired: 1 in, 2 out]
                n864 = property class="Bool (strict)"(reference=w1121, "Disabled"=w1123) -> ()  [unwired: 1 in, 2 out]
                n865 = property class="Bool (strict)"(reference=w1120, "Disabled"=w1123) -> ()  [unwired: 1 in, 2 out]
                n866 = property class="Bool (strict)"(reference=w1119, "Disabled"=w1123) -> ()  [unwired: 1 in, 2 out]
                n867 = property class="Clust (strict)"(reference=w1111, "Disabled"=w1110) -> ()  [unwired: 1 in, 2 out]
                n868 = property class="Clust (strict)"(reference=w1118, "Disabled"=u8 2) -> ()  [unwired: 1 in, 2 out]
                n869 = property class="DigNum (strict)"(reference=w1115, "Visible"=FALSE) -> ()  [unwired: 1 in, 2 out]
                n870 = property class="VISAName"(reference=w1113, "Visible"=TRUE) -> ()  [unwired: 1 in, 2 out]
                n871 = property class="Enum (strict)"(reference=w1112, "Disabled"=w1110) -> ()  [unwired: 1 in, 2 out]
                n872 = property on="TCS_Port" class="VISAName"() -> ("Value"=w1108:refnum<visa-resource-name>)  [unwired: 2 in, 2 out]
                n873 = call "VISA to RS232 Port Nr.vi"("VISA Resource Name"=w1108) -> ("Port Number"=w1107:u8)  [unwired: 1 in]
              }
              frame "QCS v1" {
                n874 = property on="QCS/PCS Device" class="DigNum (strict)"() -> ("Value"=w1125:u16)  [unwired: 2 in, 2 out]
              }
              frame "CS Emulation" {
                w1126 = refnum<class "CS Emulation.lvclass"> refnum  # CS Emulation.lvclass
                n875 = control-ref of="QCS/PCS Device"() -> (w1129:refnum<vi>)
                n876 = property class="DigNum (strict)"(reference=w1129, "Visible"=FALSE) -> ()  [unwired: 1 in, 2 out]
              }
              frame "Disabled", Default {
                w1130 = u8 2 ("Disabled")
                w1140 = refnum<class "CS Emulation.lvclass"> refnum  # CS Emulation.lvclass
                n877 = control-ref of="Tab Control 3"() -> (w1139:refnum<vi>)
                n878 = control-ref of="Ch0 -"() -> (w1134:refnum<vi>)
                n879 = control-ref of="Chn 1"() -> (w1133:refnum<vi>)
                n880 = control-ref of="Chn 2"() -> (w1132:refnum<vi>)
                n881 = control-ref of="Chn 3"() -> (w1131:refnum<vi>)
                n882 = control-ref of="QCS/PCS Device"() -> (w1143:refnum<vi>)
                n883 = property class="DigNum (strict)"(reference=w1143, "Visible"=FALSE) -> ()  [unwired: 1 in, 2 out]
                n884 = property class="Clust (strict)"(reference=w1134, "Disabled"=w1130) -> ()  [unwired: 1 in, 2 out]
                n885 = property class="Clust (strict)"(reference=w1133, "Disabled"=w1130) -> ()  [unwired: 1 in, 2 out]
                n886 = property class="Clust (strict)"(reference=w1132, "Disabled"=w1130) -> ()  [unwired: 1 in, 2 out]
                n887 = property class="Clust (strict)"(reference=w1131, "Disabled"=w1130) -> ()  [unwired: 1 in, 2 out]
                n888 = property class="TabCtl (strict)"(reference=w1139, "Disabled"=w1130) -> ()  [unwired: 1 in, 2 out]
                n889 = property on="Tab Control 2" class="TabCtl (strict)"() -> ("Pages"=w1138:refnum<vi>[])  [unwired: 2 in, 2 out]
                n890 = Index Array(array=w1138, index=1) -> (element=w1137:refnum<vi>)
                n891 = property class="Page"(reference=w1137, "PageVis"=FALSE ("Page Visible")) -> ()  [unwired: 1 in, 2 out]
              }
              frame "PCS (n.a.)" {
                w1146 = u8 2 ("Disabled")
                n892 = control-ref of="Ch0 -"() -> (w1152:refnum<vi>)
                n893 = control-ref of="Chn 1"() -> (w1151:refnum<vi>)
                n894 = control-ref of="I0"() -> (w1150:refnum<vi>)
                n895 = control-ref of="I1"() -> (w1149:refnum<vi>)
                n896 = control-ref of="Mode"() -> (w1148:refnum<vi>)
                n897 = control-ref of="Map Channel 0 to 2"() -> (w1147:refnum<vi>)
                n898 = property class="Clust (strict)"(reference=w1150, "Disabled"=w1146) -> ()  [unwired: 1 in, 2 out]
                n899 = property class="Clust (strict)"(reference=w1149, "Disabled"=w1146) -> ()  [unwired: 1 in, 2 out]
                n900 = property class="Clust (strict)"(reference=w1152, "Disabled"=w1146) -> ()  [unwired: 1 in, 2 out]
                n901 = property class="Clust (strict)"(reference=w1151, "Disabled"=w1146) -> ()  [unwired: 1 in, 2 out]
                n902 = property class="Enum (strict)"(reference=w1148, "Disabled"=w1146) -> ()  [unwired: 1 in, 2 out]
                n903 = property class="Enum (strict)"(reference=w1147, "Disabled"=w1146) -> ()  [unwired: 1 in, 2 out]
                n904 = property on="QCS/PCS Device" class="DigNum (strict)"() -> ("Value"=w1145:u16)  [unwired: 2 in, 2 out]
              }
            }
            "CS ref" <- w1105
            n905 = property on="HW Address" class="DigNum (strict)"("Value"=w1104) -> ()  [unwired: 2 in, 2 out]
          }
        }
      }
      event "Current source settings.QCS/PCS Device": Value Change {
        # "Set CS port"
        n906 = event-data() -> ("NewVal"=w1153:u16)  [unwired: 1 in, 5 out]
        n907 = property on="CS type" class="Enum (strict)"() -> ("Value"=w1154:T31)  [unwired: 2 in, 2 out]
        n908 = case shown="\"QCS v1\"" w1154 {
          tunnel: w1153 -> [_ w1157 _]
          frame Default {
          }
          frame "QCS v1" {
            n909 = Variant To Data(type=u32 255 ("HW Address"), Variant=w1157) -> (data=w1155:u32)  [unwired: 1 in, 1 out]
            n910 = property on="HW Address" class="DigNum (strict)"("Value"=w1155) -> ()  [unwired: 2 in, 2 out]
          }
          frame "CS Emulation" {
            n911 = property on="HW Address" class="DigNum (strict)"("Value"=u32 255 ("HW Address")) -> ()  [unwired: 2 in, 2 out]
          }
        }
      }
      event "Current source settings.TCS_Port": Value Change {
        # "Set TCS port"
        n912 = event-data() -> ("NewVal"=w1159:refnum<visa-resource-name>)  [unwired: 1 in, 5 out]
        n913 = property on="CS type" class="Enum (strict)"() -> ("Value"=w1160:T31)  [unwired: 2 in, 2 out]
        n914 = case shown="\"TCS\"" w1160 {
          tunnel: w1159 -> [w1163 _]
          frame "TCS" {
            n915 = Type Cast(type=refnum<visa-resource-name> refnum ("Value"), x=w1163) -> (*(type *) &x=w1162:refnum<visa-resource-name>)
            n916 = call "VISA to RS232 Port Nr.vi"("VISA Resource Name"=w1162) -> ("Port Number"=w1164:u8)  [unwired: 1 in]
            n917 = property on="HW Address" class="DigNum (strict)"("Value"=w1164) -> ()  [unwired: 2 in, 2 out]
          }
          frame Default {
          }
        }
      }
      event "I3 as temp.I3 as temp 2": Value Change {
        # "Enable/disable the PID loop"
        n918 = event-data() -> ("NewVal"=w1168:bool)  [unwired: 1 in, 5 out]
        n919 = call "IsDisabled.vi"("Enabled?"=w1168) -> ("Numeric"=w1172:i16)
        n920 = property on="ResetPIDloop" class="TypRef (strict)"() -> ("Value"=w1171:refnum<user-event>)  [unwired: 2 in, 2 out]
        n921 = property on="PID setup 2" class="Clust (strict)"("Disabled"=w1172) -> ()  [unwired: 2 in, 2 out]
        n922 = Generate User Event(user event=w1171, event data cluster="" ("event data")) -> ()  [unwired: 2 in, 2 out]
        n923 = property on="FB on" class="Enum (strict)"() -> ("Value"=w1165:enum16{"Resistance", "Temperature"})  [unwired: 2 in, 2 out]
        n924 = Index Array(array=string[] ["%#_g uA", "%#_g mK"], index=w1165) -> (element=w1167:string)
        n925 = Select(t=w1167, s=w1168, f="%#_g uA") -> ()  [unwired: 1 out]
      }
      event "Load Data": Value Change {
        # "Load data from log files"
        n926 = event-data() -> ()  [unwired: 1 in, 6 out]
        n927 = property on="AVS_Path" class="Path"() -> ("Value"=w1175:path)  [unwired: 2 in, 2 out]
        n928 = call "File Dialog4"("start path"=w1175) -> ("selected paths"=w1174:path[], "cancelled"=w1173:bool)  [unwired: 11 in, 2 out]
        n929 = case shown="False" w1173 {
          tunnel: w1174 -> [w1189 _]
          frame False {
            n930 = property on="AVS type" class="Enum (strict)"() -> ("Value"=w1179:T30)  [unwired: 2 in, 2 out]
            n931 = for {
              tunnel: w1189 -> [w1216] mode=indexing
              shift-right: [w1214] -> w1186
              shift-left: string[][] [] ("all rows") -> [w1215]
              # "skip header"
              n932 = call <vilib>:"Read From Spreadsheet File (string).vi"("file path (dialog if empty)"=w1216) -> ("all rows"=w1212:string[][])  [unwired: 6 in, 4 out]
              n933 = Array Subset(array=w1212, index (row)=6 ("index")) -> (w1211:string[][])  [unwired: 3 in]
              n934 = Insert Into Array(array=w1215, new element=w1211) -> (w1214:string[][])  [unwired: 2 in]
            }
            n935 = case shown="Default" w1179 {
              tunnel: [2 ("index") 2 ("index")] -> w1178
              tunnel: [8 ("length") 10 ("length")] -> w1176
              tunnel: [10 ("index") 12 ("index")] -> w1177
              frame Default {
              }
              frame "Impedance Bridge" {
              }
            }
            n936 = Index Array(array=w1186, index (col)=1 ("disabled index (col)")) -> (element=w1183:string[])  [unwired: 1 in]
            n937 = Array Subset(array=w1186, index (col)=w1178, length (col)=w1176) -> (w1185:string[][])  [unwired: 2 in]
            n938 = Array Subset(array=w1186, index (col)=w1177, length (col)=w1176) -> (w1184:string[][])  [unwired: 2 in]
            n939 = Transpose 2D Array(2D array=w1185) -> (transposed array=w1181:string[][])
            n940 = Transpose 2D Array(2D array=w1184) -> (transposed array=w1180:string[][])
            n941 = for {
              tunnel: w1181 -> [w1208] mode=indexing
              tunnel: w1180 -> [w1207] mode=indexing
              tunnel: w1183 -> [w1209]
              tunnel: [w1206] -> w1182 mode=indexing
              # "Sort data by date and remove duplicate points"
              n942 = Fract/Exp String To Number(string=w1208) -> (number=w1203:dbl[])  [unwired: 3 in, 1 out]
              n943 = Fract/Exp String To Number(string=w1209) -> (number=w1205:dbl[])  [unwired: 3 in, 1 out]
              n944 = Fract/Exp String To Number(string=w1207) -> (number=w1204:dbl[])  [unwired: 3 in, 1 out]
              n945 = call "Sort 1D Array (DBL)__ogtk.vi"("Array in"=w1205) -> ("Sorted Pointers"=w1210:i32[], "Sorted Array out"=w1198:dbl[])  [unwired: 9 in]
              n946 = call "Reorder 1D Array2 (DBL)__ogtk.vi"("indices"=w1210, "array"=w1203) -> ("reordered array"=w1202:dbl[])  [unwired: 9 in]
              n947 = call "Reorder 1D Array2 (DBL)__ogtk.vi"("indices"=w1210, "array"=w1204) -> ("reordered array"=w1200:dbl[])  [unwired: 9 in]
              n948 = call "Remove Duplicates from 1D Array (DBL)__ogtk.vi"("Input Array"=w1202) -> ("Output Array"=w1201:dbl[], "indices of removed elements"=w1196:i32[])
              n949 = call "Delete Elements from 1D Array (DBL)__ogtk.vi"("indices"=w1196, "array"=w1200) -> ("array w/ subset deleted"=w1199:dbl[])  [unwired: 8 in, 1 out]
              n950 = call "Delete Elements from 1D Array (DBL)__ogtk.vi"("indices"=w1196, "array"=w1198) -> ("array w/ subset deleted"=w1197:dbl[])  [unwired: 8 in, 1 out]
              n951 = Bundle("Output Array"=w1201, "array w/ subset deleted"=w1199, "array w/ subset deleted"=w1197) -> (w1206:T43)  [unwired: 1 in]
            }
            n952 = local write "Data"(w1182) -> ()
          }
          frame True {
          }
        }
      }
      event "Save Data": Value Change {
        # "Load data from log files"
        n953 = event-data() -> ()  [unwired: 1 in, 6 out]
        n954 = property on="AVS_Path" class="Path"() -> ("Value"=w1219:path)  [unwired: 2 in, 2 out]
        n955 = call "File Dialog"("start path"=w1219) -> ("selected path"=w1217:path, "cancelled"=w1218:bool)  [unwired: 11 in, 2 out]
        n956 = case shown="False" w1218 {
          tunnel: w1217 -> [w1224 _]
          frame False {
            (unwired) 30 ("dimension size")
            n957 = local read "Data"() -> (w1225:cluster{"R":dbl[], "T":dbl[], "Time":dbl[]}[])
            n958 = for {
              tunnel: w1225 -> [w1239] mode=indexing
              tunnel: [w1230] -> w1223 mode=indexing
              shift-right: [w1226] -> w1221
              shift-left: string[][] [] -> [w1227]
              n959 = Unbundle By Name(w1239) -> ("Time"=w1236:dbl[], "R"=w1235:dbl[], "T"=w1231:dbl[])
              n960 = property on="Data logging" class="Clust (strict)"() -> ("Value"=w1238:T22)  [unwired: 2 in, 2 out]
              n961 = Unbundle By Name(w1238) -> ("Date/Time Format"=w1237:string)
              n962 = Array Size(array=w1231) -> (size(s)=w1230:i32)
              n963 = for {
                tunnel: w1237 -> [w1242]
                tunnel: [w1241] -> w1234 mode=indexing
                tunnel: w1236 -> [w1240] mode=indexing
                n964 = Format Date/Time String(time format string (%c)=w1242, seconds (now)=w1240) -> (date/time string=w1241:string)  [unwired: 1 in]
              }
              n965 = Number To Fractional String(number=w1235) -> (F-format string=w1233:string[])  [unwired: 3 in]
              n966 = Number To Fractional String(number=w1231) -> (F-format string=w1232:string[])  [unwired: 3 in]
              n967 = Build Array(w1234, w1233, w1232) -> (w1228:string[][])
              n968 = Transpose 2D Array(2D array=w1228) -> (transposed array=w1229:string[][])
              n969 = Build Array (concatenate)(w1227, w1229) -> (w1226:string[][])
            }
            n970 = Array Max & Min(array=w1223) -> ()  [unwired: 4 out]
            n971 = call "Write To Spreadsheet File (string) w Error.vi"("transpose? (no:F)"=FALSE, "2D data"=w1221, "file path (dialog if empty)"=w1224) -> ()  [unwired: 7 in, 2 out]
          }
          frame True {
          }
        }
      }
      event "Currents changed": Value Change {
        # "New values for currents were entered by user/automode-> write new data to CS"
        n972 = event-data() -> ()  [unwired: 1 in, 6 out]
        n973 = local read "CS ref"() -> (w1247:refnum<class "CS.lvclass">)
        n974 = property on="CS status" class="Clust (strict)"() -> ("Value"=w1244:errorcluster)  [unwired: 2 in, 2 out]
        n975 = call-dynamic "Read.vi"("CS in"=w1247, "error in (no error)"=w1244, "Optional"=TRUE ("Unused")) -> ("CS out"=w1246:refnum<class "CS.lvclass">, "error out"=w1243:errorcluster)  [unwired: 11 in, 4 out]
        n976 = local write "CS ref"(w1246) -> ()
        n977 = property on="CS status" class="Clust (strict)"("Value"=w1243) -> ()  [unwired: 2 in, 2 out]
      }
      event "Set QCS Channel 0 output to": Value Change {
        # "Switch QCS channel 0 to aux output"
        n978 = event-data() -> ("OldVal"=w1254:T24, "NewVal"=w1249:T24)  [unwired: 1 in, 4 out]
        n979 = To Long Integer(number=w1249) -> (32bit integer=→"Map Channel 0 to 2":i32)
        n980 = local read "CS ref"() -> (w1252:refnum<class "CS.lvclass">)
        n981 = property on="CS status" class="Clust (strict)"() -> ("Value"=w1253:errorcluster)  [unwired: 2 in, 2 out]
        n982 = call-dynamic "Switch Output Channel.vi"("error in (no error)"=w1253, "New Channel"=w1249, "Old Channel"=w1254, "CS in"=w1252) -> ("error out"=w1250:errorcluster, "CS out"=w1251:refnum<class "CS.lvclass">)  [unwired: 6 in]
        n983 = local write "CS ref"(w1251) -> ()
        n984 = property on="CS status" class="Clust (strict)"("Value"=w1250) -> ()  [unwired: 2 in, 2 out]
      }
      event "T Sweep.Start": Value Change {
        # "Setup and Start Current/Temperature sweep for CS channel 3"
        n985 = event-data() -> ("CtlRef"=w1255:refnum<vi>, "NewVal"=w1256:bool)  [unwired: 1 in, 4 out]
        n986 = case shown="False" w1256 {
          tunnel: w1255 -> [w1257 w1260]
          frame False {
            n987 = property class="Bool (strict)"(reference=w1257, "Caption.Text"="Start") -> ()  [unwired: 1 in, 2 out]
          }
          frame True {
            n988 = property on="Start value" class="DigNum (strict)"() -> ("Value"=w1261:dbl)  [unwired: 2 in, 2 out]
            n989 = property class="Bool (strict)"(reference=w1260, "Caption.Text"="Stop") -> ()  [unwired: 1 in, 2 out]
            n990 = property on="Current" class="DigNum (strict)"("Val(Sgnl)"=w1261) -> ()  [unwired: 2 in, 2 out]
          }
        }
      }
      event "T Sweep.I_next": Value Change {
        # "Go to next step in Current/Temperature sweep for CS channel 3"
        n991 = event-data() -> ()  [unwired: 1 in, 6 out]
        n992 = property on="I_next" class="Bool (strict)"("Value"=FALSE) -> ()  [unwired: 2 in, 2 out]
        n993 = Get Date/Time In Seconds() -> (seconds since 1Jan1904=w1269:timestamp)
        n994 = To Double Precision Float(number=w1269) -> (double precision float=w1270:dbl)
        n995 = local write "Time Old"(w1270) -> ()
        n996 = property on="Current" class="DigNum (strict)"() -> ("Value"=w1262:dbl)  [unwired: 2 in, 2 out]
        n997 = property on="Step" class="DigNum (strict)"() -> ("Value"=w1267:dbl)  [unwired: 2 in, 2 out]
        n998 = Add(x=w1262, y=w1267) -> (x+y=w1266:dbl)
        n999 = property on="End value" class="DigNum (strict)"() -> ("Value"=w1265:dbl)  [unwired: 2 in, 2 out]
        n1000 = property on="Start value" class="DigNum (strict)"() -> ("Value"=w1264:dbl)  [unwired: 2 in, 2 out]
        n1001 = In Range and Coerce(upper limit=w1265, x=w1266, lower limit=w1264) -> (coerced(x)=w1263:dbl)  [unwired: 1 out]
        n1002 = property on="Current" class="DigNum (strict)"("Val(Sgnl)"=w1263) -> ()  [unwired: 2 in, 2 out]
      }
      event "T Sweep.I_prev": Value Change {
        # "Go to previous step in Current/Temperature sweep for CS channel 3"
        n1003 = event-data() -> ()  [unwired: 1 in, 6 out]
        n1004 = Get Date/Time In Seconds() -> (seconds since 1Jan1904=w1278:timestamp)
        n1005 = property on="I_prev" class="Bool (strict)"("Value"=FALSE) -> ()  [unwired: 2 in, 2 out]
        n1006 = To Double Precision Float(number=w1278) -> (double precision float=w1279:dbl)
        n1007 = local write "Time Old"(w1279) -> ()
        n1008 = property on="Current" class="DigNum (strict)"() -> ("Value"=w1272:dbl)  [unwired: 2 in, 2 out]
        n1009 = property on="Step" class="DigNum (strict)"() -> ("Value"=w1277:dbl)  [unwired: 2 in, 2 out]
        n1010 = Subtract(x=w1272, y=w1277) -> (x-y=w1276:dbl)
        n1011 = property on="End value" class="DigNum (strict)"() -> ("Value"=w1275:dbl)  [unwired: 2 in, 2 out]
        n1012 = property on="Start value" class="DigNum (strict)"() -> ("Value"=w1274:dbl)  [unwired: 2 in, 2 out]
        n1013 = In Range and Coerce(upper limit=w1275, x=w1276, lower limit=w1274) -> (coerced(x)=w1273:dbl)  [unwired: 1 out]
        n1014 = property on="Current" class="DigNum (strict)"("Val(Sgnl)"=w1273) -> ()  [unwired: 2 in, 2 out]
      }
      event "Reset PID", "PID setup 2.Integral Gain": Value Change {
        # "Reset the PID loop"
        n1015 = event-data() -> ()  [unwired: 1 in, 6 out]
        n1016 = property on="ResetPIDloop" class="TypRef (strict)"() -> ("Value"=w1281:refnum<user-event>)  [unwired: 2 in, 2 out]
        n1017 = Generate User Event(user event=w1281, event data cluster="" ("event data")) -> ()  [unwired: 2 in, 2 out]
      }
      event User Event {
        # "Reset the PID loop"
        n1018 = event-data() -> ()  [unwired: 1 in, 5 out]
        n1019 = local write "Error"(0.0 ("T_error")) -> ()
      }
      event "Minimize": Value Change {
        (unwired) 29 ("Splitter Position")
        (unwired) 534 ("Numeric 2")
        # "Shrink/restore the program window"
        # "726"
        # "222"
        # "1243"
        # "816"
        n1020 = event-data() -> ("NewVal"=w1284:bool)  [unwired: 1 in, 5 out]
        n1021 = case shown="True" w1284 {
          frame True {
            n1022 = property on="CS type" class="Enum (strict)"() -> ("Value"=w1294:T31)  [unwired: 2 in, 2 out]
            n1023 = property on="AVS type" class="Enum (strict)"() -> ("Value"=w1289:T30)  [unwired: 2 in, 2 out]
            n1024 = Equal?(x=w1289, y=T30."Disabled" ("Value")) -> (x = y?=w1286:bool)
            n1025 = Equal?(x=w1294, y=T31."Disabled" ("Value")) -> (x = y?=w1293:bool)
            n1026 = property on="Data History" class="TabCtl (strict)"("Value"=enum32{"History", "Settings"}."History" ("Data History")) -> ()  [unwired: 2 in, 2 out]
            n1027 = Exclusive Or(1:w1286, 2:w1293) -> (0:w1285:bool)
            n1028 = property on="Mode Buttons" class="RadioBtnsControl (strict)"("Disabled"=u8 2, "Val(Sgnl)"=T11."No Selection" ("Value (Signaling)")) -> ()  [unwired: 2 in, 2 out]
            n1029 = property class="VI"() -> ("Front Panel.PanelBounds"=w1297:T44)  [unwired: 2 in, 2 out]
            n1030 = Select(t=i16 105 ("y"), s=w1285, f=i16 169 ("y")) -> (s? t:f=w1290:i16)
            n1031 = Unbundle By Name(w1297) -> ("Left"=w1303:i16, "Top"=w1300:i16)
            n1032 = property on="Splitter 3" class="Splitter"("Position"=29 ("Splitter Position")) -> (error out=w1287:errorcluster)  [unwired: 2 in, 1 out]
            n1033 = Add(x=i16 806 ("right"), y=w1303) -> (x+y=w1302:i16)
            n1034 = Add(x=w1300, y=w1290) -> (x+y=w1299:i16)
            n1035 = Bundle By Name(cluster=w1297, "Right"=w1302, "Bottom"=w1299) -> (w1304:T44)
            n1036 = case shown="True" w1286 {
              tunnel: w1287 -> [_ w1307]
              frame False {
              }
              frame True {
                n1037 = property on="Splitter 4" class="Splitter"(error in=w1307, "Position"=32 ("Splitter Position")) -> ()  [unwired: 1 in, 2 out]
              }
            }
            n1038 = property class="VI"("Front Panel.PanelBounds"=w1304) -> ()  [unwired: 2 in, 2 out]
          }
          frame False {
            n1039 = property class="VI"() -> ("Front Panel.PanelBounds"=w1311:T44)  [unwired: 2 in, 2 out]
            n1040 = property on="Channel Controls" class="TabCtl (strict)"() -> ("Value"=w1320:T1)  [unwired: 2 in, 2 out]
            n1041 = Unbundle By Name(w1311) -> ("Left"=w1318:i16, "Top"=w1315:i16)
            n1042 = property on="Channel Controls" class="TabCtl (strict)"("Val(Sgnl)"=w1320) -> ()  [unwired: 2 in, 2 out]
            n1043 = property on="Splitter 3" class="Splitter"("Position"=560 ("Splitter Position")) -> (error out=w1309:errorcluster)  [unwired: 2 in, 1 out]
            n1044 = Add(x=i16 1233 ("right"), y=w1318) -> (x+y=w1317:i16)
            n1045 = Add(x=w1315, y=i16 704) -> (x+y=w1313:i16)
            n1046 = Bundle By Name(cluster=w1311, "Right"=w1317, "Bottom"=w1313) -> (w1319:T44)
            n1047 = property on="Splitter 4" class="Splitter"(error in=w1309, "Position"=635 ("Splitter Position")) -> ()  [unwired: 1 in, 2 out]
            n1048 = property class="VI"("Front Panel.PanelBounds"=w1319) -> ()  [unwired: 2 in, 2 out]
            n1049 = property on="Mode Buttons" class="RadioBtnsControl (strict)"("Disabled"=u8 0) -> ()  [unwired: 2 in, 2 out]
          }
        }
        n1050 = property on="Splitter 2" class="Splitter"("Position"=805 ("Splitter Position")) -> ()  [unwired: 2 in, 2 out]
      }
      event "Copy to Clipboard": Value Change {
        # "Copy current values to the clipboard"
        n1051 = event-data() -> ()  [unwired: 1 in, 6 out]
        n1052 = property on="Data array" class="Arr (strict)"() -> ("Value"=w1325:dbl[])  [unwired: 2 in, 2 out]
        n1053 = property on="T_array" class="Arr (strict)"() -> ("Value"=w1324:dbl[])  [unwired: 2 in, 2 out]
        n1054 = Build Array(w1325, w1324) -> (w1323:dbl[][])
        n1055 = Transpose 2D Array(2D array=w1323) -> (transposed array=w1322:dbl[][])
        n1056 = Array To Spreadsheet String(delimiter (Tab)="\t", array=w1322, 3:"%.4g" ("format string")) -> (spreadsheet string=w1328:string)
        n1057 = invoke class="App" method="Clipboard.Write"("Param 0"=w1328) -> ()  [unwired: 3 in, 4 out]
      }
      event "Show PID graph?": Value Change {
        # "Display plots with the PID parameters vs time for debugging"
        n1058 = event-data() -> ("NewVal"=w1329:bool)  [unwired: 1 in, 5 out]
        n1059 = property on="Channel Controls" class="TabCtl (strict)"() -> ("Pages"=w1332:refnum<vi>[])  [unwired: 2 in, 2 out]
        n1060 = Reverse 1D Array(array=w1332) -> (reversed array=w1331:refnum<vi>[])
        n1061 = Index Array(array=w1331) -> (element=w1330:refnum<vi>)  [unwired: 1 in]
        n1062 = property class="Page"(reference=w1330, "PageVis"=w1329) -> ()  [unwired: 1 in, 2 out]
      }
      event "Ch0 -.uA", "Chn 1.uA", "Chn 2.uA", "Chn 3.uA": Mouse Up {
        # "Show curent edit filed on double clicking the current indicator. Set the field to the actual current value."
        n1063 = event-data() -> ("Mods.Double Click"=w1334:bool, "CtlRef"=w1333:refnum<vi>)  [unwired: 1 in, 5 out]
        n1064 = case shown="True" w1334 {
          tunnel: w1333 -> [_ w1345]
          frame False {
          }
          frame True {
            w1341 = TRUE ("Visible")
            n1065 = property class="Str"(reference=w1345) -> ("Owner"=w1344:refnum<vi>)  [unwired: 1 in, 2 out]
            n1066 = control-ref of="uA 0"() -> (w1351:refnum<vi>)
            n1067 = control-ref of="uA 1"() -> (w1354:refnum<vi>)
            n1068 = control-ref of="uA 2"() -> (w1353:refnum<vi>)
            n1069 = control-ref of="uA 3"() -> (w1352:refnum<vi>)
            n1070 = control-ref of="Ch0 -"() -> (w1342:refnum<vi>)
            n1071 = control-ref of="Chn 1"() -> (w1348:refnum<vi>)
            n1072 = control-ref of="Chn 2"() -> (w1347:refnum<vi>)
            n1073 = control-ref of="Chn 3"() -> (w1340:refnum<vi>)
            n1074 = property on="I" class="Arr (strict)"() -> ("Value"=w1339:dbl[])  [unwired: 2 in, 2 out]
            n1075 = Type Cast(type=w1340, x=w1344) -> (*(type *) &x=w1343:refnum<vi>)
            n1076 = Build Array(w1351, w1354, w1353, w1352) -> (w1350:refnum<vi>[])
            n1077 = Build Array(w1342, w1348, w1347, w1340) -> (w1346:refnum<vi>[])
            n1078 = Search 1D Array(1D array=w1346, element=w1343) -> (index of element=w1338:i32)  [unwired: 1 in]
            n1079 = Index Array(array=w1339, index=w1338) -> (element=w1337:dbl)
            n1080 = Index Array(array=w1350, index=w1338) -> (element=w1349:refnum<vi>)
            n1081 = Multiply(x=1000.0, y=w1337) -> (x*y=w1336:dbl)
            n1082 = property on="Property Node" class="DigNum (strict)"(reference=w1349, "Value"=w1336, "Visible"=w1341, "Key Focus"=w1341) -> ()  [unwired: 1 in, 2 out]
          }
        }
      }
      event "Ch0 -.current flows", "Chn 1.current flows", "Chn 2.current flows", "Chn 3.current flows": Mouse Up {
        # "Toggle the current channel by double clickin on the \"On\" led in the current indicator."
        n1083 = event-data() -> ("CtlRef"=w1355:refnum<vi>, "Mods.Double Click"=w1356:bool)  [unwired: 1 in, 5 out]
        n1084 = case shown="True" w1356 {
          tunnel: w1355 -> [_ w1365]
          frame False {
          }
          frame True {
            n1085 = control-ref of="current flows"() -> (w1370:refnum<vi>)
            n1086 = control-ref of="current flows"() -> (w1369:refnum<vi>)
            n1087 = control-ref of="current flows"() -> (w1368:refnum<vi>)
            n1088 = control-ref of="current flows"() -> (w1367:refnum<vi>)
            n1089 = control-ref of="Toggle ON/OFF"() -> (w1364:refnum<vi>)
            n1090 = control-ref of="Toggle ON/OFF"() -> (w1362:refnum<vi>)
            n1091 = control-ref of="Toggle ON/OFF"() -> (w1361:refnum<vi>)
            n1092 = control-ref of="Toggle ON/OFF"() -> (w1363:refnum<vi>)
            n1093 = Build Array(w1370, w1369, w1368, w1367) -> (w1366:refnum<vi>[])
            n1094 = Build Array(w1364, w1362, w1361, w1363) -> (w1360:refnum<vi>[])
            n1095 = Search 1D Array(1D array=w1366, element=w1365) -> (index of element=w1359:i32)  [unwired: 1 in]
            n1096 = Index Array(array=w1360, index=w1359) -> (element=w1358:refnum<vi>)
            n1097 = property class="Bool (strict)"(reference=w1358, "Val(Sgnl)"=TRUE ("Value (Signaling)")) -> ()  [unwired: 1 in, 2 out]
          }
        }
      }
      event "uA 0", "uA 1", "uA 2", "uA 3": Value Change {
        w1372 = refnum<vi> refnum  # Numeric
        w1376 = refnum<vi> refnum  # Enum
        # "User has entered the current by double clicking on the current indicators at the bottom. \nSet range to \"Auto\" and interpret the entered value as [uA]"
        # "!!NOTE:This routine assumes that Current and Range are controls #2 & #3 in current control cluster"
        n1098 = event-data() -> ("CtlRef"=w1384:refnum<vi>, "NewVal"=w1371:u32)  [unwired: 1 in, 4 out]
        n1099 = control-ref of="I0"() -> (w1393:refnum<vi>)
        n1100 = control-ref of="I1"() -> (w1391:refnum<vi>)
        n1101 = control-ref of="I2"() -> (w1392:refnum<vi>)
        n1102 = control-ref of="I3"() -> (w1394:refnum<vi>)
        n1103 = control-ref of="uA 0"() -> (w1386:refnum<vi>)
        n1104 = control-ref of="uA 1"() -> (w1389:refnum<vi>)
        n1105 = control-ref of="uA 2"() -> (w1388:refnum<vi>)
        n1106 = control-ref of="uA 3"() -> (w1387:refnum<vi>)
        n1107 = Build Array(w1393, w1391, w1392, w1394) -> (w1390:refnum<vi>[])
        n1108 = Build Array(w1386, w1389, w1388, w1387) -> (w1385:refnum<vi>[])
        n1109 = Search 1D Array(1D array=w1385, element=w1384) -> (index of element=w1383:i32)  [unwired: 1 in]
        n1110 = Index Array(array=w1390, index=w1383) -> (element=w1382:refnum<vi>)
        n1111 = property class="Clust (strict)"(reference=w1382) -> ("Controls[]"=w1381:refnum<vi>[])  [unwired: 1 in, 2 out]
        n1112 = Index Array(array=w1381, index #1=3 ("index"), index #2=2 ("index")) -> (element #1=w1378:refnum<vi>, element #2=w1374:refnum<vi>)
        n1113 = Type Cast(type=w1372, x=w1374) -> (*(type *) &x=w1373:refnum<vi>)
        n1114 = Type Cast(type=w1376, x=w1378) -> (*(type *) &x=w1377:refnum<vi>)
        n1115 = property on="Property Node" class="Num"(reference=w1373, "Value"=w1371) -> ()  [unwired: 1 in, 2 out]
        n1116 = property on="Property Node" class="Enum"(reference=w1377, "Value"=T32."Auto") -> ()  [unwired: 1 in, 2 out]
      }
      event "Ranges": Value Change {
        # "If user has changed the exitation, update the AVS bridge settings."
        n1117 = event-data() -> ("NewVal"=w1396:T13)  [unwired: 1 in, 5 out]
        n1118 = property on="Exc&Ranges" class="Clust (strict)"() -> ("Value"=w1395:T7)  [unwired: 2 in, 2 out]
        n1119 = call "Combine Excitation&Range.vi"("Ranges"=w1396, "Exc&Ranges In"=w1395) -> ("Exc&Ranges Out"=w1397:T45)
        n1120 = property on="Exc&Ranges" class="Clust (strict)"("Value"=w1397) -> ()  [unwired: 2 in, 2 out]
      }
      event Panel Close? {
        # "Ask for confirmation is user is trying to close the program"
        n1121 = event-data() -> ()  [unwired: 1 in, 4 out]
        n1122 = Two Button Dialog(message="Are you sure you want to quit the program?") -> (T button?=w1399:bool)  [unwired: 2 in]
        n1123 = Not(x=w1399) -> (.not. x?=w1400:bool)
        n1124 = event-data("Discard?"=w1400) -> ()  [unwired: 1 in, 1 out]
      }
      event "Save config": Mouse Up {
        (unwired) T34."HKEY_CURRENT_USER" ("root key (HKEY_LOCAL_MACHINE) 2")
        # "Save parameters to the configuration file"
        n1125 = event-data() -> ()  [unwired: 1 in, 8 out]
        n1126 = control-ref of="CS Names"() -> (w1411:refnum<vi>)
        n1127 = control-ref of="AVS names"() -> (w1410:refnum<vi>)
        n1128 = control-ref of="CurCalibrations"() -> (w1404:refnum<vi>)
        n1129 = control-ref of="I3 as temp"() -> (w1402:refnum<vi>)
        n1130 = control-ref of="Automode Settings 2"() -> (w1401:refnum<vi>)
        n1131 = control-ref of="Active"() -> (w1403:refnum<vi>)
        n1132 = control-ref of="Bridge settings"() -> (w1417:refnum<vi>)
        n1133 = control-ref of="AVS Runtime Settings"() -> (w1418:refnum<vi>)
        n1134 = control-ref of="Current source settings"() -> (w1416:refnum<vi>)
        n1135 = control-ref of="Thermometer"() -> (w1419:refnum<vi>)
        n1136 = control-ref of="PID setup 2"() -> (w1420:refnum<vi>)
        n1137 = control-ref of="Data logging"() -> (w1415:refnum<vi>)
        n1138 = call "Current VIs Parent Directory__ogtk.vi"() -> ("Parent Directory (+ Relative)"=w1407:path)  [unwired: 5 in]
        n1139 = call "File Dialog3"("start path"=w1407, "pattern (all files)"="*.ini") -> ("selected path"=w1405:path)  [unwired: 10 in, 3 out]
        n1140 = Build Array(w1403, w1417, w1418, w1416, w1415, w1419, w1420, w1411, w1410, w1404, w1402, w1401) -> (w1413:refnum<vi>[])
        n1141 = call "Save Load Settings to File by Ref with path.vi"("Array of Cluster References"=w1413, "subkey"="SOFTWARE\\Leiden Cryogenics\\TC" ("subkey 2"), "Action"=enum8{"Load", "Save"}."Save", "error in (no error)"=w1409, "configuration file path"=w1405) -> ("error out"=w1408:errorcluster)  [unwired: 4 in]
      }
      event "Load config": Mouse Up {
        # "Load parameters from the configuration file"
        n1142 = event-data() -> ()  [unwired: 1 in, 8 out]
        n1143 = flat-sequence {
          tunnel: [w1445] -> w1430
          tunnel: w1426 -> [w1440]
          tunnel: [w1435] -> w1421
          tunnel: w1430 -> [w1461]
          tunnel: [w1461] -> w1429
          tunnel: [w1459] -> w1422
          tunnel: w1421 -> [w1459]
          tunnel: [w1466] -> w1428
          tunnel: w1429 -> [w1465]
          tunnel: [w1463] -> w1423
          tunnel: w1422 -> [w1463]
          tunnel: w1428 -> [w1472]
          tunnel: [w1472] -> w1427
          tunnel: [w1470] -> w1424
          tunnel: w1423 -> [w1470]
          tunnel: w1427 -> [w1475]
          tunnel: [w1474] -> w1425
          tunnel: w1424 -> [w1473]
          frame #0 {
            (unwired) T34."HKEY_CURRENT_USER" ("root key (HKEY_LOCAL_MACHINE) 2")
            n1144 = call "Current VIs Parent Directory__ogtk.vi"() -> ("Parent Directory (+ Relative)"=w1437:path)  [unwired: 5 in]
            n1145 = control-ref of="Active"() -> (w1433:refnum<vi>)
            n1146 = control-ref of="Bridge settings"() -> (w1446:refnum<vi>)
            n1147 = control-ref of="AVS Runtime Settings"() -> (w1442:refnum<vi>)
            n1148 = control-ref of="Current source settings"() -> (w1443:refnum<vi>)
            n1149 = control-ref of="Data logging"() -> (w1444:refnum<vi>)
            n1150 = control-ref of="PID setup 2"() -> (w1441:refnum<vi>)
            n1151 = control-ref of="CS Names"() -> (w1439:refnum<vi>)
            n1152 = control-ref of="AVS names"() -> (w1438:refnum<vi>)
            n1153 = control-ref of="CurCalibrations"() -> (w1434:refnum<vi>)
            n1154 = control-ref of="I3 as temp"() -> (w1432:refnum<vi>)
            n1155 = control-ref of="Automode Settings 2"() -> (w1431:refnum<vi>)
            n1156 = call "File Dialog2"("start path"=w1437, "pattern (all files)"="*.ini") -> ("selected path"=w1435:path)  [unwired: 10 in, 3 out]
            n1157 = Build Array(w1433, w1446, w1442, w1443, w1444, w1441, w1439, w1438, w1434, w1432, w1431) -> (w1448:refnum<vi>[])
            n1158 = call "Save Load Settings to File by Ref with path.vi"("Array of Cluster References"=w1448, "subkey"="SOFTWARE\\Leiden Cryogenics\\TC" ("subkey 2"), "Action"=enum8{"Load", "Save"}."Load", "error in (no error)"=w1440, "configuration file path"=w1435) -> ("error out"=w1450:errorcluster)  [unwired: 4 in]
            n1159 = disable-structure shown="Enabled" {
              disable-tunnel: w1450 -> [w1453 w1458]
              disable-tunnel: [w1451 w1458] -> w1445
              frame Disabled {
                n1160 = property on="AVS type" class="Enum (strict)"(error in=w1453) -> (error out=w1454:errorcluster, "Value"=w1456:T30)  [unwired: 1 in, 1 out]
                n1161 = Equal To 0?(x=w1456) -> (x = 0?=w1457:bool)
                n1162 = property on="Address" class="VISAName"(error in=w1454, "Visible"=w1457) -> (error out=w1455:errorcluster)  [unwired: 1 in, 1 out]
                n1163 = Not(x=w1457) -> (.not. x?=w1452:bool)
                n1164 = property on="AVS_SPort" class="VISAName"(error in=w1455, "Visible"=w1452) -> (error out=w1451:errorcluster)  [unwired: 1 in, 1 out]
              }
              frame Enabled {
              }
            }
          }
          frame #1 {
            n1165 = Wait (ms)(milliseconds to wait=250) -> ()  [unwired: 1 out]
          }
          frame #2 {
            n1166 = control-ref of="Thermometer"() -> (w1464:refnum<vi>)
            n1167 = control-ref of="CurCalibrations"() -> (w1462:refnum<vi>)
            n1168 = control-ref of="AVS_CalFolder"() -> (w1468:refnum<vi>)
            n1169 = control-ref of="Select sensor 1"() -> (w1469:refnum<vi>)
            n1170 = control-ref of="Select sensor 1"() -> (w1467:refnum<vi>)
            n1171 = call "ReloadCalibrations.vi"("error in (no error)"=w1465, "Quick convert sensors"=w1467, "CurCalibrations"=w1462, "Calibration files path"=w1468, "Channel1 sensors"=w1469, "Channels list"=w1464) -> ("error out"=w1466:errorcluster)  [unwired: 1 in]
          }
          frame #3 {
            n1172 = Wait (ms)(milliseconds to wait=250) -> ()  [unwired: 1 out]
          }
          frame #4 {
            n1173 = disable-structure shown="Enabled" {
              disable-tunnel: w1475 -> [w1478 w1486]
              disable-tunnel: [w1477 w1484] -> w1474
              disable-tunnel: w1473 -> [w1476 _]
              frame Enabled {
                (unwired) T34."HKEY_CURRENT_USER" ("root key (HKEY_LOCAL_MACHINE) 2")
                n1174 = control-ref of="Thermometer"() -> (w1481:refnum<vi>)
                n1175 = Build Array(w1481) -> (w1480:refnum<vi>[])
                n1176 = call "Save Load Settings to File by Ref with path.vi"("Array of Cluster References"=w1480, "subkey"="SOFTWARE\\Leiden Cryogenics\\TC" ("subkey 2"), "Action"=enum8{"Load", "Save"}."Load", "error in (no error)"=w1478, "configuration file path"=w1476) -> ("error out"=w1477:errorcluster)  [unwired: 4 in]
              }
              frame Disabled {
                n1177 = property on="UpdateCalibrations" class="TypRef (strict)"(error in=w1486) -> (error out=w1485:errorcluster, "Value"=w1487:refnum<user-event>)  [unwired: 1 in, 1 out]
                n1178 = Generate User Event(user event=w1487, event data cluster="" ("event data"), error in=w1485) -> (error out=w1484:errorcluster)  [unwired: 1 in, 1 out]
              }
            }
          }
        }
      }
      event "Parameters": Value Change {
        # "Show parameters menu. (only for zBridge)"
        n1179 = event-data() -> ()  [unwired: 1 in, 6 out]
        n1180 = disable-structure shown="Disabled" {
          frame Enabled {
            w1488 = 0 ("Page")
            n1181 = local read "zDll"() -> (w1489:path)
            n1182 = call "ParamMenu.vi"("Subpage"=w1488, "Page"=w1488, "path in"=w1489) -> ()  [unwired: 7 in, 2 out]
          }
          frame Disabled {
            n1183 = local read "zDll"() -> (w1490:path)
            n1184 = call "zBridgeSettings_1page.vi"("zDll"=w1490) -> ()  [unwired: 10 in, 1 out]
          }
        }
      }
      event "Edit Calibrations": Value Change {
        # "Show calibration files editor. Works with .cal and .cal2 files only"
        n1185 = event-data() -> ("NewVal"=w1499:T4)  [unwired: 1 in, 5 out]
        n1186 = Cluster To Array(cluster=w1499) -> (array=w1498:bool[])
        n1187 = local read "CurCalibrations"() -> (w1493:T18)
        n1188 = Search 1D Array(1D array=w1498, element=TRUE) -> (index of element=w1496:i32)  [unwired: 1 in]
        n1189 = Cluster To Array(cluster=w1493) -> (array=w1492:string[])
        n1190 = Index Array(array=w1492, index=w1496) -> (element=w1495:string)
        n1191 = property on="AVS_CalFolder" class="Path"() -> ("Value"=w1494:path)  [unwired: 2 in, 2 out]
        n1192 = call "Edit Calibration Coefficients.vi"("Calibration Name"=w1495, "Calibration folder"=w1494) -> ("Cancelled?"=w1491:bool)  [unwired: 1 out]
        n1193 = case shown="False" w1491 {
          frame False {
            n1194 = property on="UpdateCalibrations" class="TypRef (strict)"() -> ("Value"=w1501:refnum<user-event>)  [unwired: 2 in, 2 out]
            n1195 = Generate User Event(user event=w1501, event data cluster="" ("event data")) -> ()  [unwired: 2 in, 2 out]
          }
          frame True {
          }
        }
      }
      event "Edit calibration": Value Change {
        # "Show calibration files editor for quick convert R->T. Works with .cal and .cal2 files only"
        n1196 = event-data() -> ()  [unwired: 1 in, 6 out]
        n1197 = property on="Select sensor 1" class="Ring (strict)"() -> ("Strings []"=w1504:string[], "Value"=w1505:u16)  [unwired: 2 in, 2 out]
        n1198 = Index Array(array=w1504, index=w1505) -> (element=w1503:string)
        n1199 = property on="AVS_CalFolder" class="Path"() -> ("Value"=w1506:path)  [unwired: 2 in, 2 out]
        n1200 = call "Edit Calibration Coefficients.vi"("Calibration Name"=w1503, "Calibration folder"=w1506) -> ("Cancelled?"=w1502:bool)  [unwired: 1 out]
        n1201 = case shown="False" w1502 {
          frame False {
            n1202 = property on="UpdateCalibrations" class="TypRef (strict)"() -> ("Value"=w1508:refnum<user-event>)  [unwired: 2 in, 2 out]
            n1203 = Generate User Event(user event=w1508, event data cluster="" ("event data")) -> ()  [unwired: 2 in, 2 out]
          }
          frame True {
          }
        }
      }
      event "zBridge params.AVS Name 0", "zBridge params.AVS Name 1", "zBridge params.AVS Name 2", "zBridge params.AVS Name 3", "zBridge params.AVS Name 4", "zBridge params.AVS Name 5", "zBridge params.AVS Name 6", "zBridge params.AVS Name 7", "zBridge params.AVS Name 8", "zBridge params.AVS Name 9": Mouse Down {
        # "Show parameters menu for the channel by double clicking on \"Channel parameters\". (only for zBridge)"
        n1204 = event-data() -> ("CtlRef"=w1510:refnum<vi>, "Mods.Double Click"=w1509:bool)  [unwired: 1 in, 6 out]
        n1205 = case shown="True" w1509 {
          tunnel: w1510 -> [_ w1513]
          frame False {
          }
          frame True {
            n1206 = control-ref of="zBridge params"() -> (w1515:refnum<vi>)
            n1207 = property class="Clust (strict)"(reference=w1515) -> ("Controls[]"=w1514:refnum<vi>[])  [unwired: 1 in, 2 out]
            n1208 = Search 1D Array(1D array=w1514, element=w1513) -> (index of element=w1511:i32)  [unwired: 1 in]
            n1209 = local read "zDll"() -> (w1516:path)
            n1210 = call "ParamMenu.vi"("Subpage"=w1511, "Page"=0, "path in"=w1516) -> ()  [unwired: 7 in, 2 out]
          }
        }
      }
      event "Active.active Channel 0", "Active.active Channel 1", "Active.active Channel 2", "Active.active Channel 3", "Active.active Channel 4", "Active.active Channel 5", "Active.active Channel 6", "Active.active Channel 7", "Active.active Channel 8", "Active.active Channel 9": Mouse Down {
        # "Switch channels On/Off by double clicking on \"Active\" LED. (only for zBridge and AVS47B)"
        n1211 = event-data() -> ("CtlRef"=w1519:refnum<vi>, "Mods.Double Click"=w1517:bool)  [unwired: 1 in, 6 out]
        n1212 = property on="AVS type" class="Enum (strict)"() -> ("Value"=w1518:T30)  [unwired: 2 in, 2 out]
        n1213 = case shown="True" w1517 {
          tunnel: w1519 -> [_ w1521]
          tunnel: w1518 -> [_ w1525]
          frame False {
          }
          frame True {
            n1214 = control-ref of="Active"() -> (w1524:refnum<vi>)
            n1215 = property class="Clust (strict)"(reference=w1524) -> ("Controls[]"=w1522:refnum<vi>[])  [unwired: 1 in, 2 out]
            n1216 = property class="Bool (strict)"(reference=w1521) -> ("Value"=w1520:bool)  [unwired: 1 in, 2 out]
            n1217 = Search 1D Array(1D array=w1522, element=w1521) -> (index of element=w1523:i32)  [unwired: 1 in]
            n1218 = case shown="\"AVS47B (RS232 interface)\"" w1525 {
              tunnel: w1523 -> [_ w1530 w1531]
              tunnel: w1522 -> [_ w1529 _]
              tunnel: w1520 -> [_ w1526 _]
              frame Default {
              }
              frame "AVS47B (RS232 interface)" {
                n1219 = Index Array(array=w1529, index=w1530) -> (element=w1528:refnum<vi>)
                n1220 = Not(x=w1526) -> (.not. x?=w1527:bool)
                n1221 = property class="Ctl"(reference=w1528, "Value"=w1527) -> ()  [unwired: 1 in, 2 out]
              }
              frame "Impedance Bridge" {
                w1533 = T46."Active" ("Enum")
                # "Invert Active flag"
                n1222 = local read "zDll"() -> (w1536:path)
                n1223 = call "GetByteParam.vi"("ParNo"=w1533, "SetNo"=w1531, "zDll"=w1536) -> ("return type"=w1535:u8)  [unwired: 6 in, 2 out]
                n1224 = Decrement(x=w1535) -> (x-1=w1534:i8)
                n1225 = Absolute Value(x=w1534) -> (abs(x)=w1532:i8)
                n1226 = call "SetByteParam.vi"("SetNo"=w1531, "ParNo"=w1533, "Data"=w1532, "zDll"=w1536) -> ()  [unwired: 6 in, 2 out]
              }
            }
          }
        }
      }
      event "PID setup 2.FB on 2": Value Change {
        n1227 = event-data() -> ("NewVal"=w1537:enum16{"0", "1", "2", "3"})  [unwired: 1 in, 5 out]
        n1228 = property on="ResetPIDloop" class="TypRef (strict)"() -> ("Value"=w1540:refnum<user-event>)  [unwired: 2 in, 2 out]
        n1229 = Generate User Event(user event=w1540, event data cluster="" ("event data")) -> ()  [unwired: 2 in, 2 out]
        n1230 = Index Array(array=string[] ["%#_g uA", "%#_g mK"], index=w1537) -> ()  [unwired: 1 out]
      }
      event "AVS names": Value Change {
        # "Update channel names on the small bottom panel when the names are changed."
        n1231 = event-data() -> ("NewVal"=→"AVS names small":T3)  [unwired: 1 in, 5 out]
      }
      event "I_list": Value Change {
        n1232 = event-data() -> ("NewVal"=w1545:dbl[][])  [unwired: 1 in, 5 out]
        n1233 = local read "I_list_idx"() -> (w1544:i32)
        n1234 = Decrement(x=w1544) -> (x-1=w1543:i32)
        n1235 = Array Size(array=w1545) -> (size(s)=w1547:i32[])
        n1236 = Index Array(array=w1547) -> (element=→"I_list_idx_max":i32)  [unwired: 1 in]
        n1237 = Index Array(array=w1545, index (row)=w1543) -> (element=→"I_list[i]":dbl[])  [unwired: 1 in]
      }
      event "I_list": Shortcut Menu Activation? {
        n1238 = event-data() -> ()  [unwired: 1 in, 7 out]
        n1239 = event-data() -> ()  [unwired: 2 in, 1 out]
      }
      event "I_list": Shortcut Menu Selection (App) {
        n1240 = event-data() -> ("ItemTag"=w1548:string)  [unwired: 1 in, 7 out]
        n1241 = case shown="\"APP_SC_COPY_DATA\"" w1548 {
          frame Default {
          }
          frame "APP_SC_PASTE_DATA" {
            n1242 = invoke class="App" method="Clipboard.Read"() -> ("Read Clipbrd"=w1551:string)  [unwired: 3 in, 2 out]
            n1243 = Spreadsheet String To Array(format string="%d", spreadsheet string=w1551) -> (array=w1549:dbl[][])  [unwired: 2 in]
            n1244 = local write "I_list"(w1549) -> ()
          }
          frame "APP_SC_COPY_DATA" {
            n1245 = local read "I_list"() -> (w1554:dbl[][])
            n1246 = Array To Spreadsheet String(array=w1554, 3:"%d" ("format string")) -> (spreadsheet string=w1552:string)  [unwired: 1 in]
            n1247 = invoke class="App" method="Clipboard.Write"("Param 0"=w1552) -> ()  [unwired: 3 in, 4 out]
          }
        }
      }
      event "I_tofirst": Value Change {
        n1248 = event-data() -> ("OldVal"=w1555:bool)  [unwired: 1 in, 5 out]
        n1249 = local write "I_tofirst"(w1555) -> ()
        n1250 = property on="I_list_idx" class="DigNum (strict)"("Val(Sgnl)"=1 ("Value (Signaling)")) -> ()  [unwired: 2 in, 2 out]
      }
      event "I_next": Value Change {
        n1251 = event-data() -> ("OldVal"=w1557:bool)  [unwired: 1 in, 5 out]
        n1252 = local write "I_next"(w1557) -> ()
        n1253 = local read "I_list_idx"() -> (w1559:i32)
        n1254 = Increment(x=w1559) -> (x+1=w1558:i32)
        n1255 = property on="I_list_idx" class="DigNum (strict)"("Val(Sgnl)"=w1558) -> ()  [unwired: 2 in, 2 out]
      }
      event "I_prev": Value Change {
        n1256 = event-data() -> ("OldVal"=w1560:bool)  [unwired: 1 in, 5 out]
        n1257 = local write "I_prev"(w1560) -> ()
        n1258 = local read "I_list_idx"() -> (w1562:i32)
        n1259 = Decrement(x=w1562) -> (x-1=w1561:i32)
        n1260 = property on="I_list_idx" class="DigNum (strict)"("Val(Sgnl)"=w1561) -> ()  [unwired: 2 in, 2 out]
      }
      event "I_Clear": Value Change {
        n1261 = event-data() -> ()  [unwired: 1 in, 6 out]
        n1262 = flat-sequence {
          frame #0 {
            n1263 = local write "I_list"(dbl[][] [] ("I_list")) -> ()
          }
          frame #1 {
            n1264 = property on="I_tofirst" class="Bool (strict)"("Val(Sgnl)"=TRUE ("Value (Signaling)")) -> ()  [unwired: 2 in, 2 out]
          }
        }
      }
      event "I_list_idx": Value Change {
        w1586 = 10  # Lines to scroll
        n1265 = event-data() -> ("NewVal"=w1569:i32)  [unwired: 1 in, 5 out]
        n1266 = Array Size(array="I_list") -> (size(s)=w1572:i32[])
        n1267 = Index Array(array=w1572) -> (element=w1570:i32)  [unwired: 1 in]
        n1268 = Get Date/Time In Seconds() -> (seconds since 1Jan1904=w1566:timestamp)
        n1269 = local write "I_list_idx_max"(w1570) -> ()
        n1270 = To Double Precision Float(number=w1566) -> (double precision float=w1565:dbl)
        n1271 = local write "Time Old"(w1565) -> ()
        n1272 = In Range and Coerce(upper limit=w1570, x=w1569, lower limit=1) -> (coerced(x)=w1567:i32)  [unwired: 1 out]
        "I_list_idx" <- w1567
        n1273 = Decrement(x=w1567) -> (x-1=w1568:i32)
        n1274 = Initialize Array(FALSE, w1586) -> (w1587:bool[])
        n1275 = Index Array(array="I_list", index (row)=w1568) -> (element=w1589:dbl[])  [unwired: 1 in]
        n1276 = local write "I_list[i]"(w1589) -> ()
        n1277 = Subtract(x=w1568, y=w1586) -> (x-y=w1576:i32)
        n1278 = Increment(x=w1576) -> (x+1=w1575:i32)
        n1279 = Decrement(x=w1586) -> (x-1=w1584:i32)
        n1280 = In Range and Coerce(upper limit=inf, x=w1575, lower limit=0) -> (coerced(x)=w1574:dbl)  [unwired: 1 out]
        n1281 = In Range and Coerce(upper limit=w1584, x=w1568, lower limit=0) -> (coerced(x)=w1581:i32)  [unwired: 1 out]
        n1282 = control-ref of="I_list"() -> (w1579:refnum<vi>)
        n1283 = Build Array(w1574, 0 ("element")) -> (w1580:dbl[])
        n1284 = Replace Array Subset(array=w1587, new element=TRUE ("new element/subarray"), index=w1581) -> (→"I_selection":bool[])
        n1285 = property class="Arr (strict)"(reference=w1579, "Index Values"=w1580) -> ()  [unwired: 1 in, 2 out]
      }
      event "Save to file": Value Change {
        n1286 = event-data() -> ()  [unwired: 1 in, 6 out]
        n1287 = call "File Dialog6"() -> ("selected path"=w1592:path, "cancelled"=w1591:bool)  [unwired: 12 in, 2 out]
        n1288 = case shown="False" w1591 {
          tunnel: w1592 -> [w1593 _]
          frame False {
            n1289 = local read "I_list"() -> (w1595:dbl[][])
            n1290 = call <vilib>:"Write To Spreadsheet File (DBL).vi"("format (%.3f)"="%.1f", "2D data"=w1595, "file path (dialog if empty)"=w1593) -> ()  [unwired: 5 in, 1 out]
          }
          frame True {
          }
        }
      }
      event "Load from file": Value Change {
        n1291 = event-data() -> ()  [unwired: 1 in, 6 out]
        n1292 = call "File Dialog5"() -> ("selected path"=w1596:path, "cancelled"=w1597:bool)  [unwired: 12 in, 2 out]
        n1293 = case shown="False" w1597 {
          tunnel: w1596 -> [w1598 _]
          frame False {
            n1294 = call <vilib>:"Read From Spreadsheet File (DBL).vi"("file path (dialog if empty)"=w1598) -> ("all rows"=w1599:dbl[][])  [unwired: 6 in, 4 out]
            n1295 = local write "I_list"(w1599) -> ()
          }
          frame True {
          }
        }
      }
      event "Write to log": Value Change {
        n1296 = event-data() -> ()  [unwired: 1 in, 6 out]
        n1297 = property on="TempStabilized" class="TypRef (strict)"() -> ("Value"=w1601:refnum<user-event>)  [unwired: 2 in, 2 out]
        n1298 = Generate User Event(user event=w1601, event data cluster=FALSE ("event data")) -> ()  [unwired: 2 in, 2 out]
      }
    }
    "General" <- w21
  }
  n1299 = while {
    stop <- w1602 stop-if-true
    # "Main loop"
    n1300 = property on="start 2" class="Bool (strict)"() -> ("Value"=w1604:bool)  [unwired: 2 in, 2 out]
    n1301 = Wait (ms)(milliseconds to wait=u32 200) -> ()  [unwired: 1 out]
    n1302 = case shown="True" w1604 {
      frame False {
        n1303 = Wait (ms)(milliseconds to wait=u32 250) -> ()  [unwired: 1 out]
      }
      frame True {
        n1304 = while {
          i -> [w1615]
          stop <- "Stop" stop-if-true
          # "AVS/zBridge read-out"
          n1305 = case shown="False" "Pause" {
            tunnel: w1615 -> [w1622 _]
            frame False {
              # "for the first measurement set Stab.Time=12 s to do autoranging"
              n1306 = property on="AVS Runtime Settings" class="Clust (strict)"() -> ("Value"=w1639:T12)  [unwired: 2 in, 2 out]
              n1307 = Unbundle By Name(w1639) -> ("Stabilisation Delay"=w1630:dbl, "Averages"=w1623:u16, "Last Channel"=w1638:i8, "Read AVS channels from"=w1637:i8)
              n1308 = local read "Active"() -> (w1620:T10)
              n1309 = property on="AVS type" class="Enum (strict)"() -> ("Value"=w1635:T30)  [unwired: 2 in, 2 out]
              n1310 = call "Split Exc&Range.vi"("Excitations 2"="Exc&Ranges") -> ("Excitations"=w1627:T13, "Ranges"=w1621:T47)  [unwired: 4 in]
              n1311 = property on="AVS VISA session" class="VISAName"() -> ("Value"=w1636:refnum<visa-resource-name>)  [unwired: 2 in, 2 out]
              n1312 = Cluster To Array(cluster=w1620) -> (array=w1619:bool[])
              n1313 = call "If First Iteration.vi"("Iteration"=w1622, "Value In"=w1630, "Default"=12.0) -> ("Value Out"=w1629:dbl)
              n1314 = case shown="\"AVS47B (RS232 interface)\"" w1635 {
                tunnel: w1636 -> [w1649 w1660 _ _ _]
                tunnel: w1629 -> [w1645 w1663 w1669 _ _]
                tunnel: w1623 -> [w1646 w1662 _ _ _]
                tunnel: w1638 -> [w1647 w1658 _ _ _]
                tunnel: w1637 -> [w1648 w1659 _ _ _]
                tunnel: w1627 -> [w1650 w1654 _ _ _]
                tunnel: [w1641 w1653 errorcluster {"status"=FALSE, "code"=0, "source"=""} ("error out") w1688 errorcluster {"status"=FALSE, "code"=0, "source"=""} ("error out")] -> w1626
                tunnel: w1621 -> [w1643 w1656 w1670 w1689 w1693]
                tunnel: "Autorange" -> [w1644 w1657 _ _ _]
                tunnel: [w1642 w1655 w1670 w1689 w1693] -> w1618
                tunnel: [w1640 w1652 w1668 w1680 dbl[] [] ("Data array")] -> w1624
                tunnel: w1619 -> [_ w1651 _ _ _]
                frame "AVS47A (GPIB interface)", Default {
                  # "AVS 47 (GPIB)"
                  n1315 = call "AVS_do_single_scan.vi"("AVS Port"=w1649, "Stabilization Delay"=w1645, "Autorange"=w1644, "Number of Averages"=w1646, "Last Channel"=w1647, "First Channel"=w1648, "Excitations"=w1650, "Ranges"=w1643) -> ("error out"=w1641:errorcluster, "R"=w1640:dbl[], "Ranges"=w1642:T48)  [unwired: 3 in, 2 out]
                }
                frame "AVS47B (RS232 interface)" {
                  # "AVS 47B (RS232)"
                  n1316 = Type Cast(type=refnum<visa-resource-name> refnum ("dup VISA session"), x=w1660) -> (*(type *) &x=w1664:refnum<visa-resource-name>)
                  n1317 = call "Scanner.vi"("STABILIZATION  DELAY"=w1663, "FIRST CH TO SCAN"=w1659, "LAST CH TO SCAN"=w1658, "Autorange"=w1657, "AVERAGE COUNT"=w1662, "Excitation"=w1654, "Range"=w1656, "VISA resource"=w1664, "array"=w1651) -> ("RI"=w1652:dbl[], "Range out"=w1655:T49, "error out 2"=w1653:errorcluster)  [unwired: 1 in, 3 out]
                }
                frame "AVS Emulation" {
                  n1318 = local read "I 2"() -> (w1666:dbl[])
                  n1319 = Multiply(x=w1669, y=u32 1000 ("milliseconds to wait")) -> (x*y=w1678:dbl)
                  n1320 = Wait (ms)(milliseconds to wait=w1678) -> ()  [unwired: 1 out]
                  n1321 = Index Array(array=w1666, index=3) -> ()  [unwired: 1 out]
                  n1322 = property on="I" class="Arr (strict)"() -> ("Value"=w1677:dbl[])  [unwired: 2 in, 2 out]
                  n1323 = Multiply(x=1000.0, y=w1677) -> (x*y=w1672:dbl[])
                  n1324 = Index Array(array=w1672, index #1=2 ("index"), index #2=3 ("index")) -> (element #1=w1673:dbl, element #2=w1674:dbl)
                  n1325 = call "AVS Emulate.vi"("I_mc"=w1674, "I_still"=w1673, "Sampling time"=w1669) -> ("R"=w1668:dbl[])  [unwired: 1 out]
                }
                frame "Impedance Bridge" {
                  n1326 = local read "Bridge status"() -> (w1681:errorcluster)
                  n1327 = local read "zDll"() -> (w1690:path)
                  n1328 = call "Read Data from Single Channel.vi"("zDll"=w1690, "error in (no error)"=w1681) -> ("Unit"=→"Unit":string, "Error code"=→"Error code":u8, "Set number"=w1686:u8, "Scan parameters/Error"=→"zBridge params/Error":string, "Value"=w1685:dbl, "error out"=w1688:errorcluster)
                  "zBridge set nr." <- w1686
                  n1329 = Replace Array Subset(array="Data array", new element=w1685, index=w1686) -> (w1680:dbl[])
                }
                frame "Disabled" {
                }
              }
              "Bridge status" <- w1626
              n1330 = property on="Delay" class="DigNum (strict)"() -> ("Value"=w1634:u32)  [unwired: 2 in, 2 out]
              n1331 = property on="Data array" class="Arr (strict)"("Val(Sgnl)"=w1624) -> ()  [unwired: 2 in, 2 out]
              n1332 = property on="Ranges" class="Clust (strict)"("Val(Sgnl)"=w1618) -> ()  [unwired: 2 in, 2 out]
              n1333 = Multiply(x=u32 1000, y=w1634) -> (x*y=w1633:u32)
              n1334 = Wait (ms)(milliseconds to wait=w1633) -> ()  [unwired: 1 out]
            }
            frame True {
            }
          }
        }
        n1335 = while {
          stop <- w1695 stop-if-true
          (unwired) errorcluster {"status"=FALSE, "code"=0, "source"=""} ("Value")
          # "Current source control"
          n1336 = property on="CS status" class="Clust (strict)"() -> ("Value"=w1694:errorcluster)  [unwired: 2 in, 2 out]
          n1337 = stacked-sequence {
            seq-local: [w1723 _ _ _] -> [_ w1732 _ _]
            seq-local: [w1722 _ _ _] -> [_ w1731 _ _]
            seq-local: [_ w1732 _ _] -> [_ _ w1742 _]
            seq-local: [_ w1730 _ _] -> [_ _ w1741 _]
            tunnel: w1694 -> [w1721 _ _ _]
            frame #0 {
              # "Write 0 instead of the actual \ncurrent value to log if there \nis no current flow."
              # "Read current CS status"
              n1338 = local read "CS ref"() -> (w1711:refnum<class "CS.lvclass">)
              n1339 = property on="TCS port" class="Ring (strict)" props=["Value"]() -> ()  [unwired: 2 in, 3 out]
              n1340 = call-dynamic "Read.vi"("CS in"=w1711, "error in (no error)"=w1721, "Optional"=FALSE) -> ("CS out"=w1723:refnum<class "CS.lvclass">, "I0"=w1714:T50, "I1"=w1715:T50, "I2"=w1716:T50, "I3"=w1717:T50, "error out"=w1722:errorcluster)  [unwired: 11 in]
              n1341 = Unbundle By Name(w1714) -> ("Current (string)"=w1709:string, "I?"=w1708:bool)
              n1342 = Unbundle By Name(w1715) -> ("Current (string)"=w1724:string, "I?"=w1707:bool)
              "Current1flow" <- w1707
              n1343 = Unbundle By Name(w1716) -> ("Current (string)"=w1712:string, "I?"=w1706:bool)
              n1344 = Unbundle By Name(w1717) -> ("Current (string)"=w1725:string, "I?"=w1705:bool)
              n1345 = call "CS Data Converter.vi"("CS Data"=w1714) -> ("CS Indicator"=→"Ch0 -":T51)
              n1346 = call "CS Data Converter.vi"("CS Data"=w1715) -> ("CS Indicator"=→"Chn 1":T51)
              n1347 = call "CS Data Converter.vi"("CS Data"=w1716) -> ("CS Indicator"=→"Chn 2":T51)
              n1348 = call "CS Data Converter.vi"("CS Data"=w1717) -> ("CS Indicator"=→"Chn 3":T51)
              n1349 = Fract/Exp String To Number(string=w1709) -> (number=w1713:dbl)  [unwired: 3 in, 1 out]
              n1350 = Fract/Exp String To Number(string=w1724) -> (number=w1720:dbl)  [unwired: 3 in, 1 out]
              n1351 = Fract/Exp String To Number(string=w1712) -> (number=w1719:dbl)  [unwired: 3 in, 1 out]
              n1352 = Fract/Exp String To Number(string=w1725) -> (number=w1718:dbl)  [unwired: 3 in, 1 out]
              n1353 = Build Array(w1708, w1707, w1706, w1705) -> (w1704:bool[])
              n1354 = Not(x=w1704) -> (.not. x?=w1700:bool[])
              n1355 = Build Array(w1713, w1720, w1719, w1718) -> (w1703:dbl[])
              "I" <- w1703
              n1356 = for {
                tunnel: w1700 -> [w1729] mode=indexing
                tunnel: w1703 -> [w1728] mode=indexing
                tunnel: dbl[] [0.0, 0.0, 0.0, 0.0] ("t") -> [w1727] mode=indexing
                tunnel: [w1726] -> w1701 mode=indexing
                n1357 = Select(t=w1727, s=w1729, f=w1728) -> (s? t:f=w1726:dbl)
              }
              "All I" <- w1701
            }
            frame #1 {
              n1358 = Wait (ms)(milliseconds to wait=100) -> ()  [unwired: 1 out]
              n1359 = call <vilib>:"Clear Errors.vi"("error in (no error)"=w1731) -> ("error out"=w1730:errorcluster)  [unwired: 6 in]
            }
            frame #2 {
              # "Only send data to CS if\nnew value was entered"
              # "Set CS status"
              n1360 = call "CS OnOff & Gated and Current & Range.vi"("I in"="I0") -> ("OnOff & Gated"=w1753:T52, "Current & Range"=w1738:T53, "I out"=w1746:T54)  [unwired: 2 in]
              n1361 = call "CS OnOff & Gated and Current & Range.vi"("I in"="I1") -> ("OnOff & Gated"=w1752:T52, "Current & Range"=w1737:T53, "I out"=w1743:T54)  [unwired: 2 in]
              n1362 = call "CS OnOff & Gated and Current & Range.vi"("I in"="I2") -> ("OnOff & Gated"=w1749:T52, "Current & Range"=w1736:T53, "I out"=w1744:T54)  [unwired: 2 in]
              n1363 = call "CS OnOff & Gated and Current & Range.vi"("I in"="I3") -> ("OnOff & Gated"=w1748:T52, "Current & Range"=w1735:T53, "I out"=w1745:T54)  [unwired: 2 in]
              n1364 = local write "I0"(w1746) -> ()
              n1365 = local write "I1"(w1743) -> ()
              n1366 = local write "I2"(w1744) -> ()
              n1367 = local write "I3"(w1745) -> ()
              n1368 = local read "I 2"() -> (w1734:dbl[])
              n1369 = Equal To 0?(x="Mode") -> (x = 0?=w1739:bool)
              n1370 = call "CS_set_channels.vi"("CS in"=w1742, "Current & Range0"=w1738, "Current & Range1"=w1737, "Current & Range 2"=w1736, "Current & Range3"=w1735, "error out"=w1741, "I 2"=w1734, "Auto?"=w1739) -> ("CS.lvclass out"=w1758:refnum<class "CS.lvclass">, "Current Changed?"=w1755:bool, "error out 2"=w1759:errorcluster)  [unwired: 9 in]
              n1371 = call-dynamic "Set Mode.vi"("CS.lvclass in"=w1758, "On&G 0"=w1753, "On&G 1"=w1752, "On&G 2"=w1749, "On&G 3"=w1748, "error in (no error)"=w1759) -> ("CS.lvclass out"=w1756:refnum<class "CS.lvclass">, "error out"=w1757:errorcluster)  [unwired: 12 in]
              n1372 = case shown="True" w1755 {
                selector: w1755 -> [_ w1760]
                frame False {
                }
                frame True {
                  n1373 = property on="Currents changed" class="Bool (strict)"("Val(Sgnl)"=w1760) -> ()  [unwired: 2 in, 2 out]
                }
              }
              n1374 = local write "CS ref"(w1756) -> ()
              n1375 = property on="CS status" class="Clust (strict)"("Value"=w1757) -> ()  [unwired: 2 in, 2 out]
            }
            frame #3 {
              n1376 = Wait (ms)(milliseconds to wait=100) -> ()  [unwired: 1 out]
            }
          }
          n1377 = local read "Stop"() -> (w1695:bool)
        }
        n1378 = while {
          stop <- w1608 stop-if-true
          # "zBridge status read-out"
          n1379 = property on="AVS type" class="Enum (strict)"() -> ("Value"=w1606:T30)  [unwired: 2 in, 2 out]
          n1380 = case shown="\"Impedance Bridge\"" w1606 {
            frame Default {
            }
            frame "Impedance Bridge" {
              n1381 = local read "Bridge status"() -> (w1612:errorcluster)
              n1382 = local read "zDll"() -> (w1613:path)
              n1383 = call "ScanStatus.vi"("error in (no error)"=w1612, "zDll"=w1613) -> ("error out"=w1611:errorcluster, "Status"=w1609:i32, "Channel"=w1610:i32)  [unwired: 7 in]
              n1384 = call "zBridge Format Status.vi"("Status"=w1609, "Channel"=w1610) -> ("Status"=→"Status":T55)  [unwired: 2 in]
              n1385 = local write "Bridge status"(w1611) -> ()
            }
          }
          n1386 = Wait (ms)(milliseconds to wait=u32 200) -> ()  [unwired: 1 out]
          n1387 = local read "Stop"() -> (w1608:bool)
        }
      }
    }
    n1388 = local read "Stop"() -> (w1602:bool)
  }
  n1389 = disable-structure shown="Disabled" {
    frame Disabled {
      w1763 = string[] ["Paste Data from Clipboard"] ("item names")
      (unwired) enum32{"Page 1"}."Page 1" ("Tab Control 4")
      n1390 = Insert Menu Items(4:4, 7:w1763, 8:w1763) -> (9:w1764:refnum<k9>)  [unwired: 2 in, 3 out]
      n1391 = property on="I3" class="DigNum (strict)"() -> ("Value"=w1772:dbl)  [unwired: 2 in, 2 out]
      n1392 = property on="ON" class="Boolean (strict)"() -> ("Value"=w1771:bool)  [unwired: 2 in, 2 out]
      n1393 = control-ref of="Active"() -> ()  [unwired: 1 out]
      n1394 = local write "I0"(w1772) -> ()
      n1395 = Exclusive Or(1:w1771, 2:TRUE ("x")) -> (0:w1770:bool)
      n1396 = property on="Toggle ON/OFF" class="Bool (strict)"("Value"=w1770) -> ()  [unwired: 2 in, 2 out]
      n1397 = control-ref of="I_list"() -> (w1766:refnum<vi>)
      n1398 = property on="ResetPIDloop" class="TypRef (strict)"() -> ("Value"=w1777:refnum<user-event>)  [unwired: 2 in, 2 out]
      n1399 = property class="Arr (strict)"(reference=w1766) -> ("Index Values"=w1767:u32[])  [unwired: 1 in, 2 out]
      n1400 = Generate User Event(user event=w1777, event data cluster="" ("event data")) -> ()  [unwired: 2 in, 2 out]
      n1401 = Index Array(array=w1767) -> (element=w1768:u32)  [unwired: 1 in]
      n1402 = property on="Tab Control 2" class="TabCtl (strict)"() -> ("Pages"=w1773:refnum<vi>[])  [unwired: 2 in, 2 out]
      n1403 = property on="I_list_idx" class="DigNum (strict)"("Val(Sgnl)"=w1768) -> ()  [unwired: 2 in, 2 out]
      n1404 = Index Array(array=w1773, index=1) -> (element=w1774:refnum<vi>)
      n1405 = Generate User Event(event data cluster="" ("event data")) -> ()  [unwired: 3 in, 2 out]
      n1406 = property class="Page"(reference=w1774, "PageVis"=TRUE ("Page Visible")) -> ()  [unwired: 1 in, 2 out]
      n1407 = local read "Error"() -> ()  [unwired: 1 out]
      n1408 = local read "Int"() -> ()  [unwired: 1 out]
      n1409 = local read "I0"() -> ()  [unwired: 1 out]
    }
    frame Enabled {
    }
  }
  n1410 = control-ref of="Automode Settings 2"() -> ()  [unwired: 1 out]
  n1411 = property on="I3_SP" class="DigNum (strict)" props=["Value"]() -> ()  [unwired: 2 in, 3 out]
